vi "VC100_Facility_Control_V1.0.vi"() -> ()   [LabVIEW 2024]
uses:
  Small_Facility_Control/Current_Facility_State.ctl
  Small_Facility_Control/Facility_State.ctl
  <vilib>/Platform/TimedLoop/XDataNode/timing_clust.ctl
  <vilib>/Platform/TimedLoop/XDataNode/nitl_modes.ctl
  <vilib>/Platform/TimedLoop/XDataNode/wakeup.ctl
  <vilib>/DAQmx/read.llb/DAQmx Read (Analog Wfm 1Chan 1Samp).vi
  <vilib>/DAQmx/read.llb/DAQmx Read (Digital Bool 1Line 1Point).vi
  <vilib>/DAQmx/read.llb/DAQmx Read (Analog 1D Wfm NChan NSamp).vi
  <vilib>/DAQmx/read.llb/DAQmx Read (Digital 1D Bool NChan 1Samp 1Line).vi
  <vilib>/Analysis/baseanly.llb/Mean (DBL).vi
  92da63ed-27f3-4d29-b829-85232dab9436.vi
  dc02d6ae-0d69-4f83-ad2b-62eea8acb765.vi
  5e56a759-01b7-43ee-a6c9-aa4e2b3cae4c.vi
  a7228664-7861-4e48-9f8d-e2306638d1d9.vi
  <vilib>/DAQmx/write.llb/DAQmx Write (Digital 1D Bool NChan 1Samp 1Line).vi
  <vilib>/DAQmx/write.llb/DAQmx Write (Digital Bool 1Line 1Point).vi
  <instrlib>/U1250 Series Multimeter Device Driver/Public/Configure/Low Level/DC Voltage Configuration.vi
  <vilib>/DAQmx/create/channels.llb/DAQmx Create Channel (AI-Voltage-Basic).vi
  <vilib>/DAQmx/miscellaneous.llb/DAQmx Fill In Error Info.vi
  <vilib>/DAQmx/create/channels.llb/DAQmx Create Channel (DO-Digital Output).vi
  <vilib>/DAQmx/create/channels.llb/DAQmx Create Channel (DI-Digital Input).vi
  <vilib>/DAQmx/configure/timing.llb/DAQmx Timing (Sample Clock).vi
  <vilib>/express/express shared/transition.llb/Dynamic To Waveform Array.vi
  <vilib>/express/express signal manip/GetorSetDDTAttributes/Set DDT Attributes/SetT0.vi
  <vilib>/express/express signal manip/GetorSetDDTAttributes/Set DDT Attributes/sub Set StartTimeStamp.vi
  <vilib>/express/express shared/transition.llb/Waveform Array To Dynamic.vi
  <vilib>/Utility/file.llb/Write Delimited Spreadsheet (string).vi
  <instrlib>/U1250 Series Multimeter Device Driver/Controls/Voltage Range.ctl
  <vilib>/platform/TimedLoop/XDataNode/XDataNode.xnode
  <vilib>/express/express signal manip/GetorSetDDTAttributes/Set DDT Attributes/Set DDT Properties.xnode
  <vilib>/express/express signal manip/GetorSetDDTAttributes/Get DDT Attributes/Get DDT Properties.xnode
  <resource>/objmgr/daqmx.rc
  <instrlib>/U1250 Series Multimeter Device Driver/U1250 Series Digital Multimeter.lvlib
  <vilib>/express/express signal manip/GetorSetDDTAttributes/Set DDT Attributes/Set DDT Attributes.lvlib
  <vilib>/Platform/TimedLoop/XDataNode/XDNodeRunTimeDep.lvlib
  <vilib>/Analysis/NI_AALBase.lvlib
panel:
  out "Low Compressor Pressure!":bool
  out "Turbo on Threshold (torr) 3":dbl=0.08
  out "Compressor Pressure (Bar)":dbl=627.9033934565941 format="%_3f"
  in  "Turbo slowing Threshold (%)":dbl=50.0 format="%#_13g"
  out "Use Ecodry As Primary?":bool=TRUE
  out "Ecodry Speed":string="0"
  out "Turbo 2 Speed":string="0"
  out "Turbo 3 Standby?":bool
  out "Turbo 2 Standby?":bool
  out "Turbo 2 Motor Read":bool
  out "Turbo_2_Motor_Sys_Cmd":bool
  out "Numeric 3":dbl
  out "Numeric 2":dbl
  out "New_State? 2":bool
  out "appended array":string[][](array[string])
  out "New log 3":string
  out "New log 2":string
  out "output array":string[][](array[string])
  out "New log":string
  out "New_State?":bool
  out "Sub_state_iteration":i32
  out "DAQ_Name 2":string="cDAQ1"
  out "Turbo on Threshold (torr)":dbl=0.08
  out "Elapsed Time (s)":dbl
  in  "Turbo on Threshold (torr) 2":dbl=0.25 format="%#_13g"
  out "WRG (torr)":dbl=nan format="%_3e"
  in  "Turbo_Reset_Cmd":bool
  in  "Turbo_3_Motor_User_Cmd":bool
  in  "Turbo_2_Motor_User_Cmd":bool
  in  "Turbo_1_Motor_User_Cmd":bool
  in  "Chiller_User_Cmd":bool
  in  "Primary_User_Cmd":bool
  in  "Valve_Gate_3_User_Cmd":bool
  in  "Valve_Gate_2_User_Cmd":bool
  in  "Valve_Gate_1_User_Cmd":bool
  in  "Valve_Vent_User_Cmd":bool
  in  "Valve_Bypass_User_Cmd":bool
  in  "Valve_Turbo_3_User_Cmd":bool
  in  "Valve_Turbo_2_User_Cmd":bool
  out "Turbo 3 Valve Error?":bool
  out "Turbo 2 Valve Error?":bool
  out "Bypass Valve Error?":bool
  out "Gate 3 Valve Error?":bool
  out "Gate 2 Valve Error?":bool
  out "Gate 1 Valve Error?":bool
  in  "Valve_Turbo_1_User_Cmd":bool
  out "Turbo 1 Valve Error?":bool
  out "Index_of_working_turbo":i32
  out "Which_Turbos_used?":bool[](array[boolean])
  out "Valve_Gate_3_Sys_Cmd":bool
  out "Valve_Gate_2_Sys_Cmd":bool
  out "Valve_Turbo_3_Sys_Cmd":bool
  out "Valve_Turbo_2_Sys_Cmd":bool
  out "Turbo 3 Gauge":dbl=627.9033934565941 format="%_3e"
  out "Turbo 2 Gauge":dbl=627.9033934565941 format="%_3e"
  out "Turbo 3 Speed":string="0"
  out "Turbo 3 Status":string="Turbo Off"
  out "Turbo 2 Status":string="Turbo Off"
  out "Turbo 3 Status Color":u32(colorbox)=12632256
  out "Turbo 2 Status Color":u32(colorbox)=12632256
  out "Gate 3 Valve":bool
  out "Gate 2 Valve":bool
  out "Turbo 3 Valve":bool
  out "Turbo 2 Valve":bool
  in  "Change to Auto":bool
  out "Measurement":dbl format="%#_8f"
  in  "ON/OFF":bool
  in  "DMM VISA resource name COM4":refnum<visa-resource-name>="COM4"
  in  "use DMM?":bool
  in  "samples per channel":i32=200
  in  "rate":dbl=1000.0 format="%#_13g"
  out "Current Time/date":string
  out "String 3":string
  out "Vent Time (s) 2":dbl caption="Elapsed Time (s)"
  out "Numeric":dbl
  out "Turbo 1 Gauge":dbl=627.9033934565941 format="%_3e"
  out "Log":string
  out "Gate 1 Valve":bool
  out "Valve_Gate_1_Sys_Cmd":bool
  out "Vent Valve Error?":bool
  out "Primary Status":u32(colorbox)=12632256
  out "Bypass Valve":bool
  out "Vent Valve":bool
  out "Primary Pump Status":string="Primary Pump is Off"
  out "Wide Range Gauge Pressure":dbl=nan format="%_3e"
  out "Foreline Gauge":dbl=627.9033934565941 format="%_3e"
  out "Chiller Status":string="Chiller is Off"
  out "Turbo 1 Status":string="Turbo Off"
  out "Chiller Status 2":u32(colorbox)=12632256
  out "Turbo 1 Status Color":u32(colorbox)=12632256
  in  "stop":bool
  out "error out":errorcluster
  out "Control Level":enum32{"Admin", "Debug", "Automatic"}(tab)=enum."Automatic"
  in  "Fake_Chiller_Read":bool
  in  "Fake_Turbo_1_Pressure_mBar":dbl=0.0001 format="%_3e"
  in  "Fake_Primary_Pump_Read":bool
  in  "Fake_Valve_Turbo_Read":bool
  in  "Fake_Valve_Bypass_Read":bool
  in  "Fake_Valve_Vent_Read":bool
  in  "Use fake values?":bool=TRUE
  in  "Fake_Fore_Pressure_mBar":dbl=0.001 format="%_3e"
  in  "Fake_Valve_Gate_Read":bool
  in  "Fake_WRG_Pressure_mBar":dbl=1e-05 format="%_3e"
  in  "Turbo Engage time":timestamp=timestamp(3820287600 s since 1904-01-01)
  out "Current Facility State":T1
  out "Target Facility State":T1
  out "Tab Control":T2(tab)=enum."Holding at Rough"
  in  "Pump to High Vac":bool
  in  "Pump to Rough":bool
  in  "Overnight Pump":bool
  in  "Vent":bool
  in  "Shut Off once rough 2":bool
  in  "Vent 2":bool
  in  "Shut Off":bool
  in  "Overnight Pump 3":bool
  in  "Pump to Rough 2":bool
  in  "Pump to High Vac 2":bool
  in  "Shut Off once rough":bool
  in  "Vent 4":bool
  in  "Pump to Rough 3":bool
  in  "Pump to High Vac 3":bool
  in  "Vent 5":bool
  in  "Shutdown":bool
  in  "Pump to Rough 4":bool
  in  "Overnight Pump 2":bool
  in  "Vent and shutdonw":bool
  in  "Shutdown Now":bool
  in  "Pump to Hi vac":bool
  in  "Overnight Pump 5":bool
  in  "Pump to Rough 5":bool
  in  "Shutdown After Vent":bool
  in  "Pump to High Vac 4":bool
  in  "Vent":bool
  in  "change_to_admin_mode":bool
  out "Countdown":string
  in  "Clear error?":bool
  out "Running":bool
  out "Waveform Chart 2":waveform(dbl)[](graph)=[{"t0"=timestamp(3754409348.7178025 s since 1904-01-01), "dt"=0.1, "Y"=array[1789 elements]}, {"t0"=timestamp(3754409348.7178025 s since 1904-01-01), "dt"=0.1, "Y"=array[1789 elements]}, {"t0"=timestamp(3754409348.7178025 s since 1904-01-01), "dt"=0.1, "Y"=array[1789 elements]}, {"t0"=timestamp(3754409348.7178025 s since 1904-01-01), "dt"=0.1, "Y"=array[1789 elements]}, {"t0"=timestamp(3754409348.7178025 s since 1904-01-01), "dt"=0.1, "Y"=array[1789 elements]}, {"t0"=timestamp(3754409348.7178025 s since 1904-01-01), "dt"=0.1, "Y"=array[1789 elements]}, {"t0"=timestamp(3754409348.7178025 s since 1904-01-01), "dt"=0.1, "Y"=array[1789 elements]}, {"t0"=timestamp(3754409348.7178025 s since 1904-01-01), "dt"=0.1, "Y"=array[1789 elements]}]
  out "Turbo 3 Motor Read":bool
  out "Primary_Pump_Read":bool
  out "Turbo_3_Motor_Sys_Cmd":bool
  out "Chiller_Sys_Cmd":bool
  out "Valve_Vent_Sys_Cmd":bool
  out "Valve_Bypass_Sys_Cmd":bool
  out "Valve_Turbo_1_Sys_Cmd":bool
  out "Use_real_Values?":bool=TRUE
  out "Primary_Sys_Cmd":bool
  out "DAQ_Name":string="cDAQ1"
  out "Turbo 1 Valve":bool
  out "String 4":string
  # "mBar"
  # "Pressure (mBar)"
  # "Speed (%):"
  # "Speed (%):"
  # "mBar"
  # "mBar"
  # "mBar"
  # "On"
  # "Status"
  # "mBar"
  # "Off"
  # "Admin Mode Enabled"
  # "Please Wait..."
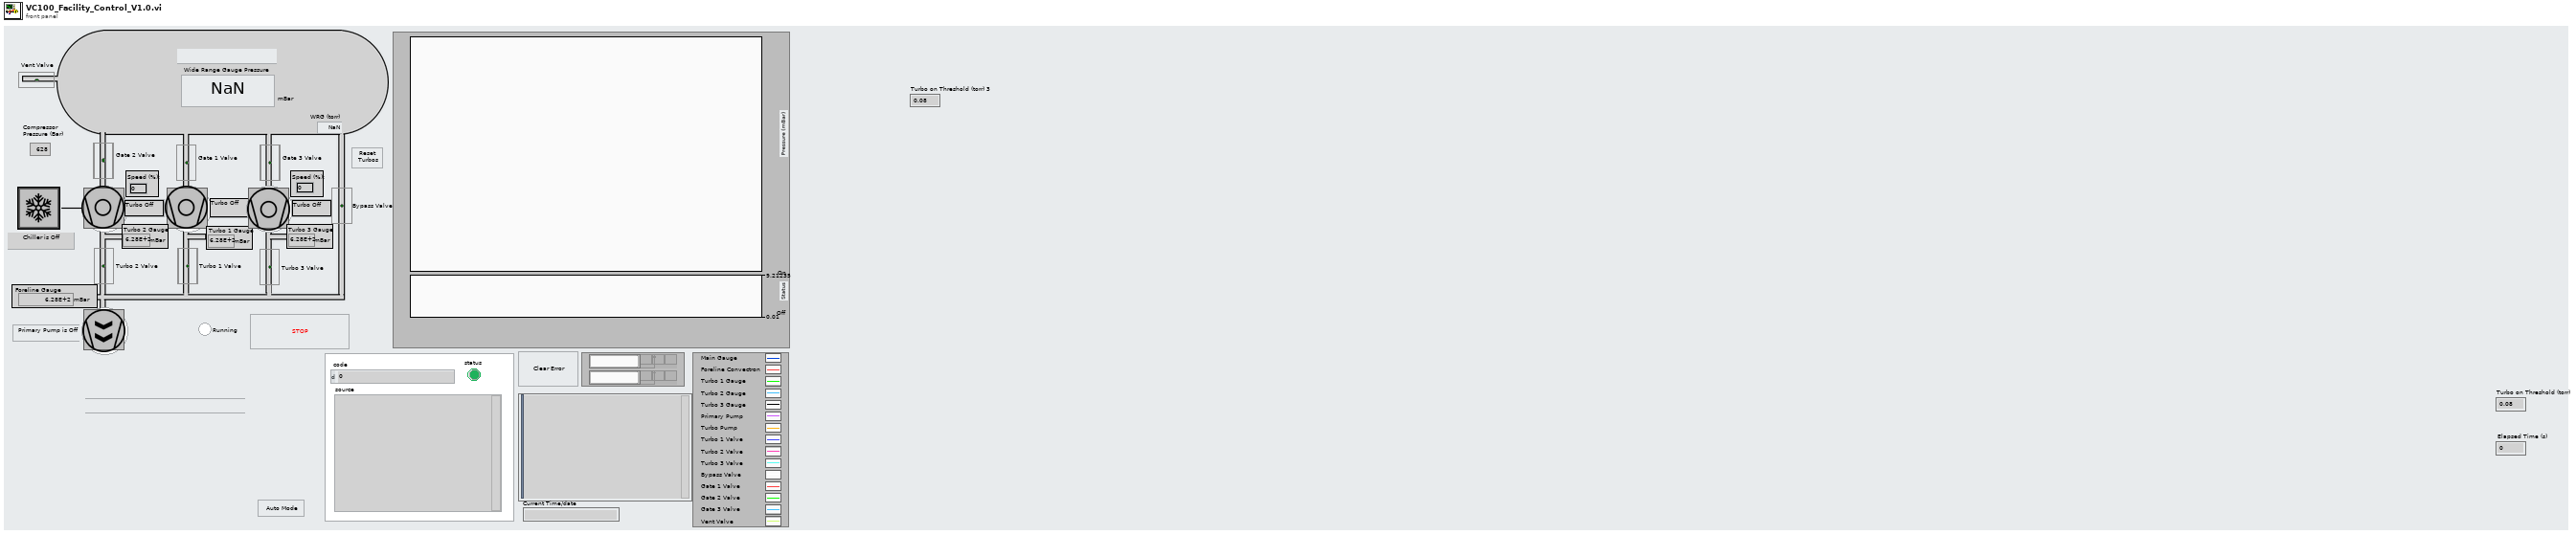
[diagram p1: front panel]
types:
  T1 = typedef "Current_Facility_State.ctl" = enum16{"Facility Off", "Pumping to Rough", "Overnight Pump", "Engage Turbo", "Pumping to High Vac", "Disengage Turbo", "Vent and Shutdown", "Turbo slowing", "Venting"}
  T2 = enum32{"Facility Off", "Pumping to Rough", "Holding at Rough", "Overnight Pump", "Engaging Turbo", "Pumping to Hig Vac", "Closing Gate", "Venting", "Turbo Slowing"}
  T3 = cluster{"Turbo Rotating Read":bool, "Turbo Accelarating Read":bool, "Turbo At Speed Read":bool, "Turbo Breaking Read":bool, "Turbo Alarm Read":bool, "Turbo Warning Read":bool, "Turbo Motor SYS CMD":bool, "Turbo Standby SYS CMD":bool, "Turbo Reset  SYS CMD":bool}
  T4 = typedef "Facility_State.ctl" = enum16{"Intialize", "Admin", "Manual", "Auto"}
  T5 = typedef "U1250 Series Digital Multimeter.lvlib/Voltage Range.ctl" = enum16{"5V", "50V", "500V", "1000V", "Auto"}
  T6 = typedef "XDNodeRunTimeDep.lvlib/timing_clust.ctl" = cluster{"Expected End [f-1]":u64, "Actual End [f-1]":u64, "Finished Late? [f-1]":bool, "Expected End [i-1]":u64, "Actual End [i-1]":u64, "Finished Late? [i-1]":bool, "Expected Start [i]":u64, "Actual Start [i]":u64, "Expected Start [f]":u64, "Actual Start [f]":u64, "Source Name":string, "Structure Name":string, "Period":i64, "Deadline":i64, "Offset":i64, "Start":i64, "Priority":i32, "Timeout":i32, "Mode":T7, "Wakeup Reason":T8, "Error":errorcluster, "Source Type":string, "Secondary Source Type":string, "Global End Time":u64, "Global Start Time":u64, "Frame Duration":u64, "Iteration Duration":u64, "Assigned CPU":i32, "I/O Scan Engine Mode":u32}
  T7 = typedef "XDNodeRunTimeDep.lvlib/nitl_modes.ctl" = enum32{"No Change", "Process missed periods, maintain original phase", "Discard missed periods, maintain original phase", "Process missed periods, ignore original phase", "Discard missed periods, ignore original phase"}
  T8 = typedef "XDNodeRunTimeDep.lvlib/wakeup.ctl" = enum32{"Normal", "Aborted", "Asynchronous wakeup", "Timing source error", "Timed loop error", "Timeout"}
  T9 = enum16{"open", "replace", "create", "open or create", "replace or create", "replace or create with confirmation"}
  T10 = enum16{"Off", "Spinning Up", "Speed Reached", "Spinning Down", "Turbo in Standby", "Turbo Warning", "Error"}
  T11 = enum16{"Off", "Spinning Up", "Speed Reached", "Spinning Down", "Turbo in Standby", "Error"}
  T12 = enum16{"Off", "Spinning Up", "Speed Reached", "Spinning Down", "Turbo In Standby", "Error"}
  T13 = cluster{"[0]":bool, "[1]":bool, "[2]":bool, "[3]":bool, "[4]":bool, "[5]":bool}
  T14 = enum16{"Left Button", "Center Button", "Right Button", "Window Close"}
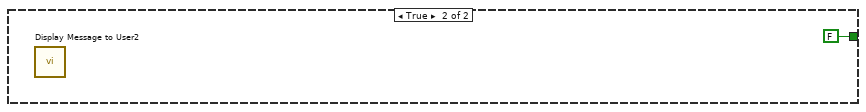
[diagram p2: hidden frame]
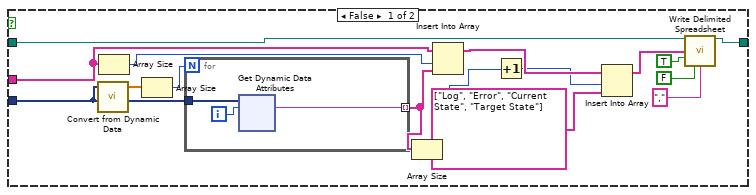
[diagram p3: hidden frame]
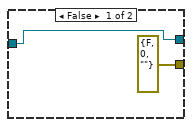
[diagram p4: hidden frame]
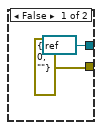
[diagram p6: hidden frame]
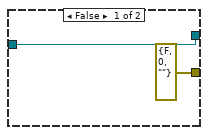
[diagram p7: hidden frame]
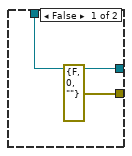
[diagram p8: hidden frame]
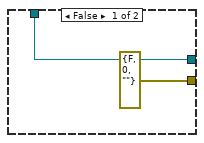
[diagram p9: hidden frame]
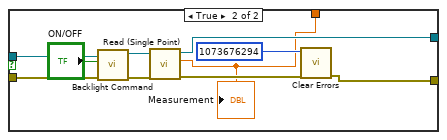
[diagram p10: hidden frame]
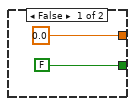
[diagram p11: hidden frame]
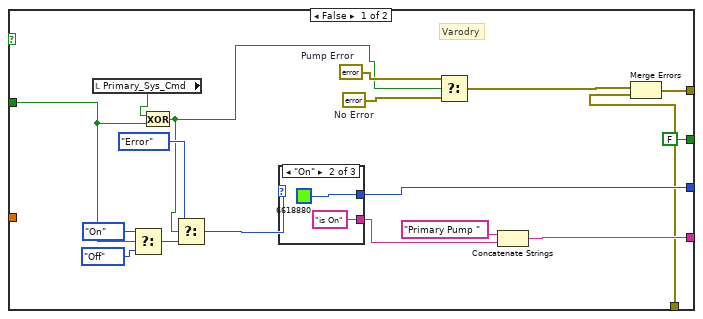
[diagram p12: hidden frame]
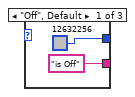
[diagram p13: hidden frame]
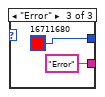
[diagram p14: hidden frame]
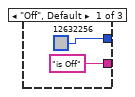
[diagram p15: hidden frame]
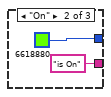
[diagram p16: hidden frame]
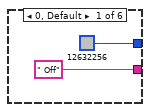
[diagram p17: hidden frame]
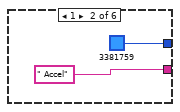
[diagram p18: hidden frame]
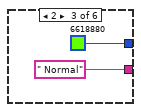
[diagram p19: hidden frame]
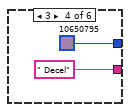
[diagram p20: hidden frame]
diagram:
  w13 = "Air_Com_pressure"  # channel name
  w11 = "Mod8/ai7"  # physical channel
  w24 = 10106 items=["default"=-1, "RSE"=10083, "NRSE"=10078, "Differential"=10106, "Pseudodifferential"=12529]  # input terminal configuration
  w30 = 10348 items=["Volts"=10348, "From Custom Scale"=10065]  # units
  w29 = "Turbo_2_Speed_Read"  # channel name
  w28 = -10.0  # minimum value
  w27 = 10.0  # maximum value
  w40 = "Turbo 2 Error read"  # channel name
  w20 = string[] ["Motor CMD", "Standby CMD", "Reset CMD"]
  w54 = T3 {"Turbo Rotating Read"=FALSE, "Turbo Accelarating Read"=FALSE, "Turbo At Speed Read"=FALSE, "Turbo Breaking Read"=FALSE, "Turbo Alarm Read"=FALSE, "Turbo Warning Read"=FALSE, "Turbo Motor SYS CMD"=FALSE, "Turbo Standby SYS CMD"=FALSE, "Turbo Reset  SYS CMD"=FALSE}  # Turbo 1 Cluseter
  w57 = "Turbo 3 Error read"  # channel name
  w78 = 10178 items=["Finite Samples"=10178, "Continuous Samples"=10123, "Hardware Timed Single Point"=12522]  # sample mode
  w77 = 25  # number of samples
  w76 = 1000.0  # rate
  w49 = 0 items=["one channel for each line", "one channel for all lines"]  # line grouping
  w84 = 10106 items=["default"=-1, "RSE"=10083, "NRSE"=10078, "Differential"=10106, "Pseudodifferential"=12529]  # input terminal configuration
  w85 = 10348 items=["Volts"=10348, "From Custom Scale"=10065]  # units
  w86 = "Turbo_3_Speed_Read"  # channel name
  w87 = -10.0  # minimum value
  w88 = 10.0  # maximum value
  w33 = 0 items=["one channel for each line", "one channel for all lines"]  # line grouping
  w80 = TRUE  # auto cleanup
  w112 = "Valve_Gate_3_Cmd"  # channel name
  w94 = "Valve_Gate_2_Cmd"  # channel name
  w97 = "Valve_Gate_1_Cmd"  # channel name
  w107 = 0 items=["one channel for each line", "one channel for all lines"]  # line grouping
  w100 = "Valve_Turbo_3_Cmd"  # channel name
  w117 = "Turbo_gauge_3_Read"  # channel name
  w115 = "Mod8/ai4"  # physical channel
  w118 = "Turbo_gauge_2_Read"  # channel name
  w129 = TRUE  # Turbo 3 in use?
  w124 = TRUE  # Turbo 2 in use?
  w127 = TRUE  # Turbo 1 in use?
  w152 = "Valve_Gate_3_Read"  # channel name
  w135 = "Valve_Gate_2_Read"  # channel name
  w138 = "Valve_Gate_1_Read"  # channel name
  w153 = 0 items=["one channel for each line", "one channel for all lines"]  # line grouping
  w141 = "Valve_Turbo_3_Read"  # channel name
  w157 = "cDAQ2Mod8/ai0"  # physical channel
  w165 = 10106 items=["Default"=-1, "RSE"=10083, "NRSE"=10078, "Differential"=10106, "Pseudodifferential"=12529] ("input terminal configuration")
  w166 = FALSE
  w173 = 4 items=["verify"=2, "reserve"=4, "commit"=3, "unreserve"=5, "abort"=6] ("action")
  w177 = 10178 items=["Finite Samples"=10178, "Continuous Samples"=10123, "Hardware Timed Single Point"=12522] ("sample mode")
  w182 = "Mod8/ai3"  # physical channel
  w47 = FALSE ("stop")
  w183 = 0  # Sub_state_iteration
  w184 = Current_Facility_State."Facility Off"  # Target Facility State
  w185 = Current_Facility_State."Facility Off"  # Current Facility State
  w189 = "Valve_Turbo_2_Read"  # channel name
  w195 = "Valve_Turbo_2_Cmd"  # channel name
  w201 = TRUE
  w202 = 5.0  # Sample Freq (Hz)
  w208 = FALSE  # invert line
  w23 = FALSE
  w130 = FALSE
  (unwired) Facility_State."Intialize"
  w241 = 0 items=["one channel for each line", "one channel for all lines"]  # line grouping
  w236 = "Chiller_Cmd"  # channel name
  w239 = TRUE  # auto cleanup
  w249 = 0 items=["one channel for each line", "one channel for all lines"]  # line grouping
  w248 = "Chiller_Read"  # channel name
  w251 = TRUE  # auto cleanup
  w280 = "Turbo_gauge_1_Read"  # channel name
  w265 = "Mod8/ai2"  # physical channel
  w278 = "Foreline_gauge_1_Read"  # channel name
  w266 = "Mod8/ai1"  # physical channel
  w5 = 10106 items=["default"=-1, "RSE"=10083, "NRSE"=10078, "Differential"=10106, "Pseudodifferential"=12529]  # input terminal configuration
  w1 = 10348 items=["Volts"=10348, "From Custom Scale"=10065]  # units
  w275 = "Wide Range_Gauge_Read"  # channel name
  w6 = 0.0  # minimum value
  w7 = 10.0  # maximum value
  w269 = "Mod8/ai0"  # physical channel
  w272 = TRUE  # auto cleanup
  w311 = "Valve_Turbo_1_Cmd"  # channel name
  w308 = "Valve_Vent_Cmd"  # channel name
  w270 = 0 items=["one channel for each line", "one channel for all lines"]  # line grouping
  w305 = "Valve_Bypass_Cmd"  # channel name
  w303 = TRUE  # auto cleanup
  w332 = "Valve_Turbo_1_Read"  # channel name
  w329 = "Valve_Vent_Read"  # channel name
  w188 = 0 items=["one channel for each line", "one channel for all lines"]  # line grouping
  w326 = "Valve_Bypass_Read"  # channel name
  w324 = TRUE  # auto cleanup
  w333 = FALSE  # auto cleanup
  w346 = 0 items=["one channel for each line", "one channel for all lines"]  # line grouping
  w205 = "Primary_Pump_Read"  # channel name
  w344 = TRUE  # auto cleanup
  w41 = "cDAQ3"
  # "Turbo 3 Digital CMD"
  # "Turbo 2  Speed Read"
  # "Saving Data"
  # "Turbo 2 Digital CMD"
  # "Turbo 1 Digital CMD"
  # "Turbo 2 Digital Read"
  # "Turbo 1 Digital Read"
  # "Turbo 3  Speed Read"
  # "Turbo 3 Digital Read"
  # "Force Stop on exit?"
  # "Init Chiller Cmd"
  # "Init Chiller Read"
  # "Init Gauge Read"
  # "Init Primary Pump Cmd"
  # "Init Valve Cmd"
  # "Init Valve Read"
  # "Init Primary Pump Read"
  n1 = call <vilib>:"DAQmx Create Task.vi"("auto cleanup"=FALSE) -> ("task out"=w51:refnum<k21>, "error out"=w50:errorcluster)  [unwired: 13 in]
  n2 = Select(t=1, s=w124, f=2) -> (s? t:f=w125:i32)
  n3 = Build Array(w127, w124, w129) -> (→"Which_Turbos_used?":bool[])
  n4 = local write "Valve_Turbo_3_Sys_Cmd"(w47) -> ()
  n5 = local write "Turbo_3_Motor_Sys_Cmd"(w47) -> ()
  n6 = local write "Valve_Gate_1_Sys_Cmd"(w47) -> ()
  n7 = local write "Valve_Gate_2_Sys_Cmd"(w47) -> ()
  n8 = local write "Valve_Turbo_1_Sys_Cmd"(w47) -> ()
  n9 = local write "Valve_Turbo_2_Sys_Cmd"(w47) -> ()
  n10 = property on="Countdown" class="Str"("Visible"=w47) -> ()  [unwired: 2 in, 2 out]
  n11 = local write "Valve_Turbo_3_Sys_Cmd"(w47) -> ()
  n12 = local write "Primary_Sys_Cmd"(w47) -> ()
  n13 = local write "Chiller_Sys_Cmd"(w47) -> ()
  n14 = local write "Valve_Bypass_Sys_Cmd"(w47) -> ()
  n15 = local write "Valve_Vent_Sys_Cmd"(w47) -> ()
  n16 = Select(t=0, s=w127, f=w125) -> (s? t:f=→"Index_of_working_turbo":i32)
  n17 = local write "New_State?"(TRUE ("New_State?")) -> ()
  n18 = local write "DAQ_Name"(w41) -> ()
  n19 = local write "Tab Control"(T2."Holding at Rough" ("Tab Control")) -> ()
  n20 = local write "stop"(FALSE ("stop")) -> ()
  n21 = local read "DAQ_Name"() -> (w15:string)
  n22 = for {
    shift-right: [w364] -> w52
    shift-left: w51 -> [w365]
    shift-right: [w363] -> w53
    shift-left: w50 -> [w366]
    tunnel: w15 -> [w362]
    tunnel: w20 -> [w355] mode=indexing
    tunnel: w49 -> [w352]
    i -> [w360]
    n23 = Concatenate Strings("Turbo 1 " ("string"), w355) -> (w353:string)
    n24 = Add(x=0, y=w360) -> (x+y=w358:i32)
    n25 = Number To Decimal String(number=w358) -> (decimal integer string=w357:string)  [unwired: 1 in]
    n26 = Concatenate Strings(w362, "Mod3/port0/line" ("lines"), w357) -> (w361:string)
    n27 = call-poly <vilib>:"DAQmx Create Virtual Channel.vi"("task in"=w365, "lines"=w361, "name to assign"=w353, "line grouping"=w352, "error in"=w366) -> ("task out"=w364:refnum<k21>, "error out"=w363:errorcluster)  [unwired: 9 in]
  }
  n28 = local write "Use_real_Values?"("Use fake values?") -> ()
  n29 = call <vilib>:"DAQmx Create Task.vi"("auto cleanup"=w80) -> ("task out"=w55:refnum<k21>, "error out"=w62:errorcluster)  [unwired: 13 in]
  n30 = call <vilib>:"Clear Errors.vi"() -> ("error out"=w215:errorcluster)  [unwired: 6 in, 1 out]
  n31 = for {
    shift-right: [w379] -> w37
    shift-left: w55 -> [w380]
    shift-right: [w378] -> w36
    shift-left: w62 -> [w381]
    tunnel: w15 -> [w377]
    tunnel: string[] ["Rotating", "Accelerating", "At Speed", "Breaking", "Alarm", "Warning"] -> [w370] mode=indexing
    tunnel: w33 -> [w367]
    i -> [w375]
    n32 = Concatenate Strings("Turbo 1 " ("string"), w370) -> (w368:string)
    n33 = Add(x=10, y=w375) -> (x+y=w373:i32)
    n34 = Number To Decimal String(number=w373) -> (decimal integer string=w372:string)  [unwired: 1 in]
    n35 = Concatenate Strings(w377, "Mod2/port0/line" ("lines"), w372) -> (w376:string)
    n36 = call-poly <vilib>:"DAQmx Create Virtual Channel.vi"("task in"=w380, "lines"=w376, "name to assign"=w368, "line grouping"=w367, "error in"=w381) -> ("task out"=w379:refnum<k21>, "error out"=w378:errorcluster)  [unwired: 9 in]
  }
  n37 = call <vilib>:"DAQmx Create Task.vi"("auto cleanup"=w272) -> ("task out"=w273:refnum<k21>, "error out"=w271:errorcluster)  [unwired: 13 in]
  n38 = local read "DAQ_Name"() -> (w4:string)
  n39 = case shown="True" w166 {
    tunnel: [refnum<visa-resource-name> refnum ("VISA resource name out") w386] -> w170
    tunnel: [errorcluster {"status"=FALSE, "code"=0, "source"=""} ("error out") w385] -> w169
    frame False {
    }
    frame True {
      n40 = call <instrlib>:"Initialize.vi"("Reset (True)"=TRUE, "ID Query (True)"=TRUE, "VISA resource name"="DMM VISA resource name COM4") -> ("error out"=w392:errorcluster, "VISA resource name out"=w394:refnum<visa-resource-name>)  [unwired: 7 in]
      n41 = call-poly <instrlib>:"Measurement Configuration.vi"("error in (no error)"=w392, "Voltage Range"=Voltage_Range."50V", "VISA resource name"=w394) -> ("error out"=w389:errorcluster, "VISA resource name out"=w390:refnum<visa-resource-name>)  [unwired: 7 in]
      n42 = call <instrlib>:"Backlight Command.vi"("error in (no error)"=w389, "ON/OFF"=TRUE, "VISA resource name"=w390) -> ("error out"=w385:errorcluster, "VISA resource name out"=w386:refnum<visa-resource-name>)  [unwired: 7 in]
    }
  }
  n43 = call <vilib>:"DAQmx Create Task.vi"("auto cleanup"=w303) -> ("task out"=w304:refnum<k21>, "error out"=w302:errorcluster)  [unwired: 13 in]
  n44 = call <vilib>:"DAQmx Create Task.vi"("auto cleanup"=w324, "error in"=w215) -> ("task out"=w325:refnum<k21>, "error out"=w323:errorcluster)  [unwired: 12 in]
  n45 = local read "DAQ_Name"() -> (w187:string)
  n46 = local read "DAQ_Name"() -> (w154:string)
  n47 = Concatenate Strings(w4, w269) -> (w268:string)
  n48 = for {
    shift-right: [w407] -> w22
    shift-left: w52 -> [w408]
    shift-right: [w406] -> w21
    shift-left: w53 -> [w409]
    tunnel: w15 -> [w405]
    tunnel: w49 -> [w396]
    tunnel: w20 -> [w395] mode=indexing
    i -> [w403]
    n49 = Concatenate Strings("Turbo 2 " ("string"), w395) -> (w397:string)
    n50 = Add(x=3, y=w403) -> (x+y=w401:i32)
    n51 = Number To Decimal String(number=w401) -> (decimal integer string=w400:string)  [unwired: 1 in]
    n52 = Concatenate Strings(w405, "Mod3/port0/line" ("lines"), w400) -> (w404:string)
    n53 = call-poly <vilib>:"DAQmx Create Virtual Channel.vi"("task in"=w408, "lines"=w404, "name to assign"=w397, "line grouping"=w396, "error in"=w409) -> ("task out"=w407:refnum<k21>, "error out"=w406:errorcluster)  [unwired: 9 in]
  }
  n54 = local read "DAQ_Name"() -> (w197:string)
  n55 = local read "DAQ_Name"() -> (w111:string)
  n56 = call-poly <vilib>:"DAQmx Create Virtual Channel.vi"("task in"=w273, "maximum value"=w7, "minimum value"=w6, "input terminal configuration"=w5, "physical channels"=w268, "name to assign"=w275, "units"=w1, "error in"=w271) -> ("task out"=w276:refnum<k21>, "error out"=w274:errorcluster)  [unwired: 6 in]
  n57 = Concatenate Strings(w15, "Mod8/ai5" ("physical channel")) -> (w32:string)
  n58 = Concatenate Strings(w197, "Mod1/port0/line0" ("lines")) -> (w295:string)
  n59 = Concatenate Strings(w111, "Mod1/port0/line4" ("lines")) -> (w105:string)
  n60 = Concatenate Strings(w187, "Mod2/port0/line0" ("lines")) -> (w321:string)
  n61 = Concatenate Strings(w154, "Mod2/port0/line4" ("lines")) -> (w143:string)
  n62 = call-poly <vilib>:"DAQmx Create Virtual Channel.vi"("task in"=w325, "lines"=w321, "name to assign"=w326, "line grouping"=w188, "error in"=w323) -> ("task out"=w328:refnum<k21>, "error out"=w327:errorcluster)  [unwired: 9 in]
  n63 = call-poly <vilib>:"DAQmx Create Virtual Channel.vi"("task in"=w304, "lines"=w295, "name to assign"=w305, "line grouping"=w270, "error in"=w302) -> ("task out"=w307:refnum<k21>, "error out"=w306:errorcluster)  [unwired: 9 in]
  n64 = Concatenate Strings(w4, w266) -> (w267:string)
  n65 = call-poly <vilib>:"DAQmx Create Virtual Channel.vi"("task in"=w276, "maximum value"=w7, "minimum value"=w6, "input terminal configuration"=w5, "physical channels"=w267, "name to assign"=w278, "units"=w1, "error in"=w274) -> ("task out"=w279:refnum<k21>, "error out"=w277:errorcluster)  [unwired: 6 in]
  n66 = Concatenate Strings(w15, "Mod2/port0/line16" ("lines")) -> (w39:string)
  n67 = call-poly <vilib>:"DAQmx Create Virtual Channel.vi"("task in"=w37, "lines"=w39, "name to assign"=w40, "line grouping"=w33, "error in"=w36) -> ("task out"=w34:refnum<k21>, "error out"=w35:errorcluster)  [unwired: 9 in]
  n68 = Concatenate Strings(w187, "Mod2/port0/line1" ("lines")) -> (w318:string)
  n69 = Concatenate Strings(w154, "Mod2/port0/line5" ("lines")) -> (w146:string)
  n70 = Concatenate Strings(w197, "Mod1/port0/line1" ("lines")) -> (w297:string)
  n71 = Concatenate Strings(w111, "Mod1/port0/line5" ("lines")) -> (w103:string)
  n72 = call-poly <vilib>:"DAQmx Create Virtual Channel.vi"("task in"=w328, "lines"=w318, "name to assign"=w329, "line grouping"=w188, "error in"=w327) -> ("task out"=w331:refnum<k21>, "error out"=w330:errorcluster)  [unwired: 9 in]
  n73 = for {
    N: 2 -> [_]
    shift-right: [w421] -> w18
    shift-left: w22 -> [w422]
    shift-right: [w420] -> w19
    shift-left: w21 -> [w423]
    tunnel: string[] ["Motor CMD", "Standby CMD"] -> [w411] mode=indexing
    tunnel: w15 -> [w410]
    i -> [w418]
    n74 = Concatenate Strings("Turbo 3 " ("string"), w411) -> (w412:string)
    n75 = Add(x=6, y=w418) -> (x+y=w416:i32)
    n76 = Number To Decimal String(number=w416) -> (decimal integer string=w415:string)  [unwired: 1 in]
    n77 = Concatenate Strings(w410, "Mod3/port0/line" ("lines"), w415) -> (w419:string)
    n78 = call-poly <vilib>:"DAQmx Create Virtual Channel.vi"("task in"=w422, "lines"=w419, "name to assign"=w412, "error in"=w423) -> ("task out"=w421:refnum<k21>, "error out"=w420:errorcluster)  [unwired: 10 in]
  }
  n79 = call-poly <vilib>:"DAQmx Create Virtual Channel.vi"("task in"=w307, "lines"=w297, "name to assign"=w308, "line grouping"=w270, "error in"=w306) -> ("task out"=w310:refnum<k21>, "error out"=w309:errorcluster)  [unwired: 9 in]
  n80 = Concatenate Strings(w4, w265) -> (w264:string)
  n81 = Concatenate Strings(w15, "Mod8/ai6" ("physical channel")) -> (w82:string)
  n82 = call-poly <vilib>:"DAQmx Create Virtual Channel.vi"("task in"=w279, "maximum value"=w7, "minimum value"=w6, "input terminal configuration"=w5, "physical channels"=w264, "name to assign"=w280, "units"=w1, "error in"=w277) -> ("task out"=w181:refnum<k21>, "error out"=w179:errorcluster)  [unwired: 6 in]
  n83 = Concatenate Strings(w15, "Mod2/port0/line17" ("lines")) -> (w59:string)
  n84 = call-poly <vilib>:"DAQmx Create Virtual Channel.vi"("task in"=w34, "lines"=w59, "name to assign"=w57, "line grouping"=w33, "error in"=w35) -> ("task out"=w58:refnum<k21>, "error out"=w56:errorcluster)  [unwired: 9 in]
  n85 = Concatenate Strings(w187, "Mod2/port0/line2" ("lines")) -> (w317:string)
  n86 = Concatenate Strings(w154, "Mod2/port0/line6" ("lines")) -> (w147:string)
  n87 = Concatenate Strings(w197, "Mod1/port0/line2" ("lines")) -> (w298:string)
  n88 = Concatenate Strings(w111, "Mod1/port0/line6" ("lines")) -> (w102:string)
  n89 = call <vilib>:"DAQmx Create Task.vi"("auto cleanup"=w344) -> ("task out"=w345:refnum<k21>, "error out"=w343:errorcluster)  [unwired: 13 in]
  n90 = call <vilib>:"DAQmx Create Task.vi"("auto cleanup"=w251) -> ("task out"=w250:refnum<k21>, "error out"=w252:errorcluster)  [unwired: 13 in]
  n91 = call-poly <vilib>:"DAQmx Create Virtual Channel.vi"("task in"=w331, "lines"=w317, "name to assign"=w332, "line grouping"=w188, "error in"=w330) -> ("task out"=w192:refnum<k21>, "error out"=w191:errorcluster)  [unwired: 9 in]
  n92 = call <vilib>:"DAQmx Create Task.vi"("auto cleanup"=w239) -> ("task out"=w240:refnum<k21>, "error out"=w238:errorcluster)  [unwired: 13 in]
  n93 = call-poly <vilib>:"DAQmx Create Virtual Channel.vi"("task in"=w310, "lines"=w298, "name to assign"=w311, "line grouping"=w270, "error in"=w309) -> ("task out"=w199:refnum<k21>, "error out"=w198:errorcluster)  [unwired: 9 in]
  n94 = call <vilib>:"DAQmx Create Task.vi"("auto cleanup"=w333) -> ("task out"=w335:refnum<k21>, "error out"=w334:errorcluster)  [unwired: 13 in]
  n95 = Concatenate Strings(w4, w182) -> (w180:string)
  n96 = call-poly <vilib>:"DAQmx Create Virtual Channel.vi"("task in"=w181, "maximum value"=w7, "minimum value"=w6, "input terminal configuration"=w5, "physical channels"=w180, "name to assign"=w118, "units"=w1, "error in"=w179) -> ("task out"=w114:refnum<k21>, "error out"=w113:errorcluster)  [unwired: 6 in]
  n97 = local read "DAQ_Name"() -> (w233:string)
  n98 = local read "DAQ_Name"() -> (w253:string)
  n99 = Concatenate Strings(w197, "Mod1/port0/line3" ("lines")) -> (w196:string)
  n100 = Concatenate Strings(w111, "Mod1/port0/line7" ("lines")) -> (w89:string)
  n101 = local read "DAQ_Name"() -> (w351:string)
  n102 = Concatenate Strings(w187, "Mod2/port0/line3" ("lines")) -> (w190:string)
  n103 = Concatenate Strings(w154, "Mod2/port0/line7" ("lines")) -> (w151:string)
  n104 = local read "DAQ_Name"() -> (w342:string)
  n105 = call-poly <vilib>:"DAQmx Create Virtual Channel.vi"("task in"=w199, "lines"=w196, "name to assign"=w195, "error in"=w198) -> ("task out"=w93:refnum<k21>, "error out"=w92:errorcluster)  [unwired: 10 in]
  n106 = call-poly <vilib>:"DAQmx Create Virtual Channel.vi"("task in"=w93, "lines"=w105, "name to assign"=w100, "line grouping"=w107, "error in"=w92) -> ("task out"=w98:refnum<k21>, "error out"=w99:errorcluster)  [unwired: 9 in]
  n107 = call-poly <vilib>:"DAQmx Create Virtual Channel.vi"("task in"=w98, "lines"=w103, "name to assign"=w97, "line grouping"=w107, "error in"=w99) -> ("task out"=w95:refnum<k21>, "error out"=w96:errorcluster)  [unwired: 9 in]
  n108 = call-poly <vilib>:"DAQmx Create Virtual Channel.vi"("task in"=w95, "lines"=w102, "name to assign"=w94, "line grouping"=w107, "error in"=w96) -> ("task out"=w109:refnum<k21>, "error out"=w110:errorcluster)  [unwired: 9 in]
  n109 = call-poly <vilib>:"DAQmx Create Virtual Channel.vi"("task in"=w109, "lines"=w89, "name to assign"=w112, "error in"=w110) -> ("task out"=w91:refnum<k21>, "error out"=w90:errorcluster)  [unwired: 10 in]
  n110 = Concatenate Strings(w233, "Mod4/port0/line1" ("lines")) -> (w234:string)
  n111 = call-poly <vilib>:"DAQmx Create Virtual Channel.vi"("task in"=w192, "lines"=w190, "name to assign"=w189, "line grouping"=w188, "error in"=w191) -> ("task out"=w133:refnum<k21>, "error out"=w134:errorcluster)  [unwired: 9 in]
  n112 = call-poly <vilib>:"DAQmx Create Virtual Channel.vi"("task in"=w133, "lines"=w143, "name to assign"=w141, "line grouping"=w153, "error in"=w134) -> ("task out"=w139:refnum<k21>, "error out"=w140:errorcluster)  [unwired: 9 in]
  n113 = call-poly <vilib>:"DAQmx Create Virtual Channel.vi"("task in"=w139, "lines"=w146, "name to assign"=w138, "line grouping"=w153, "error in"=w140) -> ("task out"=w136:refnum<k21>, "error out"=w137:errorcluster)  [unwired: 9 in]
  n114 = call-poly <vilib>:"DAQmx Create Virtual Channel.vi"("task in"=w136, "lines"=w147, "name to assign"=w135, "line grouping"=w153, "error in"=w137) -> ("task out"=w149:refnum<k21>, "error out"=w150:errorcluster)  [unwired: 9 in]
  n115 = call-poly <vilib>:"DAQmx Create Virtual Channel.vi"("task in"=w149, "lines"=w151, "name to assign"=w152, "line grouping"=w153, "error in"=w150) -> ("task out"=w131:refnum<k21>, "error out"=w132:errorcluster)  [unwired: 9 in]
  n116 = Concatenate Strings(w253, "Mod2/port0/line9" ("lines")) -> (w255:string)
  n117 = Concatenate Strings(w351, "Mod4/port0/line0" ("lines")) -> (w349:string)
  n118 = Concatenate Strings(w4, w115) -> (w116:string)
  n119 = Concatenate Strings(w342, "Mod2/port0/line8" ("lines")) -> (w340:string)
  n120 = call-poly <vilib>:"DAQmx Create Virtual Channel.vi"("task in"=w114, "maximum value"=w7, "minimum value"=w6, "input terminal configuration"=w5, "physical channels"=w116, "name to assign"=w117, "units"=w1, "error in"=w113) -> ("task out"=w10:refnum<k21>, "error out"=w8:errorcluster)  [unwired: 6 in]
  n121 = call-poly <vilib>:"DAQmx Create Virtual Channel.vi"("task in"=w345, "lines"=w340, "name to assign"=w205, "line grouping"=w346, "error in"=w343) -> ("task out"=w207:refnum<k21>, "error out"=w301:errorcluster)  [unwired: 9 in]
  n122 = property class="DAQmx Channel"(reference=w207, "Active Channels (if subset)"=w205, "Digital Input:Invert Lines"=w208) -> (reference out=w206:refnum<k21>)  [unwired: 1 in, 1 out]
  n123 = call-poly <vilib>:"DAQmx Create Virtual Channel.vi"("task in"=w250, "lines"=w255, "name to assign"=w248, "line grouping"=w249, "error in"=w252) -> ("task out"=w247:refnum<k21>, "error out"=w232:errorcluster)  [unwired: 9 in]
  n124 = call-poly <vilib>:"DAQmx Create Virtual Channel.vi"("task in"=w335, "lines"=w349, "name to assign"="Primary_Pump_Cmd", "error in"=w334) -> ("task out"=w348:refnum<k21>, "error out"=w263:errorcluster)  [unwired: 10 in]
  n125 = call-poly <vilib>:"DAQmx Create Virtual Channel.vi"("task in"=w240, "lines"=w234, "name to assign"=w236, "line grouping"=w241, "error in"=w238) -> ("task out"=w237:refnum<k21>, "error out"=w230:errorcluster)  [unwired: 9 in]
  n126 = Concatenate Strings(w4, w11) -> (w12:string)
  n127 = call-poly <vilib>:"DAQmx Create Virtual Channel.vi"("task in"=w10, "maximum value"=w7, "minimum value"=w6, "input terminal configuration"=w5, "physical channels"=w12, "name to assign"=w13, "units"=w1, "error in"=w8) -> ("task out"=w9:refnum<k21>)  [unwired: 6 in, 1 out]
  n128 = Merge Errors(w19) -> (w75:errorcluster)
  n129 = call-poly <vilib>:"DAQmx Timing.vi"("task/channels in"=w9, "sample mode"=w177, "samples per channel"=25, "rate"=1000.0) -> ("task out"=w174:refnum<k21>, "error out"=w172:errorcluster)  [unwired: 10 in]
  n130 = call <vilib>:"DAQmx Control Task.vi"("task/channels in"=w174, "action"=w173, "error in"=w172) -> ("task out"=w26:refnum<k21>, "error out"=w171:errorcluster)  [unwired: 11 in]
  n131 = call-poly <vilib>:"DAQmx Create Virtual Channel.vi"("task in"=w26, "maximum value"=w27, "minimum value"=w28, "input terminal configuration"=w24, "physical channels"=w32, "name to assign"=w29, "units"=w30) -> ("task out"=w25:refnum<k21>)  [unwired: 7 in, 1 out]
  n132 = call-poly <vilib>:"DAQmx Create Virtual Channel.vi"("task in"=w25, "maximum value"=w88, "minimum value"=w87, "input terminal configuration"=w84, "physical channels"=w82, "name to assign"=w86, "units"=w85) -> ("task out"=w3:refnum<k21>, "error out"=w2:errorcluster)  [unwired: 7 in]
  n133 = call-poly <vilib>:"DAQmx Timing.vi"("task/channels in"=w3, "sample mode"=w78, "samples per channel"=w77, "rate"=w76, "error in"=w2) -> ("task out"=w158:refnum<k21>, "error out"=w74:errorcluster)  [unwired: 9 in]
  n134 = Merge Errors(w74, w75) -> (w81:errorcluster)
  n135 = Merge Errors(w56, w81) -> (w227:errorcluster)
  n136 = Merge Errors(w90, w301) -> (w300:errorcluster)
  n137 = Merge Errors(w132, w300) -> (w339:errorcluster)
  n138 = Merge Errors(w227) -> (w228:errorcluster)
  n139 = Merge Errors(w230, w228) -> (w229:errorcluster)
  n140 = Merge Errors(w232, w229) -> (w231:errorcluster)
  n141 = node-c288(i64 1000 ("Period")) -> (w46:T6)  [unwired: 3 in]
  n142 = call-poly <vilib>:"DAQmx Create Virtual Channel.vi"("input terminal configuration"=w165, "physical channels"=w157, "name to assign"="Dummy Variable to get nice time data") -> ("task out"=w156:refnum<k21>, "error out"=w155:errorcluster)  [unwired: 11 in]
  n143 = timed-loop {
    timing: w46 -> [_]
    timing-out: [_] -> w45
    stop <- w429 stop-if-true
    # "Check if file is open"
    n144 = node-c288() -> ()  [unwired: 1 in, 1 out]
    n145 = local read "Waveform Chart 2"() -> (w428:waveform(dbl)[])
    n146 = for {
      tunnel: w428 -> [w473] mode=indexing
      shift-right: [w466] -> w427
      shift-left: _ -> [w472]
      tunnel: string[] ["Wide Range Guage (mBar)", "Foreline Gauge (mBar)", "Turbo 1 Gauge (mBar)", "Turbo 2 Gauge (mBar)", "Turbo 3 Gauge (mBar)", "Primary Pump Status", "Turbo 3 Motor Read", "Turbo 1 Valve status", "Turbo 2 Valve status", "Turbo 3 Valve status", "Bypass Valve Status", "Gate 1 Valve Status", "Gate 2 Valve Status", "Gate 3 Valve Status", "Vant Valve"] -> [w460] mode=indexing
      i -> [w464]
      w459 = 0 ("Signal Index")
      n147 = Equal?(x=0, y=w464) -> (x = y?=w462:bool)
      n148 = Unbundle By Name(w473) -> ("Y"=w470:dbl[])  [unwired: 2 out]
      n149 = Array Size(array=w470) -> (size(s)=w468:i32)
      n150 = Decrement(x=w468) -> (x-1=w469:i32)
      n151 = Index Array(array=w470, index=w469) -> (element=w461:dbl)
      n152 = xnode ("Set Dynamic Data Attributes")("Signals In"=w461, "Signal Index"=w459, "Signal Name"=w460) -> ("Signals Out"=w465:dynamicdata)  [unwired: 4 in, 1 out]
      n153 = xnode ("Set Dynamic Data Attributes")("Signals In"=w461, "Signal Index"=w459, "Signal Name"=w460) -> ("Signals Out"=w471:dynamicdata)  [unwired: 4 in, 1 out]
      n154 = Merge Signals(w471, w472) -> (w467:dynamicdata)
      n155 = Select(t=w465, s=w462, f=w467) -> (s? t:f=w466:dynamicdata)
    }
    n156 = Get Date/Time String(date format (0)=enum16{"short", "long", "abbreviated"}."short") -> (date string=w434:string)  [unwired: 2 in, 1 out]
    n157 = Search and Replace String(replace all?=TRUE ("replace all? (F)"), input string=w434, search string="/", replace string="." ("replace string (\"\")")) -> (result string=w431:string)  [unwired: 4 in, 3 out]
    n158 = Concatenate Strings(w431, ".csv" ("string")) -> (w437:string)
    n159 = Build Path(base path=path "C:/Users/Lab Admin/Desktop/Pressure_Data", name or relative path=w437) -> (appended path=w436:path)
    n160 = call <vilib>:"Check if File or Folder Exists.vi"("path"=w436) -> ("file or folder exists?"=w456:bool)  [unwired: 8 in, 2 out]
    n161 = Build Array("Timestamp" ("new element/subarray")) -> (w447:string[])
    n162 = case shown="True" w456 {
      tunnel: w436 -> [w573 w588]
      tunnel: [w575 w588] -> w445
      tunnel: w427 -> [w570 _]
      tunnel: w447 -> [w567 _]
      frame False {
        n163 = call "Convert from Dynamic Data"("Dynamic Data Type"=w570) -> ("Array"=w568:dbl[])  [unwired: 3 in]
        n164 = Array Size(array=w567) -> (size(s)=w563:i32)
        n165 = Array Size(array=w568) -> (size(s)=w569:i32)
        n166 = for {
          N: w569 -> [_]
          tunnel: w570 -> [w578]
          tunnel: [w577] -> w561 mode=indexing
          i -> [w576]
          n167 = xnode "Get Dynamic Data Attributes"("Signals In"=w578, "Signal Index"=w576) -> ("Signal Name"=w577:string)  [unwired: 1 in, 2 out]
        }
        n168 = Array Size(array=w561) -> (size(s)=w560:i32)
        n169 = Insert Into Array(array=w567, index=w563, new element=w561) -> (w566:string[])
        n170 = Increment(x=w560) -> (x+1=w562:i32)
        n171 = Insert Into Array(array=w566, index=w562, new element=string[] ["Log", "Error", "Current State", "Target State"]) -> (w564:string[])
        n172 = call-poly <vilib>:"Write Delimited Spreadsheet.vi"("file path (dialog if empty)"=w573, "1D data"=w564, "append to file? (new file:F)"=TRUE, "transpose? (no:F)"=FALSE, "delimiter (\\t)"="," ("delimiter (\\t)")) -> ("new file path (Not A Path if cancelled)"=w575:path)  [unwired: 9 in, 1 out]
      }
      frame True {
      }
    }
    n173 = Open/Create/Replace File(file path (use dialog)=w445, operation (0:open)=T9."open or create", access (0:read/write)=enum16{"read/write", "read-only", "write-only"}."read/write") -> (refnum out=w424:refnum<file>, error out=w442:errorcluster)  [unwired: 3 in, 1 out]
    n174 = Get Date/Time String(want seconds? (F)=TRUE) -> (date string=w452:string, time string=w451:string)  [unwired: 2 in]
    n175 = Close File(refnum=w424) -> ()  [unwired: 1 in, 2 out]
    n176 = Unbundle By Name(w442) -> ("code"=w441:i32)
    n177 = Concatenate Strings("\" " ("string"), w452, "  " ("string"), w451, " \"" ("string")) -> (w450:string)
    n178 = Build Array(w450) -> (w446:string[])
    n179 = Equal?(x=w441, y=5) -> (x = y?=w439:bool)
    n180 = case shown="False" w439 {
      tunnel: w445 -> [w546 _]
      tunnel: [TRUE ("Saving Data") FALSE ("Saving Data")] -> _
      tunnel: w427 -> [w542 _]
      tunnel: w446 -> [w540 _]
      frame False {
        n181 = call "Convert from Dynamic Data3"("Dynamic Data Type"=w542) -> ("Array"=w544:dbl[])  [unwired: 3 in]
        n182 = Array Size(array=w540) -> (size(s)=w539:i32)
        n183 = Array Size(array=w544) -> (size(s)=w538:i32)
        n184 = Increment(x=w538) -> (x+1=w523:i32)
        n185 = for {
          N: w538 -> [_]
          tunnel: [w556] -> _ mode=indexing
          tunnel: [w555] -> w541 mode=indexing
          tunnel: w542 -> [w557]
          i -> [w558]
          (unwired) i16 5 ("width (-)")
          n186 = call "Convert from Dynamic Data2"("Dynamic Data Type"=w557, "Channel"=w558) -> ("Array"=w556:dbl[])  [unwired: 2 in]
          n187 = Number To Exponential String(number=w556) -> (E-format string=w555:string[])  [unwired: 3 in]
        }
        n188 = local read "New log"() -> (w536:string)
        "New log 3" <- w536
        n189 = for {
          N: w539 -> [_]
          shift-right: [w553] -> w534
          shift-left: w541 -> [w554]
          tunnel: w540 -> [w550]
          i -> [w551]
          n190 = Index Array(array=w550, index=w551) -> (element=w552:string)
          n191 = Build Array(w552) -> (w549:string[])
          n192 = Insert Into Array(array=w554, index (row)=w551, new element=w549) -> (w553:string[][])  [unwired: 1 in]
        }
        n193 = local read "error out"() -> (w535:errorcluster)
        n194 = Search and Replace String(replace all?=TRUE ("replace all? (F)"), input string=w536, search string="\r") -> (result string=w530:string)  [unwired: 5 in, 3 out]
        "New log 2" <- w530
        n195 = Unbundle By Name(w535) -> ("source"=w532:string)  [unwired: 2 out]
        n196 = property on="Current Facility State" class="Enum (strict)"() -> ("RingText.Text"=w528:string)  [unwired: 2 in, 2 out]
        n197 = property on="Target Facility State" class="Enum (strict)"() -> ("RingText.Text"=w526:string)  [unwired: 2 in, 2 out]
        n198 = Build Array(w530) -> (w529:string[])
        n199 = Build Array(w532) -> (w531:string[])
        n200 = Build Array(w528) -> (w527:string[])
        n201 = Build Array(w526) -> (w525:string[])
        n202 = Build Array(w529, w531, w527, w525) -> (w524:string[][])
        "appended array" <- w524
        n203 = Insert Into Array(array=w534, index (row)=w523, new element=w524) -> (w533:string[][])  [unwired: 1 in]
        "output array" <- w533
        n204 = call-poly <vilib>:"Write Delimited Spreadsheet.vi"("file path (dialog if empty)"=w546, "2D data"=w533, "append to file? (new file:F)"=TRUE, "transpose? (no:F)"=TRUE, "delimiter (\\t)"="," ("delimiter (\\t)")) -> ()  [unwired: 9 in, 2 out]
      }
      frame True {
        n205 = call "Display Message to User2"() -> ()  [unwired: 10 in, 2 out]
      }
    }
    n206 = local read "stop"() -> (w429:bool)
    n207 = node-c288() -> ()  [unwired: 1 in, 1 out]
  }
  n208 = Merge Errors(w171, w231) -> (w175:errorcluster)
  n209 = Merge Errors(w263, w175) -> (w262:errorcluster)
  n210 = Merge Errors(w301, w262) -> ()  [unwired: 1 out]
  n211 = Divide(x=1.0, y=w202) -> (x/y=w204:dbl)
  n212 = while {
    tunnel: w204 -> [w643]
    shift-right: [w664] -> w161
    shift-left: w156 -> [w666]
    shift-right: [w663] -> w160
    shift-left: w155 -> [w665]
    stop <- w693 stop-if-true
    n213 = Multiply(x=1000.0, y=w643) -> (x*y=w636:dbl)
    n214 = Wait Until Next ms Multiple(millisecond multiple=w636) -> ()  [unwired: 1 out]
    n215 = local read "Primary_Pump_Read"() -> (w692:bool)
    n216 = local read "Turbo 3 Motor Read"() -> (w681:bool)
    n217 = call-poly <vilib>:"DAQmx Read.vi"("task/channels in"=w666, "error in"=w665) -> ("task out"=w664:refnum<k21>, "data"=w600:waveform(dbl), "error out"=w663:errorcluster)  [unwired: 11 in]
    n218 = local read "Turbo 1 Valve"() -> (w680:bool)
    n219 = local read "Turbo 2 Valve"() -> (w606:bool)
    n220 = local read "Turbo 2 Valve"() -> (w604:bool)
    n221 = local read "Wide Range Gauge Pressure"() -> (w662:dbl)
    n222 = local read "Bypass Valve"() -> (w673:bool)
    n223 = local read "Gate 3 Valve"() -> (w617:bool)
    n224 = local read "Gate 1 Valve"() -> (w672:bool)
    n225 = local read "Gate 2 Valve"() -> (w618:bool)
    n226 = local read "Vent Valve"() -> (w642:bool)
    n227 = local read "Foreline Gauge"() -> (w659:dbl)
    n228 = local read "Turbo 3 Gauge"() -> (w633:dbl)
    n229 = local read "Turbo 2 Gauge"() -> (w634:dbl)
    n230 = local read "Turbo 1 Gauge"() -> (w647:dbl)
    n231 = Boolean To (0,1)(Boolean=w642) -> (0, 1=w641:i16)
    n232 = Boolean To (0,1)(Boolean=w617) -> (0, 1=w616:i16)
    n233 = Boolean To (0,1)(Boolean=w692) -> (0, 1=w691:i16)
    n234 = Boolean To (0,1)(Boolean=w681) -> (0, 1=w682:i16)
    n235 = Boolean To (0,1)(Boolean=w680) -> (0, 1=w679:i16)
    n236 = Boolean To (0,1)(Boolean=w606) -> (0, 1=w607:i16)
    n237 = Boolean To (0,1)(Boolean=w673) -> (0, 1=w674:i16)
    n238 = Boolean To (0,1)(Boolean=w672) -> (0, 1=w671:i16)
    n239 = Boolean To (0,1)(Boolean=w618) -> (0, 1=w619:i16)
    n240 = Boolean To (0,1)(Boolean=w604) -> (0, 1=w603:i16)
    n241 = To Double Precision Float(number=w641) -> (double precision float=w640:dbl)
    n242 = To Double Precision Float(number=w616) -> (double precision float=w614:dbl)
    n243 = To Double Precision Float(number=w691) -> (double precision float=w648:dbl)
    n244 = To Double Precision Float(number=w682) -> (double precision float=w649:dbl)
    n245 = To Double Precision Float(number=w679) -> (double precision float=w650:dbl)
    n246 = To Double Precision Float(number=w607) -> (double precision float=w609:dbl)
    n247 = To Double Precision Float(number=w674) -> (double precision float=w651:dbl)
    n248 = To Double Precision Float(number=w671) -> (double precision float=w652:dbl)
    n249 = To Double Precision Float(number=w619) -> (double precision float=w621:dbl)
    n250 = To Double Precision Float(number=w603) -> (double precision float=w602:dbl)
    n251 = Build Array(w633) -> (w626:dbl[])
    n252 = Build Array(w647) -> (w658:dbl[])
    n253 = Build Array(w634) -> (w629:dbl[])
    n254 = Build Array(w640) -> (w639:dbl[])
    n255 = Build Array(w614) -> (w615:dbl[])
    n256 = Build Array(w662) -> (w661:dbl[])
    n257 = Build Array(w659) -> (w660:dbl[])
    n258 = Build Array(w648) -> (w657:dbl[])
    n259 = Build Array(w649) -> (w656:dbl[])
    n260 = Build Array(w650) -> (w655:dbl[])
    n261 = Build Array(w609) -> (w608:dbl[])
    n262 = Build Array(w651) -> (w654:dbl[])
    n263 = Build Array(w652) -> (w653:dbl[])
    n264 = Build Array(w621) -> (w620:dbl[])
    n265 = Build Array(w602) -> (w601:dbl[])
    n266 = Bundle By Name(cluster=w600, "Y"=w639) -> (w593:waveform(dbl))
    n267 = Bundle By Name(cluster=w600, "Y"=w608) -> (w599:waveform(dbl))
    n268 = Bundle By Name(cluster=w600, "Y"=w615) -> (w594:waveform(dbl))
    n269 = Bundle By Name(cluster=w600, "Y"=w661) -> (w632:waveform(dbl))
    n270 = Bundle By Name(cluster=w600, "Y"=w660) -> (w631:waveform(dbl))
    n271 = Bundle By Name(cluster=w600, "Y"=w658) -> (w630:waveform(dbl))
    n272 = Bundle By Name(cluster=w600, "Y"=w657) -> (w646:waveform(dbl))
    n273 = Bundle By Name(cluster=w600, "Y"=w656) -> (w645:waveform(dbl))
    n274 = Bundle By Name(cluster=w600, "Y"=w655) -> (w605:waveform(dbl))
    n275 = Bundle By Name(cluster=w600, "Y"=w654) -> (w597:waveform(dbl))
    n276 = Bundle By Name(cluster=w600, "Y"=w653) -> (w596:waveform(dbl))
    n277 = Bundle By Name(cluster=w600, "Y"=w620) -> (w595:waveform(dbl))
    n278 = Bundle By Name(cluster=w600, "Y"=w629) -> (w627:waveform(dbl))
    n279 = Bundle By Name(cluster=w600, "Y"=w626) -> (w628:waveform(dbl))
    n280 = Bundle By Name(cluster=w600, "Y"=w601) -> (w598:waveform(dbl))
    n281 = Build Array(w632, w631, w630, w627, w628, w646, w645, w605, w599, w598, w597, w596, w595, w594, w593) -> (→"Waveform Chart 2":waveform(dbl)[])
    n282 = property on="Waveform Chart 2" class="WFChart (strict)"("Active Plot"=u32 9, "Plot.Plot Name"="Turbo 3 Valve") -> ()  [unwired: 2 in, 2 out]
    n283 = property on="Waveform Chart 2" class="WFChart (strict)"("Active Plot"=u32 8, "Plot.Plot Name"="Turbo 2 Valve") -> ()  [unwired: 2 in, 2 out]
    n284 = property on="Waveform Chart 2" class="WFChart (strict)"("Active Plot"=u32 10, "Plot.Plot Name"="Bypass Valve") -> ()  [unwired: 2 in, 2 out]
    n285 = property on="Waveform Chart 2" class="WFChart (strict)"("Active Plot"=u32 12, "Plot.Plot Name"="Gate 2 Valve") -> ()  [unwired: 2 in, 2 out]
    n286 = property on="Waveform Chart 2" class="WFChart (strict)"("Active Plot"=u32 11, "Plot.Plot Name"="Gate 1 Valve") -> ()  [unwired: 2 in, 2 out]
    n287 = property on="Waveform Chart 2" class="WFChart (strict)"("Active Plot"=u32 13, "Plot.Plot Name"="Gate 3 Valve") -> ()  [unwired: 2 in, 2 out]
    n288 = property on="Waveform Chart 2" class="WFChart (strict)"("Active Plot"=u32 14, "Plot.Plot Name"="Vent Valve") -> ()  [unwired: 2 in, 2 out]
    n289 = property on="Waveform Chart 2" class="WFChart (strict)"("Active Plot"=u32 5, "Plot.Plot Name"="Primary Pump") -> ()  [unwired: 2 in, 2 out]
    n290 = property on="Waveform Chart 2" class="WFChart (strict)"("Active Plot"=u32 6, "Plot.Plot Name"="Turbo Pump") -> ()  [unwired: 2 in, 2 out]
    n291 = property on="Waveform Chart 2" class="WFChart (strict)"("Active Plot"=u32 7, "Plot.Plot Name"="Turbo 1 Valve") -> ()  [unwired: 2 in, 2 out]
    n292 = property on="Waveform Chart 2" class="WFChart (strict)"("Active Plot"=u32 4, "Plot.Plot Name"="Turbo 3 Gauge") -> ()  [unwired: 2 in, 2 out]
    n293 = property on="Waveform Chart 2" class="WFChart (strict)"("Active Plot"=u32 0, "Plot.Plot Name"="Main Gauge") -> ()  [unwired: 2 in, 2 out]
    n294 = property on="Waveform Chart 2" class="WFChart (strict)"("Active Plot"=u32 1, "Plot.Plot Name"="Foreline Convectron") -> ()  [unwired: 2 in, 2 out]
    n295 = property on="Waveform Chart 2" class="WFChart (strict)"("Active Plot"=u32 2, "Plot.Plot Name"="Turbo 1 Gauge") -> ()  [unwired: 2 in, 2 out]
    n296 = property on="Waveform Chart 2" class="WFChart (strict)"("Active Plot"=u32 3, "Plot.Plot Name"="Turbo 2 Gauge") -> ()  [unwired: 2 in, 2 out]
    n297 = local read "stop"() -> (w693:bool)
  }
  n298 = while {
    shift-right: [w930] -> _
    shift-left: w339 -> [w933]
    tunnel: w206 -> [w934]
    tunnel: w348 -> [w914]
    tunnel: [w924] -> w288
    tunnel: w131 -> [w923]
    tunnel: [w922] -> _
    tunnel: [w916] -> w314
    tunnel: [w906] -> w313
    tunnel: w91 -> [w905]
    tunnel: [w901] -> w291
    tunnel: w26 -> [w895]
    tunnel: [w887] -> w261
    tunnel: w247 -> [w885]
    tunnel: [w880] -> w244
    tunnel: w237 -> [w877]
    tunnel: [w858] -> w226
    tunnel: w58 -> [w856]
    tunnel: [w850] -> w214
    tunnel: w158 -> [w849]
    tunnel: [w843] -> w213
    shift-right: [w841] -> _
    shift-left: FALSE -> [w842]
    tunnel: [w839] -> w211
    shift-right: [w696] -> _
    shift-left: FALSE -> [w836]
    shift-right: [w695] -> _
    shift-left: FALSE -> [w831]
    shift-right: [w826] -> _
    shift-left: bool[] [FALSE, FALSE, FALSE] ("appended array") -> [w827]
    shift-right: [w789] -> _
    shift-left: w130 -> [w817]
    shift-right: [w819] -> _
    shift-left: w130 -> [w818]
    shift-right: [w813] -> _
    shift-left: w23 -> [w756]
    shift-right: [w788] -> _
    shift-left: bool[] [FALSE, FALSE, FALSE] ("appended array") -> [w784]
    shift-right: [w718] -> _
    shift-left: "" -> [w781]
    shift-right: [w771] -> _
    shift-left: Facility_State."Intialize" -> [w774]
    shift-right: [w768] -> _
    shift-left: w185 -> [w766]
    shift-right: [w757] -> _
    shift-left: w184 -> [w767]
    shift-right: [w749] -> _
    shift-left: w183 -> [w755]
    tunnel: w166 -> [w748]
    tunnel: w170 -> [w747]
    tunnel: w169 -> [w746]
    tunnel: [w735] -> w168
    tunnel: [w734] -> w167
    shift-right: [w719] -> _
    shift-left: w54 -> [w722]
    shift-right: [w711] -> _
    shift-left: w23 -> [w709]
    tunnel: w18 -> [w703]
    stop <- "stop" stop-if-true
    n299 = flat-sequence {
      tunnel: w934 -> [w1072]
      tunnel: w933 -> [w1071]
      tunnel: [w1070] -> w929
      tunnel: [w1023] -> w927
      tunnel: w923 -> [w1068]
      tunnel: [w1067] -> w922
      tunnel: [w1064] -> w921
      tunnel: [w1060] -> w920
      tunnel: [w1059] -> w915
      tunnel: w914 -> [w1059]
      tunnel: [w1058] -> w910
      tunnel: w905 -> [w1057]
      tunnel: [w1057] -> w902
      tunnel: w895 -> [w1012]
      tunnel: [w1050] -> w894
      tunnel: [w986] -> w893
      tunnel: [w1013] -> w891
      tunnel: [w1053] -> w886
      tunnel: w885 -> [w1044]
      tunnel: [w1043] -> w883
      tunnel: [w1039] -> w879
      tunnel: [w1036] -> w878
      tunnel: w877 -> [w1036]
      tunnel: [w972] -> w869
      tunnel: [w974] -> w868
      tunnel: [w975] -> w867
      tunnel: w856 -> [w1034]
      tunnel: [w1033] -> w855
      tunnel: w849 -> [w1032]
      tunnel: [w1031] -> w848
      tunnel: w836 -> [w1030]
      tunnel: [w1030] -> w837
      tunnel: [w1029] -> w832
      tunnel: w831 -> [w1029]
      tunnel: [w1028] -> w828
      tunnel: w827 -> [w1028]
      tunnel: [w1027] -> w823
      tunnel: [w1026] -> w822
      tunnel: w818 -> [w1027]
      tunnel: w817 -> [w1026]
      tunnel: [w1025] -> w815
      tunnel: w756 -> [w1025]
      tunnel: w784 -> [w1021]
      tunnel: [w1021] -> w785
      tunnel: w781 -> [w1019]
      tunnel: [w1019] -> w780
      tunnel: w767 -> [w1016]
      tunnel: w766 -> [w1017]
      tunnel: [w1017] -> w765
      tunnel: [w1016] -> w762
      tunnel: w755 -> [w1015]
      tunnel: [w1015] -> w754
      tunnel: w748 -> [w995]
      tunnel: w747 -> [w999]
      tunnel: w746 -> [w998]
      tunnel: [w997] -> w745
      tunnel: [w996] -> w744
      tunnel: [w985] -> w729
      tunnel: [w984] -> w728
      tunnel: [w961] -> w725
      tunnel: w722 -> [w960]
      tunnel: [w948] -> w715
      tunnel: [w942] -> w714
      tunnel: [w945] -> w713
      tunnel: [w944] -> w710
      tunnel: w709 -> [w944]
      tunnel: w703 -> [w943]
      tunnel: [w943] -> w701
      tunnel: [w941] -> w697
      tunnel: [w935] -> w694
      tunnel: w929 -> [w1265]
      tunnel: [w1266] -> w928
      tunnel: w927 -> [w1226]
      tunnel: w921 -> [w1180]
      tunnel: w920 -> [w1261]
      tunnel: [w1261] -> w919
      tunnel: w915 -> [w1260]
      tunnel: [w1260] -> w913
      tunnel: w910 -> [w1259]
      tunnel: [w1259] -> w907
      tunnel: [w1258] -> w903
      tunnel: w902 -> [w1258]
      tunnel: w894 -> [w1171]
      tunnel: w893 -> [w1170]
      tunnel: [w1247] -> w892
      tunnel: w891 -> [w1247]
      tunnel: w886 -> [w1164]
      tunnel: [w1246] -> w884
      tunnel: w883 -> [w1246]
      tunnel: w879 -> [w1227]
      tunnel: w878 -> [w1239]
      tunnel: [w1239] -> w876
      tunnel: w869 -> [w1128]
      tunnel: w868 -> [w1131]
      tunnel: w867 -> [w1125]
      tunnel: w855 -> [w1236]
      tunnel: [w1236] -> w854
      tunnel: w848 -> [w1235]
      tunnel: [w1235] -> w847
      tunnel: [w1234] -> w838
      tunnel: w837 -> [w1234]
      tunnel: [w1233] -> w833
      tunnel: w832 -> [w1233]
      tunnel: [w1232] -> w829
      tunnel: w828 -> [w1232]
      tunnel: [w1230] -> w825
      tunnel: [w1231] -> w824
      tunnel: w823 -> [w1231]
      tunnel: w822 -> [w1230]
      tunnel: [w1229] -> w816
      tunnel: w815 -> [w1229]
      tunnel: [w1195] -> w811
      tunnel: [w1225] -> w810
      tunnel: [w1224] -> w808
      tunnel: [w1226] -> w806
      tunnel: [w1164] -> w803
      tunnel: [w1171] -> w801
      tunnel: [w1170] -> w799
      tunnel: [w1227] -> w797
      tunnel: [w1129] -> w795
      tunnel: [w1126] -> w794
      tunnel: [w1223] -> w786
      tunnel: w785 -> [w1223]
      tunnel: [w1175] -> w783
      tunnel: w780 -> [w1220]
      tunnel: [w1220] -> w779
      tunnel: w765 -> [w1219]
      tunnel: [w1219] -> w764
      tunnel: w762 -> [w1218]
      tunnel: [w1218] -> w761
      tunnel: w754 -> [w1216]
      tunnel: [w1216] -> w753
      tunnel: w745 -> [w1208]
      tunnel: w744 -> [w1207]
      tunnel: [w1208] -> w743
      tunnel: [w1207] -> w742
      tunnel: [w1192] -> w733
      tunnel: [w1172] -> w732
      tunnel: w729 -> [w1169]
      tunnel: w728 -> [w1168]
      tunnel: [w1167] -> w727
      tunnel: w725 -> [w1120]
      tunnel: [w1120] -> w723
      tunnel: w715 -> [w1127]
      tunnel: w714 -> [w1130]
      tunnel: w713 -> [w1123]
      tunnel: w710 -> [w1109]
      tunnel: [w1109] -> w708
      tunnel: [w1105] -> w702
      tunnel: w701 -> [w1105]
      tunnel: w697 -> [w1103]
      tunnel: w694 -> [w1091]
      tunnel: w928 -> [w1427]
      tunnel: [w1431] -> w932
      tunnel: [w1426] -> w931
      tunnel: w919 -> [w1454]
      tunnel: [w1454] -> w918
      tunnel: w913 -> [w1453]
      tunnel: [w1453] -> w912
      tunnel: [w1452] -> w908
      tunnel: w907 -> [w1452]
      tunnel: [w1451] -> w904
      tunnel: w903 -> [w1451]
      tunnel: [w1434] -> w900
      tunnel: [w1432] -> w899
      tunnel: w892 -> [w1450]
      tunnel: [w1450] -> w889
      tunnel: w884 -> [w1449]
      tunnel: [w1449] -> w881
      tunnel: w876 -> [w1448]
      tunnel: [w1448] -> w875
      tunnel: [w1430] -> w873
      tunnel: [w1429] -> w871
      tunnel: [w1410] -> w857
      tunnel: w854 -> [w1447]
      tunnel: [w1447] -> w853
      tunnel: w847 -> [w1446]
      tunnel: [w1446] -> w846
      tunnel: w838 -> [w1431]
      tunnel: w833 -> [w1430]
      tunnel: w829 -> [w1434]
      tunnel: w825 -> [w1432]
      tunnel: w824 -> [w1433]
      tunnel: w816 -> [w1429]
      tunnel: [w1444] -> w812
      tunnel: w811 -> [w1444]
      tunnel: w810 -> [w1443]
      tunnel: [w1443] -> w809
      tunnel: w808 -> [w1442]
      tunnel: [w1442] -> w807
      tunnel: w806 -> [w1441]
      tunnel: [w1441] -> w805
      tunnel: [w1440] -> w804
      tunnel: w803 -> [w1440]
      tunnel: [w1439] -> w802
      tunnel: w801 -> [w1439]
      tunnel: [w1438] -> w800
      tunnel: w799 -> [w1438]
      tunnel: [w1437] -> w798
      tunnel: w797 -> [w1437]
      tunnel: [w1436] -> w796
      tunnel: w795 -> [w1436]
      tunnel: w794 -> [w1435]
      tunnel: [w1435] -> w793
      tunnel: [w1433] -> w792
      tunnel: [w1425] -> w787
      tunnel: w786 -> [w1425]
      tunnel: w783 -> [w1424]
      tunnel: [w1424] -> w782
      tunnel: w779 -> [w1423]
      tunnel: [w1423] -> w778
      tunnel: w764 -> [w1422]
      tunnel: [w1422] -> w763
      tunnel: w761 -> [w1421]
      tunnel: [w1421] -> w760
      tunnel: w753 -> [w1420]
      tunnel: [w1420] -> w752
      tunnel: w743 -> [w1419]
      tunnel: w742 -> [w1418]
      tunnel: [w1419] -> w741
      tunnel: [w1418] -> w740
      tunnel: w733 -> [w1417]
      tunnel: w732 -> [w1416]
      tunnel: [w1417] -> w731
      tunnel: [w1416] -> w730
      tunnel: w727 -> [w1415]
      tunnel: [w1415] -> w726
      tunnel: [w1413] -> w724
      tunnel: w723 -> [w1414]
      tunnel: w708 -> [w1412]
      tunnel: [w1412] -> w707
      tunnel: w702 -> [w1409]
      tunnel: [w1409] -> w700
      tunnel: w932 -> [w1554]
      tunnel: w931 -> [w1553]
      tunnel: [w1552] -> w926
      tunnel: [w1551] -> w925
      tunnel: w918 -> [w1544]
      tunnel: [w1544] -> w917
      tunnel: w912 -> [w1545]
      tunnel: [w1545] -> w911
      tunnel: [w1543] -> w909
      tunnel: w908 -> [w1543]
      tunnel: w904 -> [w1546]
      tunnel: w900 -> [w1550]
      tunnel: w899 -> [w1548]
      tunnel: [w1512] -> w898
      tunnel: [w1547] -> w897
      tunnel: [w1511] -> w896
      tunnel: [w1546] -> w890
      tunnel: w889 -> [w1542]
      tunnel: [w1542] -> w888
      tunnel: [w1541] -> w882
      tunnel: w881 -> [w1541]
      tunnel: w875 -> [w1540]
      tunnel: [w1540] -> w874
      tunnel: w873 -> [w1539]
      tunnel: [w1538] -> w872
      tunnel: w871 -> [w1537]
      tunnel: [w1483] -> w870
      tunnel: w857 -> [w1536]
      tunnel: w853 -> [w1535]
      tunnel: [w1535] -> w852
      tunnel: w846 -> [w1534]
      tunnel: [w1534] -> w845
      tunnel: w812 -> [w1533]
      tunnel: w809 -> [w1532]
      tunnel: w807 -> [w1531]
      tunnel: w805 -> [w1530]
      tunnel: w804 -> [w1529]
      tunnel: w802 -> [w1528]
      tunnel: w800 -> [w1515]
      tunnel: w798 -> [w1527]
      tunnel: w796 -> [w1526]
      tunnel: w793 -> [w1525]
      tunnel: w792 -> [w1549]
      tunnel: [w1524] -> w791
      tunnel: w787 -> [w1523]
      tunnel: w782 -> [w1522]
      tunnel: w778 -> [w1521]
      tunnel: [w1520] -> w777
      tunnel: w774 -> [w1494]
      tunnel: [w1507] -> w773
      tunnel: [w1519] -> w770
      tunnel: w763 -> [w1518]
      tunnel: w760 -> [w1517]
      tunnel: [w1516] -> w759
      tunnel: w752 -> [w1514]
      tunnel: [w1513] -> w751
      tunnel: w741 -> [w1492]
      tunnel: w740 -> [w1491]
      tunnel: [w1492] -> w739
      tunnel: [w1491] -> w738
      tunnel: w731 -> [w1488]
      tunnel: w730 -> [w1487]
      tunnel: w726 -> [w1486]
      tunnel: w724 -> [w1485]
      tunnel: [w1484] -> w720
      tunnel: w707 -> [w1481]
      tunnel: [w1482] -> w706
      tunnel: [w1480] -> w705
      tunnel: [w1479] -> w704
      tunnel: w700 -> [w1478]
      tunnel: [w1478] -> w699
      tunnel: [w1477] -> w698
      tunnel: w926 -> [w2941]
      tunnel: w925 -> [w3011]
      tunnel: w917 -> [w3009]
      tunnel: w911 -> [w3008]
      tunnel: w909 -> [w3007]
      tunnel: w898 -> [w2974]
      tunnel: w897 -> [w2959]
      tunnel: w896 -> [w2958]
      tunnel: w890 -> [w3003]
      tunnel: w888 -> [w3002]
      tunnel: w882 -> [w3001]
      tunnel: w874 -> [w3000]
      tunnel: w872 -> [w2942]
      tunnel: w870 -> [w2946]
      tunnel: [w3010] -> w866
      tunnel: [w3012] -> w865
      tunnel: [w3009] -> w864
      tunnel: [w3007] -> w863
      tunnel: [w3006] -> w862
      tunnel: [w3002] -> w861
      tunnel: [w3001] -> w860
      tunnel: [w2999] -> w859
      tunnel: w852 -> [w2992]
      tunnel: [w2992] -> w851
      tunnel: w845 -> [w2991]
      tunnel: [w2991] -> w844
      tunnel: [w2990] -> w840
      tunnel: [w2941] -> w835
      tunnel: [w2942] -> w830
      tunnel: [w2958] -> w821
      tunnel: [w2959] -> w820
      tunnel: [w2946] -> w814
      tunnel: w791 -> [w2967]
      tunnel: [w2967] -> w790
      tunnel: w777 -> [w2986]
      tunnel: [w2986] -> w776
      tunnel: [w2974] -> w775
      tunnel: w773 -> [w2982]
      tunnel: [w2982] -> w772
      tunnel: w770 -> [w2981]
      tunnel: [w2981] -> w769
      tunnel: w759 -> [w2980]
      tunnel: [w2980] -> w758
      tunnel: w751 -> [w2979]
      tunnel: [w2979] -> w750
      tunnel: w739 -> [w2978]
      tunnel: w738 -> [w2977]
      tunnel: [w2978] -> w737
      tunnel: [w2977] -> w736
      tunnel: [w2954] -> w721
      tunnel: w720 -> [w2954]
      tunnel: [w2949] -> w712
      tunnel: w706 -> [w2949]
      tunnel: w705 -> [w2945]
      tunnel: w704 -> [w2947]
      tunnel: w699 -> [w2950]
      tunnel: w698 -> [w2948]
      tunnel: [w3078] -> w858
      tunnel: [w3079] -> w880
      tunnel: [w3080] -> w887
      tunnel: [w3081] -> w901
      tunnel: [w3082] -> w906
      tunnel: [w3083] -> w916
      tunnel: [w3084] -> w924
      tunnel: [w3085] -> w930
      tunnel: w866 -> [w3085]
      tunnel: w865 -> [w3084]
      tunnel: w864 -> [w3083]
      tunnel: w863 -> [w3082]
      tunnel: w862 -> [w3081]
      tunnel: w861 -> [w3080]
      tunnel: w860 -> [w3079]
      tunnel: w859 -> [w3078]
      tunnel: w851 -> [w3076]
      tunnel: [w3076] -> w850
      tunnel: w844 -> [w3075]
      tunnel: [w3075] -> w843
      tunnel: w840 -> [w3074]
      tunnel: [w3074] -> w839
      tunnel: w835 -> [w3051]
      tunnel: [w3051] -> w696
      tunnel: w830 -> [w3046]
      tunnel: [w3046] -> w695
      tunnel: [w3027] -> w826
      tunnel: [w3057] -> w789
      tunnel: w821 -> [w3057]
      tunnel: [w3073] -> w819
      tunnel: w820 -> [w3073]
      tunnel: w814 -> [w3040]
      tunnel: [w3040] -> w813
      tunnel: w790 -> [w3064]
      tunnel: [w3064] -> w788
      tunnel: [w3026] -> w718
      tunnel: w776 -> [w3056]
      tunnel: w775 -> [w3027]
      tunnel: w772 -> [w3037]
      tunnel: [w3037] -> w771
      tunnel: w769 -> [w3036]
      tunnel: [w3036] -> w768
      tunnel: w758 -> [w3035]
      tunnel: [w3035] -> w757
      tunnel: w750 -> [w3034]
      tunnel: [w3034] -> w749
      tunnel: w737 -> [w3032]
      tunnel: w736 -> [w3033]
      tunnel: [w3033] -> w735
      tunnel: [w3032] -> w734
      tunnel: w721 -> [w3028]
      tunnel: [w3028] -> w719
      tunnel: [w3020] -> w711
      tunnel: w712 -> [w3020]
      frame #0 {
        w978 = 10178 items=["Finite Samples"=10178, "Continuous Samples"=10123, "Hardware Timed Single Point"=12522] ("sample mode")
        w994 = FALSE
        w1010 = 10178 items=["Finite Samples"=10178, "Continuous Samples"=10123, "Hardware Timed Single Point"=12522] ("sample mode")
        # "Get Turbo 2 Error"
        # "Drop below threshold long enough to close Breather"
        # "Turbo 2 Read"
        # "Turbo 1 Cluster"
        # "Turbo 1 Read"
        # "Get Turbo 3 Error"
        # "Note this error in line\nfrom the other AI in \ntask must be attached\nto ensure they are read \nsequentially! Otherwise \nthis will throw an error"
        # "Convert 0-10V to 0-100% Turbo Speed"
        # "Turbo Speed Read"
        # "Turbo Error Read"
        # "Turbo Read"
        # "Chiller Read"
        # "Gauge Read"
        # "Valve Read"
        # "Read Current Status"
        # "Primary Pump Read"
        n300 = call-poly <vilib>:"DAQmx Timing.vi"("task/channels in"=w1012, "sample mode"=w1010, "samples per channel"="samples per channel", "rate"="rate") -> ("task out"=w1001:refnum<k21>, "error out"=w1000:errorcluster)  [unwired: 10 in]
        n301 = call-poly <vilib>:"DAQmx Read.vi"("task/channels in"=w1068) -> ("task out"=w1058:refnum<k21>, "data"=w1066:bool[], "error out"=w1067:errorcluster)  [unwired: 12 in]
        n302 = call-poly <vilib>:"DAQmx Read.vi"("task/channels in"=w1044) -> ("task out"=w1043:refnum<k21>, "data"=w1038:bool, "error out"=w1041:errorcluster)  [unwired: 12 in]
        n303 = call-poly <vilib>:"DAQmx Read.vi"("task/channels in"=w1072) -> ("task out"=w1060:refnum<k21>, "data"=w959:bool, "error out"=w1046:errorcluster)  [unwired: 12 in]
        n304 = call-poly <vilib>:"DAQmx Timing.vi"("task/channels in"=w1032, "sample mode"=w978, "samples per channel"=2000, "rate"=4000.0) -> ("task out"=w979:refnum<k21>)  [unwired: 10 in, 1 out]
        n305 = case shown="False" w995 {
          tunnel: w999 -> [w1075 w1085]
          tunnel: w998 -> [w1074 w1084]
          tunnel: [w1074 w1078] -> w997
          tunnel: [w1075 w1077] -> w996
          tunnel: [0.0 ("Measurement") w1076] -> _
          frame False {
          }
          frame True {
            n306 = call <instrlib>:"Backlight Command.vi"("error in (no error)"=w1084, "ON/OFF"="ON/OFF", "VISA resource name"=w1085) -> ("error out"=w1081:errorcluster, "VISA resource name out"=w1082:refnum<visa-resource-name>)  [unwired: 7 in]
            n307 = call <instrlib>:"Read (Single Point).vi"("error in (no error)"=w1081, "VISA resource name"=w1082) -> ("error out"=w1079:errorcluster, "Measurement"=w1076:dbl, "VISA resource name out"=w1077:refnum<visa-resource-name>)  [unwired: 7 in]
            "Measurement" <- w1076
            n308 = call <vilib>:"Clear Errors.vi"("error in (no error)"=w1079, "specific error code to clear (0: all)"=1073676294) -> ("error out"=w1078:errorcluster)  [unwired: 4 in, 1 out]
          }
        }
        n309 = Build Array("Fake_Valve_Turbo_Read", "Fake_Valve_Bypass_Read", "Fake_Valve_Vent_Read", "Fake_Valve_Gate_Read", w994, w994, w994, w994) -> (w1065:bool[])
        n310 = call-poly <vilib>:"DAQmx Read.vi"("task/channels in"=w1001, "number of samples per channel"="samples per channel", "error in"=w1000) -> ("task out"=w1013:refnum<k21>, "data"=w938:waveform(dbl)[], "error out"=w1014:errorcluster)  [unwired: 10 in]
        n311 = Index Array(array=w938, index=0) -> (element=w1009:waveform(dbl))
        n312 = Index Array(array=w938, index=2) -> (element=w1006:waveform(dbl))
        n313 = Index Array(array=w938, index=3) -> (element=w991:waveform(dbl))
        n314 = Index Array(array=w938, index=5) -> (element=w939:waveform(dbl))
        n315 = Index Array(array=w938, index=4) -> (element=w988:waveform(dbl))
        n316 = Index Array(array=w938, index=1) -> (element=w1008:waveform(dbl))
        n317 = call-poly <vilib>:"Mean.vi"("X"=w1006) -> ("mean"=w1005:dbl)  [unwired: 1 out]
        n318 = call-poly <vilib>:"Mean.vi"("X"=w991) -> ("mean"=w992:dbl)  [unwired: 1 out]
        n319 = call-poly <vilib>:"Mean.vi"("X"=w1009) -> ("mean"=w993:dbl)  [unwired: 1 out]
        n320 = call-poly <vilib>:"Mean.vi"("X"=w1008) -> ("mean"=w1007:dbl)  [unwired: 1 out]
        n321 = call-poly <vilib>:"Mean.vi"("X"=w939) -> ("mean"=w937:dbl)  [unwired: 1 out]
        n322 = call-poly <vilib>:"Mean.vi"("X"=w988) -> ("mean"=w987:dbl)  [unwired: 1 out]
        n323 = formula code="P_Gage_mBar = (10**(((V-6.143)/1.286)));" "Turbo 1 Pressure calculation (mBar)"("V"=w1005) -> ("P_Gage_mBar"=w1049:dbl)
        n324 = formula code="P_Gage_mBar = (10**(((V-6.143)/1.286)));" "Foreline 1 Pressure calculation (mBar)"("V"=w1007) -> ("P_Gage_mBar"=w1051:dbl)
        n325 = formula code="P_Gage_mBar = (10**(((V-6.143)/1.286)));" "Turbo 2 Pressure calculation (mBar)"("V"=w992) -> ("P_Gage_mBar"=w985:dbl)
        n326 = formula code="Pressure_Bar = (V/5*10);" "Air Compressor Pressure Calc (Bar)"("V"=w937) -> ("Pressure_Bar"=w935:dbl)
        n327 = formula code="P_Gage_mBar = (10**(((V-6.143)/1.286)));" "Turbo 3 Pressure calculation (mBar)"("V"=w987) -> ("P_Gage_mBar"=w984:dbl)
        n328 = formula code="P_WRG_mBar = 10**((V-6.8)/0.6);" "Ion gauge Pressure calculation (mBar)"("V"=w993) -> ("P_WRG_mBar"=w1018:dbl)
        n329 = call-poly <vilib>:"DAQmx Read.vi"("task/channels in"=w979, "error in"=w1014) -> ("task out"=w1031:refnum<k21>, "data"=w949:waveform(dbl)[], "error out"=w982:errorcluster)  [unwired: 11 in]
        n330 = Index Array(array=w949, index=7) -> (element=w977:waveform(dbl))
        n331 = Index Array(array=w949, index=6) -> (element=w954:waveform(dbl))
        n332 = call-poly <vilib>:"Mean.vi"("X"=w977) -> ("mean"=w976:dbl)  [unwired: 1 out]
        n333 = call-poly <vilib>:"Mean.vi"("X"=w954) -> ("mean"=w953:dbl)  [unwired: 1 out]
        n334 = local read "Use_real_Values?"() -> (w1024:bool)
        n335 = call-poly <vilib>:"DAQmx Read.vi"("task/channels in"=w1034, "error in"=w982) -> ("task out"=w1033:refnum<k21>, "data"=w946:bool[], "error out"=w1035:errorcluster)  [unwired: 11 in]
        n336 = Multiply(x=w953, y=10.0) -> (x*y=w942:dbl)
        "Numeric 2" <- w942
        n337 = Multiply(x=w976, y=10.0) -> (x*y=w974:dbl)
        "Numeric" <- w974
        n338 = Multiply(x=0.0, y=10.0) -> (x*y=w941:dbl)
        "Numeric 3" <- w941
        n339 = Merge Errors(w1041, w1035) -> (w1040:errorcluster)
        n340 = Merge Errors(w1014, w1040) -> (w1042:errorcluster)
        n341 = Merge Errors(w1046, w1042) -> (w1045:errorcluster)
        n342 = Number To Decimal String(number=w942, width (-)=i16 0) -> (decimal integer string=→"Turbo 2 Speed":string)
        n343 = Number To Decimal String(number=w974, width (-)=i16 0) -> (decimal integer string=→"Turbo 3 Speed":string)
        n344 = Number To Decimal String(number=w941, width (-)=i16 0) -> (decimal integer string=→"Ecodry Speed":string)
        n345 = Select(t=w959, s=w1024, f="Fake_Primary_Pump_Read") -> (s? t:f=w1023:bool)
        n346 = Select(t=w1038, s=w1024, f="Fake_Chiller_Read") -> (s? t:f=w1039:bool)
        n347 = Merge Errors(w1071, w1045) -> (w1070:errorcluster)
        n348 = Select(t=w1066, s=w1024, f=w1065) -> (s? t:f=w1064:bool[])
        n349 = Array Subset(array=w946, index=0, length=6) -> (w969:bool[])
        n350 = Array To Cluster(array=w969) -> (cluster=w968:T13)
        n351 = Unbundle(w968) -> ("[0]"=w967:bool, "[1]"=w966:bool, "[2]"=w965:bool, "[3]"=w964:bool, "[4]"=w963:bool, "[5]"=w962:bool)
        n352 = Bundle By Name(cluster=w960, "Turbo Rotating Read"=w967, "Turbo Accelarating Read"=w966, "Turbo At Speed Read"=w965, "Turbo Breaking Read"=w964, "Turbo Alarm Read"=w963, "Turbo Warning Read"=w962) -> (w961:T3)
        n353 = local read "Turbo_2_Motor_Sys_Cmd"() -> (w948:bool)
        "Turbo 2 Motor Read" <- w948
        n354 = local read "Turbo_3_Motor_Sys_Cmd"() -> (w972:bool)
        "Turbo 3 Motor Read" <- w972
        n355 = Index Array(array=w946, index=6) -> (element=w945:bool)
        n356 = local write "Turbo 3 Motor Read"(w972) -> ()
        n357 = local write "Turbo 2 Motor Read"(w948) -> ()
        n358 = Index Array(array=w946, index=7) -> (element=w975:bool)
        n359 = Select(t=w1051, s=w1024, f="Fake_Fore_Pressure_mBar") -> (s? t:f=w1050:dbl)
        n360 = Select(t=w1018, s=w1024, f="Fake_WRG_Pressure_mBar") -> (s? t:f=w1053:dbl)
        n361 = Select(t=w1049, s=w1024, f="Fake_Turbo_1_Pressure_mBar") -> (s? t:f=w986:dbl)
      }
      frame #1 {
        w1093 = 5.0  # Compressor Threashold (Bar)
        w1089 = errorcluster {"status"=FALSE, "code"=5010, "source"="Compressor Pressure Below 5 Bar!"}  # Compressor Error
        w1094 = 5.0  # Min time below threshhold (s)
        w1182 = errorcluster {"status"=FALSE, "code"=5010, "source"="Conflict between Gate 1 Valve command and read!"}  # Valve Gate Error
        w1187 = errorcluster {"status"=FALSE, "code"=5010, "source"="Conflict between Gate 1 Valve command and read!"}  # Valve Gate Error
        w1198 = errorcluster {"status"=FALSE, "code"=5001, "source"="Conflict between turbo 3 valve command and read!"}  # Valve Turbo 3 Error
        w1206 = errorcluster {"status"=FALSE, "code"=5001, "source"="Conflict between turbo 2 valve command and read!"}  # Valve Turbo 2 Error
        w1189 = errorcluster {"status"=FALSE, "code"=5010, "source"="Conflict between Gate 1 Valve command and read!"}  # Valve Gate Error
        w1214 = errorcluster {"status"=FALSE, "code"=5004, "source"="Conflict between Chiller command and read!"}  # Chiller Error
        w1212 = errorcluster {"status"=FALSE, "code"=0, "source"=""}  # No Error
        w1249 = errorcluster {"status"=FALSE, "code"=5003, "source"="Conflict between Vent Valve command and read!"}  # Valve Vent Error
        w1253 = errorcluster {"status"=FALSE, "code"=5002, "source"="Conflict between Bypass Valve command and read!"}  # Valve Bypass Error
        w1181 = errorcluster {"status"=FALSE, "code"=0, "source"=""}  # No Error
        w1256 = errorcluster {"status"=FALSE, "code"=5001, "source"="Conflict between turbo 1 valve command and read!"}  # Valve Turbo 1 Error
        # "And turbo valve open"
        # "Drop below threshold long enough"
        # "Foreline Pressure Reached?"
        # "WRG Pressure reached?"
        # "Check For Turbo Errors and Display Status"
        # "Check For Chiller Errors and Display Status"
        # "Display Gauge"
        # "Check For Primary Pump Errors and Display Status"
        # "Check For Valve Errors and Display Status"
        # "Check Status for error, and display status"
        n362 = local read "Use Ecodry As Primary?"() -> (w1104:bool)
        n363 = Build Array(w1123, w1125) -> (w1124:bool[])
        n364 = local read "Chiller_Sys_Cmd"() -> (w1217:bool)
        n365 = Build Array(w1130, w1131) -> (w1129:dbl[])
        n366 = Build Array(w1127, w1128) -> (w1126:bool[])
        n367 = local read "Which_Turbos_used?"() -> (w1100:bool[])
        n368 = local read "Chiller_Sys_Cmd"() -> (w1242:bool)
        n369 = Unbundle By Name(w1120) -> ("Turbo Accelarating Read"=w1156:bool)
        n370 = Unbundle By Name(w1120) -> ("Turbo Standby SYS CMD"=w1152:bool)
        n371 = Unbundle By Name(w1120) -> ("Turbo Warning Read"=w1159:bool)
        n372 = Unbundle By Name(w1120) -> ("Turbo At Speed Read"=w1149:bool)
        n373 = Unbundle By Name(w1120) -> ("Turbo Breaking Read"=w1153:bool)
        n374 = Unbundle By Name(w1120) -> ("Turbo Rotating Read"=w1144:bool)
        n375 = Unbundle By Name(w1120) -> ("Turbo Alarm Read"=w1161:bool)
        n376 = local read "Turbo 2 Standby?"() -> (w1108:bool)
        n377 = local read "Turbo 3 Standby?"() -> (w1107:bool)
        n378 = local read "Valve_Turbo_1_Sys_Cmd"() -> (w1257:bool)
        n379 = local read "Valve_Gate_2_Sys_Cmd"() -> (w1186:bool)
        n380 = local read "Valve_Gate_3_Sys_Cmd"() -> (w1183:bool)
        n381 = local read "Valve_Gate_1_Sys_Cmd"() -> (w1190:bool)
        n382 = local read "Valve_Bypass_Sys_Cmd"() -> (w1252:bool)
        n383 = local read "Valve_Vent_Sys_Cmd"() -> (w1251:bool)
        n384 = local read "Valve_Turbo_2_Sys_Cmd"() -> (w1205:bool)
        n385 = local read "Valve_Turbo_3_Sys_Cmd"() -> (w1199:bool)
        n386 = Index Array(array=w1180, index=6) -> (element=w1174:bool)
        "Gate 2 Valve" <- w1174
        n387 = Index Array(array=w1180, index=7) -> (element=w1173:bool)
        "Gate 3 Valve" <- w1173
        n388 = Index Array(array=w1180, index=0) -> (element=w1225:bool)
        "Bypass Valve" <- w1225
        n389 = Index Array(array=w1180, index=5) -> (element=w1175:bool)
        "Gate 1 Valve" <- w1175
        n390 = Index Array(array=w1180, index=1) -> (element=w1224:bool)
        "Vent Valve" <- w1224
        n391 = Index Array(array=w1180, index=2) -> (element=w1195:bool)
        "Turbo 1 Valve" <- w1195
        n392 = Not(x=w1161) -> (.not. x?=w1139:bool)
        n393 = Index Array(array=w1180, index=3) -> (element=w1194:bool)
        "Turbo 2 Valve" <- w1194
        n394 = Index Array(array=w1100, index=1) -> (element=w1098:bool)
        n395 = Index Array(array=w1180, index=4) -> (element=w1193:bool)
        "Turbo 3 Valve" <- w1193
        n396 = Not(x=w1159) -> (.not. x?=w1137:bool)
        n397 = Or(x=w1137, y=w1139) -> (x .or. y?=w1138:bool)
        n398 = case shown="True" w1138 {
          tunnel: w1137 -> [_ w1382]
          tunnel: [w1377 w1379] -> w1136
          tunnel: errorcluster {"status"=FALSE, "code"=0, "source"=""} ("error constant") -> [w1377 w1380]
          frame False {
          }
          frame True {
            n399 = Select(t=" Warning" ("source"), s=w1382, f=" Alarm" ("source")) -> (s? t:f=w1381:string)
            n400 = Concatenate Strings("Turbo" ("string"), "1" ("string"), w1381) -> (w1386:string)
            n401 = Bundle By Name(cluster=w1380, "status"=TRUE, "code"=5005, "source"=w1386) -> (w1379:errorcluster)
          }
        }
        n402 = Select(t=enum16{"Off", "On", "Error"}."On", s=w1227, f=enum16{"Off", "On", "Error"}."Off") -> (s? t:f=w1241:enum16{"Off", "On", "Error"})
        n403 = Exclusive Or(1:w1227, 2:w1242) -> (0:w1213:bool)
        n404 = local write "Vent Valve"(w1224) -> ()
        n405 = local write "Bypass Valve"(w1225) -> ()
        n406 = Build Array(w1108, w1107) -> (w1106:bool[])
        n407 = Index Array(array=w1100, index=2) -> (element=w1097:bool)
        n408 = local write "Turbo 1 Valve"(w1195) -> ()
        n409 = local write "Turbo 2 Valve"(w1194) -> ()
        n410 = local write "Turbo 3 Valve"(w1193) -> ()
        n411 = Or(x=w1153, y=w1144) -> (x .or. y?=w1145:bool)
        n412 = Select(t=enum16{"Off", "On", "Error"}."Error", s=w1213, f=w1241) -> (s? t:f=w1240:enum16{"Off", "On", "Error"})
        n413 = local write "Gate 2 Valve"(w1174) -> ()
        n414 = local write "Gate 3 Valve"(w1173) -> ()
        n415 = local write "Gate 1 Valve"(w1175) -> ()
        n416 = Build Array(w1098, w1097) -> (w1096:bool[])
        n417 = case shown="\"On\"" w1240 {
          tunnel: [u32 12632256 ("Color") u32 6618880 ("Color") u32 16711680 ("Color")] -> w1228
          tunnel: ["Chiller is Off" "Chiller is On" "Chiller error"] -> w1237
          frame "Off", Default {
          }
          frame "On" {
          }
          frame "Error" {
          }
        }
        "Chiller Status" <- w1237
        "Chiller Status 2" <- w1228
        n418 = Select(t=w1214, s=w1213, f=w1212) -> (s? t:f=w1215:errorcluster)
        n419 = Exclusive Or(1:w1186, 2:w1174) -> (0:w1179:bool)
        "Gate 2 Valve Error?" <- w1179
        n420 = Exclusive Or(1:w1183, 2:w1173) -> (0:w1178:bool)
        "Gate 3 Valve Error?" <- w1178
        n421 = Select(t=T10."Spinning Down", s=w1145, f=T10."Off") -> (s? t:f=w1146:T10)
        n422 = Select(t=T10."Speed Reached", s=w1149, f=w1146) -> (s? t:f=w1148:T10)
        n423 = Select(t=T10."Turbo in Standby", s=w1152, f=w1148) -> (s? t:f=w1147:T10)
        n424 = Select(t=T10."Spinning Up", s=w1156, f=w1147) -> (s? t:f=w1158:T10)
        n425 = Select(t=T10."Turbo Warning", s=w1137, f=w1158) -> (s? t:f=w1160:T10)
        n426 = Select(t=T10."Error", s=w1139, f=w1160) -> (s? t:f=w1135:T10)
        n427 = Exclusive Or(1:w1190, 2:w1175) -> (0:w1188:bool)
        "Gate 1 Valve Error?" <- w1188
        n428 = Exclusive Or(1:w1252, 2:w1225) -> (0:w1210:bool)
        "Bypass Valve Error?" <- w1210
        n429 = Exclusive Or(1:w1251, 2:w1224) -> (0:w1209:bool)
        "Vent Valve Error?" <- w1209
        n430 = Exclusive Or(1:w1257, 2:w1195) -> (0:w1211:bool)
        "Turbo 1 Valve Error?" <- w1211
        n431 = Exclusive Or(1:w1205, 2:w1194) -> (0:w1203:bool)
        "Turbo 2 Valve Error?" <- w1203
        n432 = Exclusive Or(1:w1199, 2:w1193) -> (0:w1196:bool)
        "Turbo 3 Valve Error?" <- w1196
        n433 = Less?(x=w1091, y=w1093) -> (x < y?=w1092:bool)
        n434 = case shown="\"Spinning Up\"" w1135 {
          tunnel: [u32 12632256 ("Color") u32 3381759 ("Color") u32 6618880 ("Color") u32 10650795 ("Color") u32 16514929 ("Color") u32 16757266 ("Color") u32 16711680 ("Color")] -> w1132
          tunnel: ["Off" "Accel" "Normal" "Decel" "In Standby" "Warning" "Error"] -> w1141
          frame "Off", Default {
          }
          frame "Spinning Up" {
          }
          frame "Speed Reached" {
          }
          frame "Spinning Down" {
          }
          frame "Turbo in Standby" {
          }
          frame "Turbo Warning" {
          }
          frame "Error" {
          }
        }
        "Turbo 1 Status Color" <- w1132
        n435 = Select(t=w1256, s=w1211, f=w1181) -> (s? t:f=w1202:errorcluster)
        n436 = Select(t=w1187, s=w1179, f=w1181) -> (s? t:f=w1177:errorcluster)
        n437 = Select(t=w1182, s=w1178, f=w1181) -> (s? t:f=w1176:errorcluster)
        n438 = Select(t=w1189, s=w1188, f=w1181) -> (s? t:f=w1221:errorcluster)
        n439 = Select(t=w1206, s=w1203, f=w1181) -> (s? t:f=w1201:errorcluster)
        n440 = Select(t=w1198, s=w1196, f=w1181) -> (s? t:f=w1197:errorcluster)
        n441 = Select(t=w1249, s=w1209, f=w1181) -> (s? t:f=w1250:errorcluster)
        n442 = Select(t=w1253, s=w1210, f=w1181) -> (s? t:f=w1254:errorcluster)
        n443 = Divide(x=w1164, y=1.33322368) -> (x/y=→"WRG (torr)":dbl)
        n444 = Build Array(w1170, w1169, w1168) -> (w1167:dbl[])
        n445 = call "Is Value Changed.vim"("value"=w1092) -> ("changed or first call?"=w1095:bool)
        n446 = Merge Errors(w1136) -> (w1122:errorcluster)
        n447 = for {
          tunnel: w1126 -> [w1357] mode=indexing
          tunnel: w1217 -> [_]
          tunnel: [w1333] -> w1111 mode=indexing
          tunnel: [w1352] -> w1117 mode=indexing
          tunnel: w1129 -> [w1322] mode=indexing
          tunnel: w1124 -> [w1329] mode=indexing
          shift-right: [w1344] -> w1121
          shift-left: w1122 -> [w1345]
          tunnel: w1106 -> [w1324] mode=indexing
          tunnel: w1096 -> [w1327] mode=indexing
          i -> [w1343]
          w1348 = errorcluster {"status"=FALSE, "code"=0, "source"=""}  # No Error
          w1360 = 5.0  # Turbo Slow Speed  Threshold
          w1359 = 95.0  # Turbo Speed Reached  Threshold
          # "Ignore Turbo Error if chiller off"
          n448 = Not(x=w1329) -> (.not. x?=w1328:bool)
          n449 = Equal?(x=0, y=w1343) -> (x = y?=w1337:bool)
          n450 = And(x=w1327, y=w1328) -> (x .and. y?=w1326:bool)
          n451 = Greater?(x=w1322, y=40.0) -> (0:w1320:bool)
          n452 = Select(t="Turbo 2 Error." ("string"), s=w1337, f="Turbo 3 Error." ("string")) -> (s? t:f=w1339:string)
          n453 = Greater?(x=w1322, y=w1359) -> (0:w1325:bool)
          n454 = And(x=w1324, y=w1320) -> (x .and. y?=w1323:bool)
          n455 = Select(t=T11."Turbo in Standby", s=w1323, f=T11."Spinning Up") -> (s? t:f=w1331:T11)
          n456 = Select(t=T12."Speed Reached", s=w1325, f=w1331) -> (s? t:f=w1351:u16)
          n457 = Bundle By Name(cluster=w1348, "status"=TRUE, "code"=5007, "source"=w1339) -> (w1350:errorcluster)
          n458 = Greater?(x=w1322, y=w1360) -> (0:w1362:bool)
          n459 = Select(t=T11."Spinning Down", s=w1362, f=T11."Off") -> (s? t:f=w1363:T11)
          n460 = Select(t=w1351, s=w1357, f=w1363) -> (s? t:f=w1364:u16)
          n461 = Select(t=T12."Error", s=w1326, f=w1364) -> (s? t:f=w1361:u16)
          n462 = Or(x=w1326, y=FALSE) -> ()  [unwired: 1 out]
          n463 = case shown="4" w1361 {
            tunnel: [u32 12632256 ("Color") u32 3381759 ("Color") u32 6618880 ("Color") u32 10650795 ("Color") u32 16757266 ("Color") u32 16711680 ("Color")] -> w1352
            tunnel: [" Off" " Accel" " Normal" " Decel" " In Standby" " Error"] -> w1338
            frame 0, Default {
            }
            frame 1 {
            }
            frame 2 {
            }
            frame 3 {
            }
            frame 4 {
            }
            frame 5 {
            }
          }
          n464 = Select(t=" Turbo 2 ", s=w1337, f=" Turbo 3 ") -> (s? t:f=w1334:string)
          n465 = Select(t=w1350, s=w1326, f=w1348) -> (s? t:f=w1349:errorcluster)
          n466 = Concatenate Strings(w1334, w1338) -> (w1333:string)
          n467 = Merge Errors(w1349, w1345) -> (w1344:errorcluster)
        }
        n468 = case shown="True" w1092 {
          tunnel: w1095 -> [_ w1274]
          tunnel: [FALSE ("Time has Elapsed") w1272] -> w1090
          tunnel: [0.0 ("Elapsed Time (s)") w1270] -> _
          tunnel: w1094 -> [_ w1271]
          frame False {
          }
          frame True {
            n469 = call "Elapsed Time5"("Time Target (s)"=w1271, "Reset"=w1274, "Auto Reset"=FALSE) -> ("Elapsed Time (s)"=w1270:dbl, "Time has Elapsed"=w1272:bool)  [unwired: 9 in, 6 out]
          }
        }
        "Low Compressor Pressure!" <- w1090
        n470 = property on="Low Compressor Pressure!" class="Bool (strict)"("Visible"=w1090) -> ()  [unwired: 2 in, 2 out]
        n471 = Concatenate Strings("Turbo " ("string"), "1" ("string"), " " ("string"), w1141) -> (→"Turbo 1 Status":string)
        n472 = Select(t=w1089, s=w1090, f=errorcluster {"status"=FALSE, "code"=0, "source"=""}) -> (s? t:f=w1087:errorcluster)
        n473 = Merge Errors(w1215, w1121) -> (w1238:errorcluster)
        n474 = Index Array(array=w1111, index=0) -> (element=→"Turbo 2 Status":string)
        n475 = Index Array(array=w1111, index=1) -> (element=→"Turbo 3 Status":string)
        n476 = Build Array(w1195, w1194, w1193) -> (w1192:bool[])
        n477 = Index Array(array=w1117, index=0) -> (element=→"Turbo 2 Status Color":u32)
        n478 = Index Array(array=w1117, index=1) -> (element=→"Turbo 3 Status Color":u32)
        n479 = Build Array(w1175, w1174, w1173) -> (w1172:bool[])
        n480 = Merge Errors(w1087, w1238) -> (w1088:errorcluster)
        n481 = case shown="True" w1104 {
          tunnel: [w1289 w1308] -> w1267
          tunnel: [w1283 w1307] -> w1248
          tunnel: w1088 -> [w1279 w1313]
          tunnel: w1226 -> [w1278 _]
          tunnel: [w1277 w1313] -> w1222
          tunnel: w1103 -> [_ w1312]
          tunnel: [FALSE ("Visible") TRUE ("Visible")] -> w1102
          frame False {
            w1285 = errorcluster {"status"=FALSE, "code"=5000, "source"="Conflict between Primary pump command and read!"}  # Pump Error
            w1284 = errorcluster {"status"=FALSE, "code"=0, "source"=""}  # No Error
            # "Varodry"
            n482 = local read "Primary_Sys_Cmd"() -> (w1290:bool)
            n483 = Select(t=enum16{"Off", "On", "Error"}."On", s=w1278, f=enum16{"Off", "On", "Error"}."Off") -> (s? t:f=w1291:enum16{"Off", "On", "Error"})
            n484 = Exclusive Or(1:w1278, 2:w1290) -> (0:w1276:bool)
            n485 = Select(t=enum16{"Off", "On", "Error"}."Error", s=w1276, f=w1291) -> (s? t:f=w1292:enum16{"Off", "On", "Error"})
            n486 = case shown="\"On\"" w1292 {
              tunnel: [u32 12632256 ("Color") u32 6618880 ("Color") u32 16711680 ("Color")] -> w1289
              tunnel: ["is Off" "is On" "Error"] -> w1282
              frame "Off", Default {
              }
              frame "On" {
              }
              frame "Error" {
              }
            }
            n487 = Select(t=w1285, s=w1276, f=w1284) -> (s? t:f=w1280:errorcluster)
            n488 = Concatenate Strings("Primary Pump " ("string"), w1282) -> (w1283:string)
            n489 = Merge Errors(w1280, w1279) -> (w1277:errorcluster)
          }
          frame True {
            # "Ecodry"
            n490 = local read "Primary_Sys_Cmd"() -> (w1304:bool)
            n491 = Greater?(x=w1312, y=90.0) -> (0:w1303:bool)
            n492 = Select(t=enum16{"Off", "On", "Accelerating"}."Accelerating", s=w1304, f=enum16{"Off", "On", "Accelerating"}."Off") -> (s? t:f=w1300:enum16{"Off", "On", "Accelerating"})
            n493 = Select(t=enum16{"Off", "On", "Accelerating"}."On", s=w1303, f=w1300) -> (s? t:f=w1305:enum16{"Off", "On", "Accelerating"})
            n494 = case shown="\"Accelerating\"" w1305 {
              tunnel: [u32 12632256 ("Color") u32 6618880 ("Color") u32 3381759 ("Color")] -> w1308
              tunnel: ["is Off" "is On" "Accelerating"] -> w1310
              frame "Off", Default {
              }
              frame "On" {
              }
              frame "Accelerating" {
              }
            }
            n495 = Concatenate Strings("Primary Pump " ("string"), w1310) -> (w1307:string)
          }
        }
        "Primary Status" <- w1267
        "Primary Pump Status" <- w1248
        n496 = property on="Ecodry Speed" class="Str"("Visible"=w1102) -> ()  [unwired: 2 in, 2 out]
        n497 = Merge Errors(w1202, w1201, w1197, w1254, w1250, w1221, w1222, w1177, w1176) -> (w1255:errorcluster)
        n498 = Merge Errors(w1265, w1255) -> (w1266:errorcluster)
        "error out" <- w1265
        "Wide Range Gauge Pressure" <- w1164
        "Foreline Gauge" <- w1171
        "Primary_Pump_Read" <- w1226
        "Turbo 1 Gauge" <- w1170
        "Turbo 2 Gauge" <- w1169
        "Turbo 3 Gauge" <- w1168
        "Compressor Pressure (Bar)" <- w1091
        "Turbo on Threshold (torr) 3" <- w1093
      }
      frame #2 {
        # "Clear Errors?"
        # "Poll User Turbo Commands"
        # "Poll User Chiller Commands"
        # "Poll User Primary Pump Commands"
        # "Poll User Valve Commands"
        n499 = case shown="True" "Turbo_Reset_Cmd" {
          tunnel: w1414 -> [w1458 w1461]
          tunnel: [w1457 w1460] -> w1413
          tunnel: [FALSE ("Turbo_Reset_Cmd") w1459] -> w1410
          frame False {
            n500 = Bundle By Name(cluster=w1458, "Turbo Reset  SYS CMD"=FALSE) -> (w1457:T3)
          }
          frame True {
            n501 = call <vilib>:"Three Button Dialog.vi"("Right Button Text (\"Cancel\")"="No" ("Left Button Text (\"Yes\")"), "Center Button Text (\"No\")"="Yes, Reset  Both HiPaces" ("Left Button Text (\"Yes\")"), "Left Button Text (\"Yes\")"="Yes, Reset Shimadzu" ("Left Button Text (\"Yes\")"), "message"="Reset Turbo?") -> ("Which Button?"=w1462:T14)  [unwired: 7 in]
            n502 = case shown="\"Right Button\"" w1462 {
              tunnel: w1461 -> [w1470 w1472 w1474]
              tunnel: [w1469 w1472 w1474] -> w1460
              tunnel: [FALSE ("Turbo_Reset_Cmd") TRUE FALSE ("Turbo_Reset_Cmd")] -> w1459
              frame "Left Button", Default {
                n503 = Bundle By Name(cluster=w1470, "Turbo Reset  SYS CMD"=TRUE) -> (w1469:T3)
              }
              frame "Center Button" {
              }
              frame "Right Button" {
              }
            }
          }
        }
        n504 = case shown="False" "Clear error?" {
          tunnel: [w1475 w1476] -> w1426
          tunnel: w1427 -> [w1475 _]
          frame False {
          }
          frame True {
            n505 = call <vilib>:"Clear Errors.vi"() -> ("error out"=w1476:errorcluster)  [unwired: 6 in, 1 out]
          }
        }
        n506 = Wait (ms)(milliseconds to wait=u32 10) -> ()  [unwired: 1 out]
      }
      frame #3 {
        # "Turbo 3 Standby"
        # "Gate Cmd"
        # "Turbo 2 Standby"
        # "Turbo Standby\ncmd"
        # "Gate Valve\nRead"
        # "Turbo Motor\nRead"
        # "Turbo Speed\n(%)"
        # "Turbo 3 Motor\nCmd"
        # "Turbo Error\nAckn Cmd"
        # "Chiller \nCmd"
        # "Chiller \nRead"
        # "WRG Pressure (mBar)"
        # "Primary Pump\nCmd"
        # "Primary Pump\nRead"
        # "Vent Valve\nCmd"
        # "Bypass Valve\nCmd"
        # "Turbo_Valve\nCmd"
        # "Vent Valve\nRead"
        # "Bypass Valve\nRead"
        # "Turbo_Valve\nRead"
        # "Asses User Demands"
        n507 = Select(t=Facility_State."Admin", s="change_to_admin_mode", f=w1494) -> (s? t:f=w1495:T4)
        n508 = case shown="\"Auto\"" w1495 {
          selector: w1495 -> [w1620 _ _ w2135]
          tunnel: [w1556 FALSE ("Primary_User_Cmd") FALSE w2119] -> w1552
          tunnel: w1554 -> [w1628 _ _ w2126]
          tunnel: w1553 -> [w1625 _ _ w2106]
          tunnel: [w1625 errorcluster {"status"=FALSE, "code"=0, "source"=""} ("error out") errorcluster {"status"=FALSE, "code"=0, "source"=""} ("error out") w2106] -> w1551
          tunnel: w1550 -> [w1633 _ _ w2131]
          tunnel: w1549 -> [w1632 _ _ w2130]
          tunnel: w1548 -> [w1631 _ _ w2129]
          tunnel: [w1603 bool[] [FALSE, FALSE, FALSE] ("appended array") w1998 w2071] -> w1512
          tunnel: [w1607 FALSE ("Valve_Bypass_User_Cmd") FALSE ("Valve_Bypass_User_Cmd") w2121] -> w1547
          tunnel: [w1619 FALSE ("Valve_Vent_User_Cmd") FALSE ("Valve_Vent_User_Cmd") w2120] -> w1511
          tunnel: w1539 -> [w1626 _ _ w2124]
          tunnel: [w1555 FALSE ("Chiller_User_Cmd") FALSE ("Chiller_User_Cmd") w2014] -> w1538
          tunnel: w1537 -> [w1591 _ _ w2117]
          tunnel: [w1569 w1973 w1994 w2081] -> w1483
          tunnel: w1536 -> [w1577 _ _ w2015]
          tunnel: w1533 -> [_ _ _ w2096]
          tunnel: w1532 -> [_ _ _ w2134]
          tunnel: w1531 -> [_ _ _ w2133]
          tunnel: w1530 -> [_ _ _ w2127]
          tunnel: w1529 -> [_ _ _ w2116]
          tunnel: w1528 -> [_ _ _ w2092]
          tunnel: w1527 -> [_ _ _ w2125]
          tunnel: w1526 -> [w1557 _ _ w2118]
          tunnel: w1525 -> [_ _ _ w2123]
          tunnel: [TRUE ("Visible") FALSE ("Visible") FALSE ("Visible") FALSE ("Visible")] -> w1489
          tunnel: [w1601 bool[] [FALSE, FALSE, FALSE] ("appended array") w1998 w2072] -> w1524
          tunnel: w1523 -> [w1623 _ _ w2128]
          tunnel: w1522 -> [_ _ _ w2132]
          tunnel: w1521 -> [w1622 w1987 w2008 w2108]
          tunnel: [w1622 w1987 w2008 w2088] -> w1520
          tunnel: [w1609 w1986 w2007 w2135] -> w1507
          tunnel: [w1612 Current_Facility_State."Facility Off" Current_Facility_State."Facility Off" w2045] -> w1519
          tunnel: w1518 -> [_ _ _ w2112]
          tunnel: w1517 -> [_ _ _ w2111]
          tunnel: [w1614 Current_Facility_State."Facility Off" ("Facility Target State") Current_Facility_State."Facility Off" ("Facility Target State") w2052] -> w1516
          tunnel: w1515 -> [_ _ _ w2091]
          tunnel: w1514 -> [_ _ _ w2115]
          tunnel: [w1617 0 ("f") 0 ("f") w2114] -> w1513
          tunnel: w1488 -> [_ _ _ _]
          tunnel: w1487 -> [_ _ _ w2095]
          tunnel: w1486 -> [_ _ _ w2094]
          tunnel: [w1586 w1975 w1997 w2089] -> w1484
          tunnel: w1485 -> [w1585 _ w1997 w2093]
          tunnel: [w1576 w1973 w1994 w2035] -> w1482
          tunnel: w1481 -> [w1568 _ _ w2027]
          tunnel: [w1575 w1972 w1993 w2022] -> w1479
          tunnel: [w1570 w1972 w1993 w2016] -> w1480
          tunnel: [w1577 w1972 w1993 w2015] -> w1477
          frame "Admin" {
            w1561 = 15.0 ("y")
            (unwired) FALSE ("Turbo_Error_Acknowlege_Cmd")
            # "Turbo  Standby\nCmd"
            # "Turbo on?"
            # "go right into substate 2, if and only if you are going\n to primary pump down and bypass is open"
            # "Bypass"
            # "Turbo Valve"
            # "Vent"
            # "Gate"
            # "Enable Switches?"
            # "Read User Commands"
            n509 = Unbundle By Name(w1585) -> ("Turbo Motor SYS CMD"=w1592:bool, "Turbo Standby SYS CMD"=w1581:bool)
            n510 = local read "Turbo 2 Standby?"() -> (w1567:bool)
            n511 = local read "Turbo 3 Standby?"() -> (w1566:bool)
            n512 = Index Array(array=w1557, index=1) -> (element=w1563:dbl)
            n513 = Index Array(array=w1557, index=0) -> (element=w1562:dbl)
            n514 = Greater?(x=w1563, y=w1561) -> (0:w1559:bool)
            n515 = Greater?(x=w1562, y=w1561) -> (0:w1560:bool)
            n516 = Build Array(w1592, w1568, w1591) -> (w1590:bool[])
            n517 = Or(x=w1560, y=w1559) -> (x .or. y?=w1558:bool)
            n518 = Build Array("Turbo_1_Motor_User_Cmd", "Turbo_2_Motor_User_Cmd", "Turbo_3_Motor_User_Cmd") -> (w1593:bool[])
            n519 = Build Array(w1581, w1567, w1566) -> (w1580:bool[])
            n520 = Build Array("Valve_Gate_1_User_Cmd", "Valve_Gate_2_User_Cmd", "Valve_Gate_3_User_Cmd") -> (w1579:bool[])
            n521 = Build Array("Valve_Turbo_1_User_Cmd", "Valve_Turbo_2_User_Cmd", "Valve_Turbo_3_User_Cmd") -> (w1578:bool[])
            n522 = for {
              tunnel: w1593 -> [w1640] mode=indexing
              tunnel: w1590 -> [w1642] mode=indexing
              tunnel: [w1641] -> w1572 mode=indexing
              tunnel: [w1643] -> w1571 mode=indexing
              tunnel: w1580 -> [w1639] mode=indexing
              i -> [w1638]
              n523 = Increment(x=w1638) -> (x+1=w1637:i32)
              n524 = Number To Decimal String(number=w1637) -> (decimal integer string=w1636:string)  [unwired: 1 in]
              n525 = Concatenate Strings("Turbo " ("string"), w1636) -> (w1634:string)
              n526 = case shown="True" w1640 {
                tunnel: [w1645 w1650] -> w1641
                tunnel: w1642 -> [w1645 w1649]
                tunnel: [w1644 w1648] -> w1643
                tunnel: w1639 -> [w1644 w1646]
                tunnel: w1634 -> [_ w1647]
                frame False {
                }
                frame True {
                  n527 = case shown="True" w1649 {
                    tunnel: [w1655 w1659] -> w1650
                    tunnel: [FALSE w1658] -> w1648
                    tunnel: w1647 -> [_ w1657]
                    tunnel: w1646 -> [_ w1656]
                    frame False {
                      n528 = Two Button Dialog(message="Start Turbo Pump?", 1:"No" ("F button name (\"Cancel\")"), 2:"Yes" ("T button name (\"OK\")")) -> (T button?=w1655:bool)
                    }
                    frame True {
                      n529 = case shown="False" w1656 {
                        tunnel: [w1665 w1683] -> w1659
                        tunnel: [w1664 w1682] -> w1658
                        tunnel: w1657 -> [w1661 w1679]
                        frame False {
                          n530 = Concatenate Strings("Stop " ("string"), w1661, " Pump?" ("string")) -> (w1662:string)
                          n531 = call <vilib>:"Three Button Dialog.vi"("Right Button Text (\"Cancel\")"=" Activate Standby" ("Right Button Text (\"Cancel\")"), "Center Button Text (\"No\")"="No" ("Center Button Text (\"No\")"), "Left Button Text (\"Yes\")"="Yes" ("Left Button Text (\"Yes\")"), "message"=w1662) -> ("Which Button?"=w1666:T14)  [unwired: 7 in]
                          n532 = case shown="\"Window Close\"" w1666 {
                            tunnel: [FALSE TRUE TRUE TRUE] -> w1665
                            tunnel: [FALSE FALSE TRUE FALSE] -> w1664
                            frame "Left Button" {
                            }
                            frame "Center Button", Default {
                            }
                            frame "Right Button" {
                            }
                            frame "Window Close" {
                            }
                          }
                        }
                        frame True {
                          n533 = Concatenate Strings(" Exit " ("string"), w1679, " Standby Mode? " ("string")) -> (w1678:string)
                          n534 = call <vilib>:"Three Button Dialog.vi"("Right Button Text (\"Cancel\")"=" Yes, Spin Down" ("Right Button Text (\"Cancel\")"), "Center Button Text (\"No\")"="No" ("Center Button Text (\"No\")"), "Left Button Text (\"Yes\")"="Yes, Spin Up" ("Left Button Text (\"Yes\")"), "message"=w1678) -> ("Which Button?"=w1684:T14)  [unwired: 7 in]
                          n535 = case shown="\"Center Button\", Default" w1684 {
                            tunnel: [TRUE TRUE FALSE TRUE] -> w1683
                            tunnel: [FALSE TRUE FALSE TRUE] -> w1682
                            frame "Left Button" {
                            }
                            frame "Center Button", Default {
                            }
                            frame "Right Button" {
                            }
                            frame "Window Close" {
                            }
                          }
                        }
                      }
                    }
                  }
                }
              }
            }
            n536 = for {
              tunnel: w1633 -> [w1726] mode=indexing
              tunnel: [w1725] -> w1603 mode=indexing
              tunnel: w1578 -> [w1724] mode=indexing
              i -> [w1722]
              n537 = Increment(x=w1722) -> (x+1=w1721:i32)
              n538 = Number To Decimal String(number=w1721) -> (decimal integer string=w1723:string)  [unwired: 1 in]
              n539 = case shown="True" w1724 {
                tunnel: [w1727 w1730] -> w1725
                tunnel: w1726 -> [w1727 w1729]
                tunnel: w1723 -> [_ w1728]
                frame False {
                }
                frame True {
                  n540 = case shown="False" w1729 {
                    tunnel: [w1737 w1742] -> w1730
                    tunnel: w1728 -> [w1731 w1738]
                    frame False {
                      n541 = Concatenate Strings("Open Turbo " ("string"), w1731, " Valve?" ("string")) -> (w1732:string)
                      n542 = Two Button Dialog(message=w1732, 1:"No" ("F button name (\"Cancel\")"), 2:"Yes" ("T button name (\"OK\")")) -> (T button?=w1737:bool)
                    }
                    frame True {
                      n543 = Concatenate Strings("Close Turbo " ("string"), w1738, " Valve?" ("string")) -> (w1739:string)
                      n544 = Two Button Dialog(message=w1739, 1:"No" ("F button name (\"Cancel\")"), 2:"Yes" ("T button name (\"OK\")")) -> (T button?=w1743:bool)
                      n545 = Not(x=w1743) -> (.not. x?=w1742:bool)
                    }
                  }
                }
              }
            }
            n546 = for {
              tunnel: w1623 -> [w1701] mode=indexing
              tunnel: [w1700] -> w1601 mode=indexing
              tunnel: w1579 -> [w1696] mode=indexing
              i -> [w1699]
              n547 = Increment(x=w1699) -> (x+1=w1697:i32)
              n548 = Number To Decimal String(number=w1697) -> (decimal integer string=w1698:string)  [unwired: 1 in]
              n549 = case shown="True" w1696 {
                tunnel: [w1702 w1704] -> w1700
                tunnel: w1701 -> [w1702 w1703]
                tunnel: w1698 -> [_ w1705]
                frame False {
                }
                frame True {
                  n550 = case shown="False" w1703 {
                    tunnel: [w1712 w1717] -> w1704
                    tunnel: w1705 -> [w1709 w1716]
                    frame False {
                      n551 = Concatenate Strings("Open Gate " ("string"), w1709, " Valve" ("string")) -> (w1706:string)
                      n552 = Two Button Dialog(message=w1706, 1:"No" ("F button name (\"Cancel\")"), 2:"Yes" ("T button name (\"OK\")")) -> (T button?=w1712:bool)
                    }
                    frame True {
                      n553 = Concatenate Strings("Close Gate " ("string"), w1716, " Valve?" ("string")) -> (w1713:string)
                      n554 = Two Button Dialog(message=w1713, 1:"No" ("F button name (\"Cancel\")"), 2:"Yes" ("T button name (\"OK\")")) -> (T button?=w1718:bool)
                      n555 = Not(x=w1718) -> (.not. x?=w1717:bool)
                    }
                  }
                }
              }
            }
            n556 = case shown="True" "Valve_Bypass_User_Cmd" {
              tunnel: [w1959 w1961] -> w1607
              tunnel: w1632 -> [w1959 w1960]
              frame False {
              }
              frame True {
                n557 = case shown="False" w1960 {
                  tunnel: [w1965 w1966] -> w1961
                  frame False {
                    n558 = Two Button Dialog(message="Open Bypass Valve?", 1:"No" ("F button name (\"Cancel\")"), 2:"Yes" ("T button name (\"OK\")")) -> (T button?=w1965:bool)
                  }
                  frame True {
                    n559 = Two Button Dialog(message="Close Bypass Valve?", 1:"No" ("F button name (\"Cancel\")"), 2:"Yes" ("T button name (\"OK\")")) -> (T button?=w1967:bool)
                    n560 = Not(x=w1967) -> (.not. x?=w1966:bool)
                  }
                }
              }
            }
            n561 = case shown="True" "Valve_Vent_User_Cmd" {
              tunnel: [w1947 w1949] -> w1619
              tunnel: w1631 -> [w1947 w1948]
              frame False {
              }
              frame True {
                n562 = case shown="False" w1948 {
                  tunnel: [w1953 w1954] -> w1949
                  frame False {
                    n563 = Two Button Dialog(message="Open Vent Valve?", 1:"No" ("F button name (\"Cancel\")"), 2:"Yes" ("T button name (\"OK\")")) -> (T button?=w1953:bool)
                  }
                  frame True {
                    n564 = Two Button Dialog(message="Close Vent Valve?", 1:"No" ("F button name (\"Cancel\")"), 2:"Yes" ("T button name (\"OK\")")) -> (T button?=w1955:bool)
                    n565 = Not(x=w1955) -> (.not. x?=w1954:bool)
                  }
                }
              }
            }
            n566 = case shown="True" "Primary_User_Cmd" {
              tunnel: [w1935 w1937] -> w1556
              tunnel: w1628 -> [w1935 w1936]
              frame False {
              }
              frame True {
                n567 = case shown="True" w1936 {
                  tunnel: [w1941 w1942] -> w1937
                  frame False {
                    n568 = Two Button Dialog(message="Turn on Primary Pump?", 1:"No" ("F button name (\"Cancel\")"), 2:"Yes" ("T button name (\"OK\")")) -> (T button?=w1941:bool)
                  }
                  frame True {
                    n569 = Two Button Dialog(message="Turn Off Primary Pump?", 1:"No" ("F button name (\"Cancel\")"), 2:"Yes" ("T button name (\"OK\")")) -> (T button?=w1943:bool)
                    n570 = Not(x=w1943) -> (.not. x?=w1942:bool)
                  }
                }
              }
            }
            n571 = case shown="True" "Chiller_User_Cmd" {
              tunnel: [w1923 w1925] -> w1555
              tunnel: w1626 -> [w1923 w1924]
              frame False {
              }
              frame True {
                n572 = case shown="True" w1924 {
                  tunnel: [w1929 w1930] -> w1925
                  frame False {
                    n573 = Two Button Dialog(message="Turn on Chiller?", 1:"No" ("F button name (\"Cancel\")"), 2:"Yes" ("T button name (\"OK\")")) -> (T button?=w1929:bool)
                  }
                  frame True {
                    n574 = Two Button Dialog(message="Turn Off Chiller?", 1:"No" ("F button name (\"Cancel\")"), 2:"Yes" ("T button name (\"OK\")")) -> (T button?=w1931:bool)
                    n575 = Not(x=w1931) -> (.not. x?=w1930:bool)
                  }
                }
              }
            }
            n576 = local read "Index_of_working_turbo"() -> (w1602:i32)
            n577 = Index Array(array=w1572, index=0) -> (element=w1587:bool)
            n578 = Index Array(array=w1571, index=0) -> (element=w1582:bool)
            n579 = Index Array(array=w1572, index=1) -> (element=w1576:bool)
            n580 = Index Array(array=w1571, index=1) -> (element=w1575:bool)
            n581 = Index Array(array=w1572, index=2) -> (element=w1569:bool)
            n582 = case shown="True" "Change to Auto" {
              tunnel: w1556 -> [_ w1784]
              tunnel: w1620 -> [w1748 _]
              tunnel: [w1748 w1773] -> w1609
              tunnel: [Current_Facility_State."Facility Off" w1775] -> w1612
              tunnel: [Current_Facility_State."Facility Off" w1777] -> w1614
              tunnel: w1569 -> [_ w1783]
              tunnel: w1558 -> [_ w1782]
              tunnel: w1603 -> [_ w1766]
              tunnel: w1601 -> [_ w1781]
              tunnel: w1619 -> [_ w1780]
              tunnel: w1607 -> [_ w1768]
              tunnel: w1602 -> [_ w1758]
              tunnel: w1601 -> [_ w1753]
              frame False {
                (unwired) FALSE ("Keep Primary On While venting?")
              }
              frame True {
                # "All  Gate  valves Closed"
                # "All used Gate  valves Open"
                # "All  Turbo  valves Closed"
                # "All used Turbo  valves Open"
                # "Ask to Switch?"
                # "Primary on?"
                n583 = Index Array(array=w1766, index=w1758) -> (element=w1760:bool)
                n584 = Index Array(array=w1781, index=w1758) -> (element=w1759:bool)
                n585 = local read "Which_Turbos_used?"() -> (w1752:bool[])
                n586 = case shown="True" w1784 {
                  tunnel: w1783 -> [w1801 w1822]
                  tunnel: w1782 -> [_ _]
                  tunnel: [w1812 w1829] -> w1776
                  tunnel: [w1811 w1828] -> w1778
                  tunnel: [w1810 w1827] -> w1779
                  tunnel: w1760 -> [w1799 w1824]
                  tunnel: w1759 -> [w1808 w1821]
                  tunnel: w1780 -> [w1807 w1826]
                  tunnel: [w1809 w1825] -> w1762
                  tunnel: w1768 -> [w1806 w1823]
                  frame False {
                    # "Must be facility off, lets check"
                    n587 = Not(x=w1799) -> (.not. x?=w1805:bool)
                    n588 = Not(x=w1807) -> (.not. x?=w1803:bool)
                    n589 = Not(x=w1808) -> (.not. x?=w1804:bool)
                    n590 = Not(x=w1806) -> (.not. x?=w1802:bool)
                    n591 = Not(x=w1801) -> (.not. x?=w1800:bool)
                    n592 = Compound Arithmetic op=AND(w1800, w1805, w1804, w1803, w1802) -> (w1798:bool)
                    n593 = case shown="True" w1798 {
                      tunnel: [Current_Facility_State."Facility Off" Current_Facility_State."Facility Off"] -> w1812
                      tunnel: [Current_Facility_State."Facility Off" Current_Facility_State."Facility Off"] -> w1811
                      tunnel: ["" "Facility off"] -> w1810
                      tunnel: [FALSE TRUE] -> w1809
                      frame False {
                      }
                      frame True {
                      }
                    }
                  }
                  frame True {
                    # "Gate open?"
                    n594 = case shown="False" w1821 {
                      selector: w1821 -> [w1833 w1909]
                      tunnel: [w1838 w1914] -> w1829
                      tunnel: [w1837 w1913] -> w1828
                      tunnel: [w1836 w1912] -> w1827
                      tunnel: w1826 -> [w1830 w1908]
                      tunnel: [w1835 w1911] -> w1825
                      tunnel: w1824 -> [w1834 w1910]
                      tunnel: w1823 -> [w1832 w1906]
                      tunnel: w1822 -> [w1831 _]
                      frame False {
                        # "Turbo On?"
                        n595 = case shown="True" w1831 {
                          selector: w1831 -> [w1843 _]
                          tunnel: [w1849 w1865] -> w1838
                          tunnel: [w1848 w1864] -> w1837
                          tunnel: [w1847 w1863] -> w1836
                          tunnel: [w1846 w1862] -> w1835
                          tunnel: w1834 -> [w1841 w1860]
                          tunnel: w1833 -> [w1845 w1859]
                          tunnel: w1832 -> [_ w1861]
                          tunnel: w1830 -> [_ w1858]
                          frame False {
                            # "Must be Pumping to rough,\nlets check:"
                            n596 = Not(x=w1843) -> (.not. x?=w1842:bool)
                            n597 = Not(x=w1845) -> (.not. x?=w1844:bool)
                            n598 = Not(x=w1841) -> (.not. x?=w1840:bool)
                            n599 = Compound Arithmetic op=AND(w1840, w1844, w1842) -> (w1839:bool)
                            n600 = case shown="True" w1839 {
                              tunnel: [Current_Facility_State."Facility Off" Current_Facility_State."Pumping to Rough"] -> w1849
                              tunnel: [Current_Facility_State."Facility Off" Current_Facility_State."Pumping to High Vac"] -> w1848
                              tunnel: ["" "Pumping to Rough"] -> w1847
                              tunnel: [FALSE ("Keep Primary On While venting?") TRUE ("Keep Primary On While venting?")] -> w1846
                              frame False {
                              }
                              frame True {
                                # "If bypass open, skip warm up"
                              }
                            }
                          }
                          frame True {
                            # "Is the bypass open?"
                            n601 = case shown="True" w1861 {
                              selector: w1861 -> [w1869 w1887]
                              tunnel: [w1875 w1895] -> w1865
                              tunnel: [w1874 w1894] -> w1864
                              tunnel: [w1873 w1893] -> w1863
                              tunnel: [w1872 w1892] -> w1862
                              tunnel: w1860 -> [w1871 w1886]
                              tunnel: w1859 -> [w1870 w1891]
                              tunnel: w1858 -> [_ w1889]
                              frame False {
                                # "Must be venting, Lets Check:"
                                n602 = Not(x=w1870) -> (.not. x?=w1868:bool)
                                n603 = Not(x=w1869) -> (.not. x?=w1867:bool)
                                n604 = Compound Arithmetic op=AND(w1871, w1868, w1867) -> (w1866:bool)
                                n605 = case shown="True" w1866 {
                                tunnel: [Current_Facility_State."Facility Off" Current_Facility_State."Venting"] -> w1875
                                tunnel: [Current_Facility_State."Facility Off" Current_Facility_State."Venting"] -> w1874
                                tunnel: ["0" "Venting"] -> w1873
                                tunnel: [FALSE ("Keep Primary On While venting?") TRUE ("Keep Primary On While venting?")] -> w1872
                                frame False {
                                }
                                frame True {
                                }
                                }
                              }
                              frame True {
                                # "Must be pumping to Rough,\n Lets check:"
                                n606 = Not(x=w1891) -> (.not. x?=w1890:bool)
                                n607 = Not(x=w1886) -> (.not. x?=w1885:bool)
                                n608 = Not(x=w1889) -> (.not. x?=w1888:bool)
                                n609 = Compound Arithmetic op=AND(w1885, w1890, w1888, w1887) -> (w1884:bool)
                                n610 = case shown="True" w1884 {
                                tunnel: [Current_Facility_State."Facility Off" Current_Facility_State."Pumping to Rough"] -> w1895
                                tunnel: [Current_Facility_State."Facility Off" Current_Facility_State."Pumping to High Vac"] -> w1894
                                tunnel: ["" "Pumping to Rough"] -> w1893
                                tunnel: [FALSE ("Keep Primary On While venting?") TRUE ("Keep Primary On While venting?")] -> w1892
                                frame False {
                                }
                                frame True {
                                }
                                }
                              }
                            }
                          }
                        }
                      }
                      frame True {
                        # "Must be Hi Vac, lets check:"
                        n611 = Not(x=w1908) -> (.not. x?=w1907:bool)
                        n612 = Not(x=w1906) -> (.not. x?=w1905:bool)
                        n613 = Compound Arithmetic op=AND(w1910, w1909, w1907, w1905) -> (w1904:bool)
                        n614 = case shown="False" w1904 {
                          tunnel: [Current_Facility_State."Facility Off" Current_Facility_State."Pumping to High Vac"] -> w1914
                          tunnel: [Current_Facility_State."Facility Off" Current_Facility_State."Pumping to High Vac"] -> w1913
                          tunnel: ["" "Pumping to High Vac"] -> w1912
                          tunnel: [FALSE ("Keep Primary On While venting?") TRUE ("Keep Primary On While venting?")] -> w1911
                          frame False {
                          }
                          frame True {
                          }
                        }
                      }
                    }
                  }
                }
                n615 = Not(x=w1766) -> (.not. x?=w1765:bool[])
                n616 = Not Exclusive Or(1:w1752, 2:w1766) -> (0:w1767:bool[])
                n617 = Not(x=w1753) -> (.not. x?=w1755:bool[])
                n618 = Not Exclusive Or(1:w1752, 2:w1753) -> (0:w1754:bool[])
                n619 = And Array Elements(Boolean array=w1765) -> (logical AND=w1764:bool)
                n620 = And Array Elements(Boolean array=w1767) -> (logical AND=w1763:bool)
                n621 = And Array Elements(Boolean array=w1755) -> (logical AND=w1756:bool)
                n622 = And Array Elements(Boolean array=w1754) -> (logical AND=w1757:bool)
                n623 = Or(x=w1763, y=w1764) -> (x .or. y?=w1750:bool)
                n624 = Or(x=w1757, y=w1756) -> (x .or. y?=w1751:bool)
                n625 = And(x=w1750, y=w1751) -> (x .and. y?=w1749:bool)
                n626 = And(x=w1762, y=w1749) -> (x .and. y?=w1761:bool)
                n627 = case shown="False" w1761 {
                  tunnel: w1779 -> [_ w1796]
                  tunnel: [Current_Facility_State."Facility Off" ("f") Current_Facility_State."Facility Off" ("f")] -> w1770
                  tunnel: [FALSE ("T button?") w1790] -> w1769
                  frame False {
                    n628 = call "Display Message to User"("Message"="Target State Not Recognised! " ("string")) -> ()  [unwired: 9 in, 2 out]
                  }
                  frame True {
                    n629 = Concatenate Strings("Go to State: " ("string"), "\r", "\"" ("string"), w1796, "\"?" ("string")) -> (w1794:string)
                    n630 = Two Button Dialog(message=w1794, 1:"No" ("F button name (\"Cancel\")"), 2:"Yes" ("T button name (\"OK\")")) -> (T button?=w1790:bool)
                  }
                }
                n631 = Select(t=w1776, s=w1769, f=Current_Facility_State."Facility Off") -> (s? t:f=w1775:T1)
                n632 = Select(t=w1778, s=w1769, f=w1770) -> (s? t:f=w1777:T1)
                n633 = Select(t=Facility_State."Auto", s=w1769, f=Facility_State."Admin") -> (s? t:f=w1773:T4)
              }
            }
            n634 = Index Array(array=w1571, index=2) -> (element=w1570:bool)
            n635 = Bundle By Name(cluster=w1585, "Turbo Motor SYS CMD"=w1587, "Turbo Standby SYS CMD"=w1582) -> (w1586:T3)
            n636 = Equal?(x=w1612, y=Current_Facility_State."Pumping to Rough") -> (x = y?=w1611:bool)
            n637 = Equal?(x=w1609, y=Facility_State."Auto") -> (x = y?=w1610:bool)
            n638 = Compound Arithmetic op=AND(w1610, w1611, w1607) -> (w1615:bool)
            n639 = Select(t=2, s=w1615, f=0) -> (s? t:f=w1617:i32)
          }
          frame "Intialize" {
            w1972 = FALSE ("Turbo_Motor_User_Cmd")
            w1975 = T3 {"Turbo Rotating Read"=FALSE, "Turbo Accelarating Read"=FALSE, "Turbo At Speed Read"=FALSE, "Turbo Breaking Read"=FALSE, "Turbo Alarm Read"=FALSE, "Turbo Warning Read"=FALSE, "Turbo Motor SYS CMD"=FALSE, "Turbo Standby SYS CMD"=FALSE, "Turbo Reset  SYS CMD"=FALSE}  # Defualt Turbo Cluseter
            w1973 = FALSE ("Turbo_Motor_User_Cmd")
            # "Enable Switches?"
            n640 = Two Button Dialog(message="Select Control Mode", 1:"Admin" ("Center Button Text (\"No\")"), 2:"Auto" ("Right Button Text (\"Cancel\")")) -> (T button?=w1980:bool)
            n641 = case shown="True" w1980 {
              tunnel: [Facility_State."Admin" Facility_State."Auto"] -> w1986
              frame False {
              }
              frame True {
              }
            }
          }
          frame "Manual" {
            w1998 = bool[] [FALSE, FALSE, FALSE] ("appended array")
            w1993 = FALSE
            (unwired) FALSE ("T button?")
            (unwired) FALSE ("Primary_User_Cmd")
            (unwired) FALSE ("Turbo_Error_Acknowlege_Cmd")
            w1994 = FALSE ("Turbo_Motor_User_Cmd")
            (unwired) FALSE ("Valve_Turbo_User_Cmd")
            # "Enable Switches?"
            n642 = Two Button Dialog(message="Select Control Mode", 1:"Admin" ("Center Button Text (\"No\")"), 2:"Auto" ("Right Button Text (\"Cancel\")")) -> (T button?=w2001:bool)
            n643 = case shown="True" w2001 {
              tunnel: [Facility_State."Admin" Facility_State."Auto"] -> w2007
              frame False {
              }
              frame True {
              }
            }
          }
          frame "Auto" {
            w2109 = Current_Facility_State."Facility Off" ("t")
            # "Go to blank \"Holding at rough\"\npage for a few seconds between \nstate changes"
            # "Foreline\nConvectron\n(mBar)"
            # "Turbo\nConvectron\n(mBar)"
            # "Sub_state_iteration"
            # "Turbo valve control"
            # "Bypass control"
            # "Vent control"
            # "Gate control"
            # "Command Primary"
            # "Command Chiller"
            # "Enable admin Switches?"
            n644 = call <vilib>:"Simple Error Handler.vi"("error in (no error)"=w2106) -> ("code out"=w2103:i32)  [unwired: 4 in, 4 out]
            n645 = Greater Or Equal?(x=w2103, y=5000) -> (x >= y?=w2104:bool)
            n646 = Less Or Equal?(x=w2103, y=5010) -> (x <= y?=w2101:bool)
            n647 = And(x=w2104, y=w2101) -> (x .and. y?=w2100:bool)
            n648 = call <vilib>:"Simple Error Handler.vi"("error in (no error)"=w2106) -> ("error?"=w2099:bool)  [unwired: 4 in, 4 out]
            n649 = Or(x=w2100, y=w2099) -> (x .or. y?=w2097:bool)
            n650 = case shown="True" w2097 {
              tunnel: w2108 -> [w2163 w2169]
              tunnel: [w2163 w2168] -> w2107
              frame False {
              }
              frame True {
                n651 = Get Date/Time String(want seconds? (F)=TRUE) -> (time string=w2164:string)  [unwired: 2 in, 1 out]
                n652 = Concatenate Strings(w2169, "\r", "Shutt down due to error at " ("string"), w2164) -> (w2168:string)
              }
            }
            n653 = Select(t=w2109, s=w2097, f=w2111) -> (s? t:f=w2110:T1)
            n654 = Select(t=w2109, s=w2097, f=w2112) -> (s? t:f=w2048:T1)
            n655 = call "Is Value Changed.vim"("value"=w2048) -> ("changed or first call?"=→"New_State?":bool)
            n656 = case shown="\"Pumping to Rough\"" w2048 {
              tunnel: w2096 -> [_ _ _ _ _ _ _ _]
              tunnel: w2134 -> [_ _ _ _ _ _ _ _]
              tunnel: w2133 -> [_ _ _ _ _ _ _ _]
              tunnel: w2132 -> [_ _ _ _ _ _ _ _]
              tunnel: w2131 -> [_ w2328 _ _ _ _ w2767 w2898]
              tunnel: w2130 -> [_ w2309 _ _ _ _ _ _]
              tunnel: w2129 -> [_ _ _ _ _ _ _ _]
              tunnel: w2128 -> [_ _ _ _ _ _ _ _]
              tunnel: w2127 -> [_ w2311 _ _ _ _ _ _]
              tunnel: w2126 -> [_ _ _ _ _ _ _ _]
              tunnel: w2125 -> [_ _ _ _ _ _ _ _]
              tunnel: w2124 -> [_ _ _ _ _ _ _ _]
              tunnel: w2123 -> [_ _ _ _ _ _ _ _]
              tunnel: [bool[] [FALSE, FALSE, FALSE] w2306 w2436 w2482 w2634 w2672 w2796 w2913] -> w2122
              tunnel: [FALSE ("Valve_Bypass_User_Cmd") w2322 FALSE ("Valve_Bypass_User_Cmd") w2497 FALSE ("Valve_Bypass_User_Cmd") w2675 FALSE ("Valve_Bypass_User_Cmd") FALSE ("Valve_Bypass_User_Cmd")] -> w2121
              tunnel: [FALSE ("Valve_Vent_User_Cmd") FALSE ("Valve_Vent_User_Cmd") FALSE ("Valve_Vent_User_Cmd") FALSE ("Valve_Vent_User_Cmd") FALSE ("Valve_Vent_User_Cmd") FALSE ("Valve_Vent_User_Cmd") w2766 FALSE ("t")] -> w2120
              tunnel: [FALSE ("Primary_User_Cmd") TRUE ("Primary_User_Cmd") w2438 TRUE ("Primary_User_Cmd") TRUE ("Primary_User_Cmd") TRUE ("Primary_User_Cmd") w2743 TRUE ("Primary_User_Cmd")] -> w2119
              tunnel: [FALSE ("Chiller_User_Cmd") w2233 w2438 TRUE ("Chiller_User_Cmd") TRUE ("Chiller_User_Cmd") TRUE ("Chiller_User_Cmd") w2743 TRUE ("Chiller_User_Cmd")] -> w2014
              tunnel: [w2218 w2332 w2434 w2494 w2639 w2678 w2825 w2904] -> w2045
              tunnel: w2110 -> [w2226 w2246 w2453 _ w2655 w2677 w2835 _]
              tunnel: [w2213 w2334 w2457 w2487 w2641 w2676 w2830 w2916] -> w2052
              tunnel: w2118 -> [_ w2241 w2413 w2486 _ _ w2748 w2876]
              tunnel: w2117 -> [_ w2298 _ w2485 _ w2683 w2793 _]
              tunnel: [w2185 w2289 w2410 w2495 w2626 w2673 w2792 w2873] -> w2017
              tunnel: w2091 -> [_ _ _ w2492 _ _ _ _]
              tunnel: w2116 -> [_ w2286 _ w2493 _ _ _ _]
              tunnel: w2092 -> [_ _ _ w2491 _ _ w2772 w2899]
              tunnel: w2115 -> [_ w2314 _ w2498 _ w2681 w2775 w2882]
              tunnel: [0 ("Sub_state_iteration") w2331 0 ("Sub_state_iteration") w2490 0 ("f") w2680 w2827 w2892] -> w2114
              tunnel: w2107 -> [w2215 w2342 w2448 w2489 w2661 w2679 w2840 w2924]
              tunnel: [w2215 w2342 w2447 w2488 w2661 w2679 w2840 w2924] -> w2098
              tunnel: [T2."Facility Off" ("Tab Control") T2."Pumping to Rough" ("Tab Control") T2."Overnight Pump" ("Tab Control") T2."Engaging Turbo" ("Tab Control") T2."Pumping to Hig Vac" ("Tab Control") T2."Closing Gate" ("Tab Control") T2."Venting" ("Tab Control") T2."Turbo Slowing" ("Tab Control")] -> w2042
              tunnel: w2095 -> [_ _ _ _ _ _ _ _]
              tunnel: [bool[] [FALSE, FALSE, FALSE] bool[] [FALSE, FALSE, FALSE] ("appended array") bool[] [FALSE, FALSE, FALSE] ("appended array") w2479 w2631 w2671 bool[] [FALSE, FALSE, FALSE] ("appended array") bool[] [FALSE, FALSE, FALSE] ("appended array")] -> w2032
              tunnel: w2094 -> [_ w2299 _ _ _ _ w2773 w2900]
              tunnel: w2093 -> [_ w2297 w2442 w2478 w2630 w2670 w2794 w2922]
              tunnel: [w2209 w2290 w2442 w2477 w2629 w2669 w2791 w2921] -> w2090
              tunnel: w2027 -> [_ w2237 _ w2475 _ w2668 w2745 _]
              tunnel: [w2185 w2235 w2410 w2476 w2598 w2667 w2746 w2873] -> w2026
              frame "Facility Off", Default {
                w2209 = T3 {"Turbo Rotating Read"=FALSE, "Turbo Accelarating Read"=FALSE, "Turbo At Speed Read"=FALSE, "Turbo Breaking Read"=FALSE, "Turbo Alarm Read"=FALSE, "Turbo Warning Read"=FALSE, "Turbo Motor SYS CMD"=FALSE, "Turbo Standby SYS CMD"=FALSE, "Turbo Reset  SYS CMD"=FALSE}  # Defualt Turbo Cluseter
                w2185 = FALSE ("Turbo_Error_Acknowlege_Cmd")
                n657 = local read "New_State?"() -> (w2202:bool)
                n658 = Select(t=FALSE, s=w2202, f="Pump to Rough") -> (s? t:f=w2205:bool)
                n659 = Select(t=Current_Facility_State."Pumping to Rough", s=w2205, f=w2226) -> (s? t:f=w2224:T1)
                n660 = local read "New_State?"() -> (w2201:bool)
                n661 = Select(t=FALSE, s=w2201, f="Pump to High Vac") -> (s? t:f=w2198:bool)
                n662 = Select(t=Current_Facility_State."Pumping to High Vac", s=w2198, f=w2224) -> (s? t:f=w2221:T1)
                n663 = local read "New_State?"() -> (w2196:bool)
                n664 = Select(t=FALSE, s=w2196, f="Overnight Pump") -> (s? t:f=w2194:bool)
                n665 = Select(t=Current_Facility_State."Overnight Pump", s=w2194, f=w2221) -> (s? t:f=w2208:T1)
                n666 = local read "New_State?"() -> (w2193:bool)
                n667 = Select(t=FALSE, s=w2193, f="Shut Off once rough 2") -> (s? t:f=w2190:bool)
                n668 = Compound Arithmetic op=OR(w2205, w2198, w2194, w2190) -> (w2227:bool)
                n669 = Select(t=Current_Facility_State."Facility Off", s=w2190, f=w2208) -> (s? t:f=w2207:T1)
                n670 = Select(t=Current_Facility_State."Pumping to Rough", s=w2227, f=Current_Facility_State."Facility Off") -> (s? t:f=w2219:T1)
                n671 = local read "New_State?"() -> (w2189:bool)
                n672 = Select(t=FALSE, s=w2189, f="Vent") -> (s? t:f=w2186:bool)
                n673 = Select(t=Current_Facility_State."Venting", s=w2186, f=w2219) -> (s? t:f=w2218:T1)
                n674 = Select(t=Current_Facility_State."Vent and Shutdown", s=w2186, f=w2207) -> (s? t:f=w2213:T1)
              }
              frame "Pumping to Rough" {
                w2254 = Current_Facility_State."Facility Off" ("y")
                w2285 = 5.0  # Turbo_hot_start_threshold_(mbar)
                w2239 = 15.0 ("y")
                # "Hot Start Turbo?"
                # "Time long enough"
                # "Foreline\nConvectron\n(mBar)"
                # "Open if lower, then keep open"
                # "For 10 mins"
                # "Turbo spinning?"
                # "Turn on Chiller?"
                n675 = Unbundle By Name(w2297) -> ("Turbo Rotating Read"=w2323:bool)
                n676 = Index Array(array=w2241, index=1) -> (element=w2242:dbl)
                n677 = Index Array(array=w2241, index=0) -> (element=w2240:dbl)
                n678 = Greater?(x=w2242, y=w2239) -> (0:w2330:bool)
                n679 = Greater?(x=w2240, y=w2239) -> (0:w2238:bool)
                n680 = Compound Arithmetic op=OR(w2323, w2238, w2330) -> (w2232:bool)
                n681 = Equal?(x=0, y=w2314) -> (x = y?=w2310:bool)
                n682 = call "Elapsed Time3"("Time Target (s)"=20.0, "Reset"=w2310, "Auto Reset"=FALSE) -> ("Time has Elapsed"=w2318:bool)  [unwired: 9 in, 7 out]
                n683 = And(x=w2310, y=w2311) -> (x .and. y?=w2308:bool)
                n684 = Compound Arithmetic op=OR(w2318, w2308) -> (w2317:bool)
                n685 = case shown="2" w2314 {
                  tunnel: [w2374 w2382 2] -> w2313
                  tunnel: w2317 -> [_ w2379 _]
                  tunnel: [w2376 w2379 TRUE] -> w2316
                  tunnel: [FALSE ("Time has Elapsed") FALSE ("Time has Elapsed") w2386] -> w2281
                  tunnel: w2308 -> [w2373 _ _]
                  tunnel: w2286 -> [_ _ w2383]
                  frame 0, Default {
                    (unwired) 2 ("t")
                    (unwired) TRUE ("Skip Primary Warm")
                    w2371 = FALSE ("Skip Primary Warm")
                    n686 = Select(t=1, s=w2373, f=1 ("Sub_state_iteration")) -> (s? t:f=w2374:i32)
                    n687 = Select(t=w2371, s=w2373, f=w2371) -> (s? t:f=w2376:bool)
                  }
                  frame 1 {
                    n688 = Select(t=2, s=w2379, f=1 ("Sub_state_iteration")) -> (s? t:f=w2382:i32)
                  }
                  frame 2 {
                    w2388 = 30.0  # Min time below threshhold (s)
                    # "And turbo valve open"
                    # "Drop below threshold long enough"
                    # "Foreline Pressure Reached?"
                    # "WRG Pressure reached?"
                    n689 = Less?(x=w2383, y="Turbo on Threshold (torr) 2") -> (x < y?=w2385:bool)
                    n690 = call "Is Value Changed.vim"("value"=w2385) -> ("changed or first call?"=w2390:bool)
                    n691 = case shown="True" w2385 {
                      tunnel: w2390 -> [_ w2398]
                      tunnel: [FALSE ("Time has Elapsed") w2396] -> w2386
                      tunnel: [0.0 ("Elapsed Time (s)") w2394] -> w2389
                      tunnel: w2388 -> [_ w2395]
                      frame False {
                      }
                      frame True {
                        n692 = call "Elapsed Time"("Time Target (s)"=w2395, "Reset"=w2398, "Auto Reset"=FALSE) -> ("Elapsed Time (s)"=w2394:dbl, "Time has Elapsed"=w2396:bool)  [unwired: 9 in, 6 out]
                      }
                    }
                    "Elapsed Time (s)" <- w2389
                    "Turbo on Threshold (torr)" <- "Turbo on Threshold (torr) 2"
                  }
                }
                n693 = Equal?(x=Current_Facility_State."Overnight Pump", y=w2246) -> (x = y?=w2296:bool)
                n694 = Compound Arithmetic op=OR(w2232, w2310) -> (w2249:bool)
                n695 = And(x=w2281, y=w2296) -> (x .and. y?=w2349:bool)
                n696 = Select(t=Current_Facility_State."Overnight Pump" ("x"), s=w2349, f=Current_Facility_State."Pumping to Rough") -> (s? t:f=w2345:T1)
                n697 = Equal?(x=w2246, y=Current_Facility_State."Pumping to Rough") -> (x = y?=w2294:bool)
                n698 = Equal?(x=w2246, y=Current_Facility_State."Facility Off") -> (x = y?=w2247:bool)
                n699 = Compound Arithmetic op=OR(w2296, w2294, w2247) -> (w2293:bool)
                n700 = case shown="False" w2293 {
                  tunnel: w2298 -> [w2367 _]
                  tunnel: w2297 -> [w2366 w2370]
                  tunnel: [w2367 w2368] -> w2292
                  tunnel: [w2366 w2369] -> w2291
                  tunnel: w2237 -> [w2365 _]
                  tunnel: [w2365 w2368] -> w2236
                  frame False {
                  }
                  frame True {
                    w2368 = FALSE
                    n701 = Bundle By Name(cluster=w2370, "Turbo Motor SYS CMD"=w2368) -> (w2369:T3)
                  }
                }
                n702 = Equal?(x=Current_Facility_State."Pumping to High Vac" ("y"), y=w2246) -> (x = y?=w2335:bool)
                n703 = Or(x=w2335, y=w2249) -> (x .or. y?=w2233:bool)
                n704 = And(x=w2281, y=w2335) -> (x .and. y?=w2346:bool)
                n705 = Select(t=Current_Facility_State."Engage Turbo" ("x"), s=w2346, f=w2345) -> (s? t:f=w2339:T1)
                n706 = local read "New_State?"() -> (w2276:bool)
                n707 = Select(t=FALSE, s=w2276, f="Overnight Pump 3") -> (s? t:f=w2259:bool)
                n708 = Select(t=Current_Facility_State."Overnight Pump", s=w2259, f=w2246) -> (s? t:f=w2303:T1)
                n709 = local read "New_State?"() -> (w2274:bool)
                n710 = Select(t=FALSE, s=w2274, f="Pump to Rough 2") -> (s? t:f=w2258:bool)
                n711 = Select(t=Current_Facility_State."Pumping to Rough", s=w2258, f=w2303) -> (s? t:f=w2302:T1)
                n712 = local read "New_State?"() -> (w2270:bool)
                n713 = case shown="False" FALSE {
                  tunnel: w2292 -> [w2355 _]
                  tunnel: w2291 -> [w2354 w2364]
                  tunnel: [w2355 w2357] -> w2289
                  tunnel: [w2354 w2363] -> w2290
                  tunnel: w2236 -> [w2353 _]
                  tunnel: [w2353 w2356] -> w2235
                  frame False {
                  }
                  frame True {
                    n714 = local read "Which_Turbos_used?"() -> (w2362:bool[])
                    n715 = Index Array(array=w2362, index=0) -> (element=w2358:bool)
                    n716 = Index Array(array=w2362, index=1) -> (element=w2356:bool)
                    n717 = Index Array(array=w2362, index=2) -> (element=w2357:bool)
                    n718 = Bundle By Name(cluster=w2364, "Turbo Motor SYS CMD"=w2358) -> (w2363:T3)
                  }
                }
                n719 = Select(t=FALSE, s=w2270, f="Pump to High Vac 2") -> (s? t:f=w2257:bool)
                n720 = Select(t=Current_Facility_State."Pumping to High Vac", s=w2257, f=w2302) -> (s? t:f=w2279:T1)
                n721 = Less?(x=w2286, y=w2285) -> (x < y?=w2284:bool)
                n722 = Equal?(x=w2246, y=Current_Facility_State."Pumping to High Vac") -> (x = y?=w2287:bool)
                n723 = local read "New_State?"() -> (w2268:bool)
                n724 = local read "New_State?"() -> (w2264:bool)
                n725 = And(x=w2287, y=w2284) -> ()  [unwired: 1 out]
                n726 = Select(t=FALSE, s=w2268, f="Shut Off once rough") -> (s? t:f=w2253:bool)
                n727 = Select(t=w2254, s=w2253, f=w2279) -> (s? t:f=w2278:T1)
                n728 = Select(t=FALSE, s=w2264, f="Shut Off") -> (s? t:f=w2252:bool)
                n729 = Select(t=w2254, s=w2252, f=w2278) -> (s? t:f=w2255:T1)
                n730 = Equal?(x=w2255, y=w2254) -> (x = y?=w2282:bool)
                n731 = for {
                  tunnel: w2309 -> [w2405]
                  tunnel: w2286 -> [w2404]
                  tunnel: w2299 -> [w2403] mode=indexing
                  tunnel: w2328 -> [w2401] mode=indexing
                  tunnel: [w2400] -> w2327 mode=indexing
                  tunnel: w2281 -> [w2399]
                  n732 = Less?(x=w2404, y=w2403) -> (x < y?=w2406:bool)
                  n733 = And(x=w2406, y=w2405) -> (x .and. y?=w2402:bool)
                  n734 = Compound Arithmetic op=OR(w2402, w2401, w2399) -> (w2400:bool)
                }
                n735 = And(x=w2282, y=w2281) -> (x .and. y?=w2280:bool)
                n736 = Or(x=w2252, y=w2280) -> (x .or. y?=w2283:bool)
                n737 = Select(t=Current_Facility_State."Turbo slowing", s=w2232, f=Current_Facility_State."Facility Off" ("t")) -> (s? t:f=w2248:T1)
                n738 = Select(t=w2248, s=w2283, f=w2339) -> (s? t:f=w2350:T1)
                n739 = local read "New_State?"() -> (w2262:bool)
                n740 = Select(t=FALSE, s=w2262, f="Vent 2") -> (s? t:f=w2256:bool)
                n741 = Compound Arithmetic op=OR(w2256, w2283, w2259) -> (w2305:bool)
                n742 = Select(t=Current_Facility_State."Venting", s=w2256, f=w2255) -> (s? t:f=w2334:T1)
                n743 = Select(t=FALSE, s=w2305, f=w2316) -> (s? t:f=w2322:bool)
                n744 = local read "Which_Turbos_used?"() -> (w2320:bool[])
                n745 = And(x=w2327, y=w2320) -> (x .and. y?=w2321:bool[])
                n746 = Select(t=Current_Facility_State."Venting", s=w2256, f=w2350) -> (s? t:f=w2332:T1)
                n747 = Not Equal?(x=w2332, y=Current_Facility_State."Pumping to Rough") -> (x != y?=w2336:bool)
                n748 = case shown="False" w2336 {
                  tunnel: w2313 -> [w2407 _]
                  tunnel: [w2407 0 ("t")] -> w2331
                  frame False {
                  }
                  frame True {
                  }
                }
                n749 = Not Equal?(x=w2255, y=Current_Facility_State."Pumping to Rough") -> (x != y?=w2325:bool)
                n750 = And(x=w2321, y=w2325) -> (x .and. y?=w2307:bool[])
                n751 = Select(t=bool[] [FALSE, FALSE, FALSE] ("appended array"), s=w2305, f=w2307) -> (s? t:f=w2306:bool[])
              }
              frame "Overnight Pump" {
                (unwired) FALSE ("Turbo_Error_Acknowlege_Cmd")
                w2456 = Current_Facility_State."Pumping to Rough" ("t")
                w2410 = FALSE ("Turbo_Error_Acknowlege_Cmd")
                w2460 = Current_Facility_State."Venting" ("t")
                # "Turbo spinning?"
                n752 = local read "Turbo Engage time"() -> (w2430:timestamp)
                n753 = local read "Turbo slowing Threshold (%)"() -> (w2409:dbl)
                n754 = Index Array(array=w2413, index=1) -> (element=w2415:dbl)
                n755 = Index Array(array=w2413, index=0) -> (element=w2414:dbl)
                n756 = Unbundle By Name(w2442) -> ("Turbo Rotating Read"=w2441:bool)
                n757 = Greater?(x=w2415, y=w2409) -> (0:w2412:bool)
                n758 = Greater?(x=w2414, y=w2409) -> (0:w2411:bool)
                n759 = Get Date/Time In Seconds() -> (seconds since 1Jan1904=w2431:timestamp)
                n760 = Build Array(w2441, w2411, w2412) -> (w2440:bool[])
                n761 = Compound Arithmetic op=OR(w2441, w2411, w2412) -> (w2438:bool)
                n762 = Greater?(x=w2431, y=w2430) -> (0:w2444:bool)
                n763 = Select(t=Current_Facility_State."Pumping to High Vac", s=w2444, f=w2453) -> (s? t:f=w2452:T1)
                n764 = case shown="True" w2444 {
                  tunnel: w2448 -> [w2466 w2471]
                  tunnel: [w2466 w2470] -> w2447
                  frame False {
                  }
                  frame True {
                    n765 = Get Date/Time String(want seconds? (F)=TRUE) -> (time string=w2467:string)  [unwired: 2 in, 1 out]
                    n766 = Concatenate Strings(w2471, "\r", "Timestamp reached, turning on pumps at " ("string"), w2467) -> (w2470:string)
                  }
                }
                n767 = Select(t=Current_Facility_State."Pumping to Rough", s=w2444, f=Current_Facility_State."Overnight Pump") -> (s? t:f=w2450:T1)
                n768 = local read "New_State?"() -> (w2429:bool)
                n769 = Select(t=FALSE, s=w2429, f="Vent 4") -> (s? t:f=w2427:bool)
                n770 = Select(t=w2460, s=w2427, f=w2450) -> (s? t:f=w2463:T1)
                n771 = Select(t=w2460, s=w2427, f=w2452) -> (s? t:f=w2459:T1)
                n772 = local read "New_State?"() -> (w2425:bool)
                n773 = Select(t=FALSE, s=w2425, f="Pump to Rough 3") -> (s? t:f=w2422:bool)
                n774 = Select(t=w2456, s=w2422, f=w2463) -> (s? t:f=w2462:T1)
                n775 = Select(t=w2456, s=w2422, f=w2459) -> (s? t:f=w2458:T1)
                n776 = local read "New_State?"() -> (w2421:bool)
                n777 = Select(t=FALSE, s=w2421, f="Pump to High Vac 3") -> (s? t:f=w2418:bool)
                n778 = Select(t=Current_Facility_State."Pumping to High Vac", s=w2418, f=w2458) -> (s? t:f=w2457:T1)
                n779 = Select(t=Current_Facility_State."Pumping to Rough", s=w2418, f=w2462) -> (s? t:f=w2434:T1)
                n780 = local read "Which_Turbos_used?"() -> (w2439:bool[])
                n781 = And(x=w2439, y=w2440) -> (x .and. y?=w2437:bool[])
                n782 = Not Equal?(x=w2434, y=Current_Facility_State."Overnight Pump") -> (x != y?=w2432:bool)
                n783 = Select(t=bool[] [FALSE, FALSE, FALSE] ("appended array"), s=w2432, f=w2437) -> (s? t:f=w2436:bool[])
              }
              frame "Engage Turbo" {
                (unwired) FALSE ("Turbo_Error_Acknowlege_Cmd")
                # "Command Turbo"
                n784 = case shown="1" w2498 {
                  tunnel: [TRUE ("Valve_Bypass_User_Cmd") TRUE ("Valve_Bypass_User_Cmd") TRUE ("Valve_Bypass_User_Cmd") FALSE ("Valve_Bypass_User_Cmd") FALSE ("Valve_Bypass_User_Cmd") FALSE ("Valve_Bypass_User_Cmd")] -> w2497
                  tunnel: [w2502 w2525 w2557 w2566 w2575 w2583] -> w2495
                  tunnel: [Current_Facility_State."Engage Turbo" ("f") w2534 Current_Facility_State."Engage Turbo" ("f") Current_Facility_State."Engage Turbo" ("f") Current_Facility_State."Engage Turbo" ("f") Current_Facility_State."Pumping to High Vac" ("f")] -> w2494
                  tunnel: w2493 -> [_ w2539 _ _ _ _]
                  tunnel: w2492 -> [_ _ _ _ _ _]
                  tunnel: w2491 -> [_ w2538 _ _ _ _]
                  tunnel: [1 ("Sub_state_iteration") w2532 3 ("Sub_state_iteration") 4 ("f") 5 ("f") 0 ("f")] -> w2490
                  tunnel: w2489 -> [w2503 w2529 w2559 w2569 w2578 w2593]
                  tunnel: [w2503 w2528 w2559 w2569 w2578 w2593] -> w2488
                  tunnel: [Current_Facility_State."Pumping to High Vac" ("f") Current_Facility_State."Pumping to High Vac" ("Target Facility State") Current_Facility_State."Pumping to High Vac" ("f") Current_Facility_State."Pumping to High Vac" ("f") Current_Facility_State."Pumping to High Vac" ("f") Current_Facility_State."Pumping to High Vac" ("f")] -> w2487
                  tunnel: w2486 -> [_ w2511 _ _ _ _]
                  tunnel: w2485 -> [w2502 w2525 w2557 w2566 w2575 _]
                  tunnel: [bool[] [FALSE, FALSE, FALSE] ("appended array") bool[] [FALSE, FALSE, FALSE] ("appended array") bool[] [FALSE, FALSE, FALSE] ("appended array") bool[] [FALSE, FALSE, FALSE] ("appended array") bool[] [TRUE, TRUE, TRUE] ("appended array") bool[] [TRUE, TRUE, TRUE] ("appended array")] -> w2480
                  tunnel: w2478 -> [w2500 w2520 w2556 w2565 w2574 w2590]
                  tunnel: [w2500 w2520 w2556 w2565 w2574 w2588] -> w2477
                  tunnel: [w2499 w2508 w2554 w2563 w2572 w2581] -> w2476
                  tunnel: w2475 -> [w2499 w2508 w2554 w2563 w2572 _]
                  frame 0, Default {
                    (unwired) FALSE ("T button?")
                    # "Init"
                  }
                  frame 1 {
                    w2512 = 15.0 ("y")
                    w2523 = 5.0  # Threshold_wiggle_room_multiplier
                    # "Any Turbos spinnig?"
                    # "Foreline Pressuse"
                    # "WRG Pressuse"
                    # "Check safe to turn on turbo/open gate"
                    n785 = Unbundle By Name(w2520) -> ("Turbo Rotating Read"=w2521:bool)
                    n786 = local read "Turbo on Threshold (torr)"() -> (w2517:dbl)
                    n787 = Index Array(array=w2511, index=1) -> (element=w2514:dbl)
                    n788 = Index Array(array=w2511, index=0) -> (element=w2513:dbl)
                    n789 = Greater?(x=w2514, y=w2512) -> (0:w2509:bool)
                    n790 = Greater?(x=w2513, y=w2512) -> (0:w2510:bool)
                    n791 = Compound Arithmetic op=OR(w2521, w2510, w2509) -> (w2519:bool)
                    n792 = Multiply(x=w2517, y=w2523) -> (x*y=w2524:dbl)
                    n793 = Less?(x=w2539, y=w2524) -> (x < y?=w2537:bool)
                    n794 = Less?(x=w2538, y=w2524) -> (x < y?=w2536:bool)
                    n795 = And(x=w2537, y=w2536) -> (x .and. y?=w2526:bool)
                    n796 = Select(t=Current_Facility_State."Engage Turbo" ("f"), s=w2526, f=Current_Facility_State."Pumping to Rough") -> (s? t:f=w2534:T1)
                    n797 = Select(t=2, s=w2526, f=0 ("Sub_state_iteration")) -> (s? t:f=w2532:i32)
                    n798 = case shown="False" w2526 {
                      tunnel: w2529 -> [w2544 w2551]
                      tunnel: [w2545 w2552] -> w2528
                      tunnel: w2519 -> [w2540 w2547]
                      frame False {
                        n799 = Select(t="Pressure NOT low enough to open gates!" ("string"), s=w2540, f="Pressure NOT low enough to turn on turbos!" ("string")) -> (s? t:f=w2542:string)
                        n800 = Concatenate Strings(w2544, "\r", w2542) -> (w2545:string)
                      }
                      frame True {
                        n801 = Select(t="Pressure low enough to open gates" ("string"), s=w2547, f="Pressure low enough to turn on turbos" ("string")) -> (s? t:f=w2548:string)
                        n802 = Concatenate Strings(w2551, "\r", w2548) -> (w2552:string)
                      }
                    }
                  }
                  frame 2 {
                    (unwired) FALSE ("T button?")
                    # "Open turbo Valve"
                  }
                  frame 3 {
                    (unwired) FALSE ("T button?")
                    # "Close Bypass"
                  }
                  frame 4 {
                    (unwired) TRUE ("T button?")
                    # "Open Gate"
                  }
                  frame 5 {
                    # "Turn on Turbo"
                    n803 = local read "Which_Turbos_used?"() -> (w2584:bool[])
                    n804 = Index Array(array=w2584, index=1) -> (element=w2581:bool)
                    n805 = Index Array(array=w2584, index=0) -> (element=w2582:bool)
                    n806 = Index Array(array=w2584, index=2) -> (element=w2583:bool)
                    n807 = Bundle By Name(cluster=w2590, "Turbo Motor SYS CMD"=w2582) -> (w2588:T3)
                  }
                }
                n808 = local read "Which_Turbos_used?"() -> (w2481:bool[])
                n809 = And(x=w2481, y=w2480) -> (x .and. y?=w2479:bool[])
                n810 = And(x=w2481, y=bool[] [TRUE, TRUE, TRUE] ("appended array")) -> (x .and. y?=w2482:bool[])
              }
              frame "Pumping to High Vac" {
                (unwired) TRUE ("T button?")
                # "Keep Primary on?"
                # "Turn off Turbo?"
                n811 = local read "New_State?"() -> (w2618:bool)
                n812 = Select(t=FALSE, s=w2618, f="Shutdown") -> (s? t:f=w2615:bool)
                n813 = Select(t=Current_Facility_State."Disengage Turbo", s=w2615, f=Current_Facility_State."Pumping to High Vac") -> (s? t:f=w2659:T1)
                n814 = Select(t=Current_Facility_State."Facility Off", s=w2615, f=w2655) -> (s? t:f=w2654:T1)
                n815 = local read "New_State?"() -> (w2614:bool)
                n816 = Select(t=FALSE, s=w2614, f="Pump to Rough 4") -> (s? t:f=w2611:bool)
                n817 = Select(t=Current_Facility_State."Pumping to Rough", s=w2611, f=w2654) -> (s? t:f=w2653:T1)
                n818 = Select(t=Current_Facility_State."Disengage Turbo", s=w2611, f=w2659) -> (s? t:f=w2658:T1)
                n819 = local read "New_State?"() -> (w2610:bool)
                n820 = Select(t=FALSE, s=w2610, f="Overnight Pump 2") -> (s? t:f=w2607:bool)
                n821 = Select(t=Current_Facility_State."Overnight Pump" ("f"), s=w2607, f=w2653) -> (s? t:f=w2652:T1)
                n822 = Select(t=Current_Facility_State."Disengage Turbo", s=w2607, f=w2658) -> (s? t:f=w2657:T1)
                n823 = local read "New_State?"() -> (w2606:bool)
                n824 = Select(t=FALSE, s=w2606, f="Vent and shutdonw") -> (s? t:f=w2603:bool)
                n825 = Select(t=Current_Facility_State."Vent and Shutdown", s=w2603, f=w2652) -> (s? t:f=w2642:T1)
                n826 = Select(t=Current_Facility_State."Disengage Turbo", s=w2603, f=w2657) -> (s? t:f=w2640:T1)
                n827 = local read "Which_Turbos_used?"() -> (w2621:bool[])
                n828 = local read "New_State?"() -> (w2602:bool)
                n829 = Compound Arithmetic op=OR(w2615, w2611, w2607, w2603) -> (w2644:bool)
                n830 = Select(t=FALSE, s=w2602, f="Vent 5") -> (s? t:f=w2599:bool)
                n831 = Not(x=w2644) -> (.not. x?=w2627:bool)
                n832 = Index Array(array=w2621, index=0) -> (element=w2620:bool)
                n833 = Index Array(array=w2621, index=1) -> (element=w2619:bool)
                n834 = Index Array(array=w2621, index=2) -> (element=w2625:bool)
                n835 = And(x=w2620, y=w2627) -> (x .and. y?=w2628:bool)
                n836 = Select(t=Current_Facility_State."Disengage Turbo", s=w2599, f=w2640) -> (s? t:f=w2639:T1)
                n837 = Select(t=Current_Facility_State."Venting", s=w2599, f=w2642) -> (s? t:f=w2641:T1)
                n838 = And(x=w2627, y=w2625) -> (x .and. y?=w2626:bool)
                n839 = And(x=w2619, y=w2627) -> (x .and. y?=w2598:bool)
                n840 = Bundle By Name(cluster=w2630, "Turbo Motor SYS CMD"=w2628) -> (w2629:T3)
                n841 = local read "Which_Turbos_used?"() -> (w2635:bool[])
                n842 = local read "Which_Turbos_used?"() -> (w2633:bool[])
                n843 = And(x=w2635, y=bool[] [TRUE, TRUE, TRUE] ("appended array")) -> (x .and. y?=w2634:bool[])
                n844 = And(x=w2633, y=bool[] [TRUE, TRUE, TRUE] ("appended array")) -> (x .and. y?=w2631:bool[])
              }
              frame "Disengage Turbo" {
                n845 = case shown="1" w2681 {
                  tunnel: w2683 -> [w2693 w2710 w2741]
                  tunnel: [w2693 w2710 w2741] -> w2673
                  tunnel: [1 ("f") w2704 0 ("f")] -> w2680
                  tunnel: [w2687 w2698 w2715] -> w2672
                  tunnel: [Current_Facility_State."Disengage Turbo" ("f") Current_Facility_State."Disengage Turbo" ("f") w2720] -> w2678
                  tunnel: w2677 -> [w2691 w2702 w2724]
                  tunnel: [w2691 w2702 w2724] -> w2676
                  tunnel: [FALSE FALSE w2730] -> w2675
                  tunnel: [bool[] [FALSE, FALSE, FALSE] ("appended array") bool[] [FALSE, FALSE, FALSE] ("appended array") bool[] [FALSE, FALSE, FALSE] ("appended array")] -> w2671
                  tunnel: [w2685 w2696 w2712] -> w2669
                  tunnel: w2670 -> [w2685 w2696 w2712]
                  tunnel: w2668 -> [w2684 w2695 w2711]
                  tunnel: [w2684 w2695 w2711] -> w2667
                  frame 0, Default {
                    # "Close gate"
                    n846 = local read "Which_Turbos_used?"() -> (w2689:bool[])
                    n847 = And(x=w2689, y=bool[] [TRUE, TRUE, TRUE] ("appended array")) -> (x .and. y?=w2687:bool[])
                  }
                  frame 1 {
                    (unwired) FALSE ("T button?")
                    # "Wait 3 secs"
                    n848 = call "Elapsed Time2"("Time Target (s)"=1.0, "Auto Reset"=TRUE) -> ("Time has Elapsed"=w2706:bool)  [unwired: 10 in, 7 out]
                    n849 = Select(t=2 ("Sub_state_iteration"), s=w2706, f=1) -> (s? t:f=w2704:i32)
                    n850 = local read "Which_Turbos_used?"() -> (w2700:bool[])
                    n851 = And(x=w2700, y=bool[] [TRUE, TRUE, TRUE] ("appended array")) -> (x .and. y?=w2698:bool[])
                  }
                  frame 2 {
                    (unwired) FALSE ("T button?")
                    # "Overnight pump"
                    # "Slowing down"
                    # "Close Turbo Valve"
                    n852 = Equal?(x=w2724, y=Current_Facility_State."Pumping to Rough" ("t")) -> (x = y?=w2730:bool)
                    n853 = Select(t=Current_Facility_State."Pumping to Rough", s=w2730, f=Current_Facility_State."Turbo slowing" ("y")) -> (s? t:f=w2726:T1)
                    n854 = Equal?(x=w2724, y=Current_Facility_State."Overnight Pump") -> (x = y?=w2728:bool)
                    n855 = Select(t=Current_Facility_State."Overnight Pump", s=w2728, f=w2726) -> (s? t:f=w2725:T1)
                    n856 = Equal?(x=w2724, y=Current_Facility_State."Vent and Shutdown") -> (x = y?=w2735:bool)
                    n857 = Equal?(x=w2724, y=Current_Facility_State."Venting") -> (x = y?=w2719:bool)
                    n858 = Or(x=w2735, y=w2719) -> (x .or. y?=w2734:bool)
                    n859 = Select(t=Current_Facility_State."Venting", s=w2734, f=w2725) -> (s? t:f=w2722:T1)
                    n860 = Equal?(x=w2724, y=Current_Facility_State."Facility Off") -> (x = y?=w2721:bool)
                    n861 = Select(t=Current_Facility_State."Turbo slowing", s=w2721, f=w2722) -> (s? t:f=w2720:T1)
                    n862 = Select(t=bool[] [TRUE, TRUE, TRUE] ("appended array"), s=w2719, f=bool[] [FALSE, FALSE, FALSE] ("appended array")) -> (s? t:f=w2718:bool[])
                    n863 = local read "Which_Turbos_used?"() -> (w2714:bool[])
                    n864 = And(x=w2714, y=w2718) -> (x .and. y?=w2715:bool[])
                  }
                }
              }
              frame "Venting" {
                (unwired) FALSE ("T button?")
                # "Stop Turbos?"
                # "Close Vent ?"
                # "Close Turbo Vavle when \nventing is complete, \nor changing state,\nor if it is the first iteration"
                # "For 20 mins"
                # "Open Vent valve"
                n865 = local read "Turbo slowing Threshold (%)"() -> (w2742:dbl)
                n866 = Unbundle By Name(w2794) -> ("Turbo Rotating Read"=w2798:bool)
                n867 = Index Array(array=w2748, index=1) -> (element=w2750:dbl)
                n868 = Index Array(array=w2748, index=0) -> (element=w2749:dbl)
                n869 = Greater?(x=w2750, y=w2742) -> (0:w2747:bool)
                n870 = Greater?(x=w2749, y=w2742) -> (0:w2744:bool)
                n871 = Compound Arithmetic op=OR(w2798, w2744, w2747) -> (w2743:bool)
                n872 = Build Array(w2798, w2744, w2747) -> (w2771:bool[])
                n873 = Select(t=Current_Facility_State."Turbo slowing" ("y"), s=w2743, f=Current_Facility_State."Facility Off") -> (s? t:f=w2832:T1)
                n874 = Equal?(x=w2835, y=Current_Facility_State."Facility Off" ("t")) -> (x = y?=w2837:bool)
                n875 = Equal?(x=w2835, y=Current_Facility_State."Vent and Shutdown") -> (x = y?=w2758:bool)
                n876 = Or(x=w2758, y=w2837) -> (x .or. y?=w2836:bool)
                n877 = Select(t=w2832, s=w2836, f=Current_Facility_State."Venting") -> (s? t:f=w2842:T1)
                n878 = Equal?(x=w2775, y=0) -> (x = y?=w2816:bool)
                n879 = Select(t=Current_Facility_State."Facility Off", s=w2836, f=w2835) -> (s? t:f=w2811:T1)
                n880 = Multiply(x=15.0, y=60.0) -> (x*y=w2823:dbl)
                n881 = call "Elapsed Time4"("Time Target (s)"=w2823, "Reset"=w2816, "Auto Reset"=TRUE) -> ("Elapsed Time (s)"=→"Vent Time (s) 2":dbl, "Time has Elapsed"=w2818:bool)  [unwired: 9 in, 6 out]
                n882 = case shown="2" w2775 {
                  tunnel: [TRUE TRUE FALSE] -> w2759
                  tunnel: [1 ("Sub_state_iteration") w2866 2 ("Sub_state_iteration")] -> w2828
                  tunnel: w2818 -> [_ w2864 _]
                  frame 0, Default {
                  }
                  frame 1 {
                    n883 = Select(t=2, s=w2864, f=1 ("Sub_state_iteration")) -> (s? t:f=w2866:i32)
                  }
                  frame 2 {
                  }
                }
                n884 = Select(t=Current_Facility_State."Venting" ("f"), s=w2759, f=w2842) -> (s? t:f=w2814:T1)
                n885 = local read "New_State?"() -> (w2789:bool)
                n886 = Select(t=FALSE, s=w2789, f="Overnight Pump 5") -> (s? t:f=w2755:bool)
                n887 = local read "New_State? 2"() -> (w2762:bool)
                n888 = local read "New_State?"() -> (w2780:bool)
                n889 = Select(t=FALSE, s=w2762, f="Shutdown After Vent") -> (s? t:f=w2760:bool)
                n890 = Select(t=Current_Facility_State."Pumping to Rough", s=w2755, f=w2814) -> (s? t:f=w2813:T1)
                n891 = Select(t=FALSE, s=w2780, f="Shutdown Now") -> (s? t:f=w2754:bool)
                n892 = Select(t=Current_Facility_State."Overnight Pump", s=w2755, f=w2811) -> (s? t:f=w2802:T1)
                n893 = Or(x=w2760, y=w2754) -> (x .or. y?=w2761:bool)
                n894 = Select(t=Current_Facility_State."Facility Off", s=w2761, f=w2802) -> (s? t:f=w2769:T1)
                n895 = Select(t=Current_Facility_State."Turbo slowing", s=w2743, f=Current_Facility_State."Facility Off") -> (s? t:f=w2807:T1)
                n896 = Select(t=w2807, s=w2754, f=w2813) -> (s? t:f=w2804:T1)
                n897 = local read "New_State?"() -> (w2786:bool)
                n898 = for {
                  tunnel: w2772 -> [w2853]
                  tunnel: w2773 -> [w2852] mode=indexing
                  tunnel: [w2847] -> w2770 mode=indexing
                  tunnel: w2771 -> [w2851] mode=indexing
                  tunnel: w2767 -> [w2850] mode=indexing
                  n899 = Less?(x=w2853, y=w2852) -> (x < y?=w2849:bool)
                  n900 = Or(x=w2849, y=w2850) -> (x .or. y?=w2848:bool)
                  n901 = And(x=w2851, y=w2848) -> (x .and. y?=w2847:bool)
                }
                n902 = Select(t=FALSE, s=w2786, f="Pump to Rough 5") -> (s? t:f=w2756:bool)
                n903 = Compound Arithmetic op=OR(w2755, w2754, w2756, w2760) -> (w2790:bool)
                n904 = case shown="False" w2790 {
                  tunnel: w2794 -> [w2855 w2860]
                  tunnel: w2793 -> [w2856 _]
                  tunnel: [w2856 w2857] -> w2792
                  tunnel: [w2855 w2859] -> w2791
                  tunnel: [w2854 w2857] -> w2746
                  tunnel: w2745 -> [w2854 _]
                  frame False {
                  }
                  frame True {
                    w2857 = FALSE
                    n905 = Bundle By Name(cluster=w2860, "Turbo Motor SYS CMD"=FALSE) -> (w2859:T3)
                  }
                }
                n906 = Select(t=Current_Facility_State."Pumping to Rough", s=w2756, f=w2804) -> (s? t:f=w2803:T1)
                n907 = Select(t=Current_Facility_State."Pumping to Rough", s=w2756, f=w2769) -> (s? t:f=w2801:T1)
                n908 = Equal?(x=w2775, y=0) -> (x = y?=w2776:bool)
                n909 = local read "New_State?"() -> (w2783:bool)
                n910 = local read "Which_Turbos_used?"() -> (w2799:bool[])
                n911 = Select(t=FALSE, s=w2783, f="Pump to Hi vac") -> (s? t:f=w2757:bool)
                n912 = Compound Arithmetic op=OR(w2757, w2756, w2755, w2754) -> (w2753:bool)
                n913 = Select(t=FALSE, s=w2753, f=w2759) -> (s? t:f=w2766:bool)
                n914 = Select(t=Current_Facility_State."Pumping to Rough", s=w2757, f=w2803) -> (s? t:f=w2825:T1)
                n915 = Select(t=Current_Facility_State."Pumping to High Vac", s=w2757, f=w2801) -> (s? t:f=w2830:T1)
                n916 = Not Equal?(x=w2825, y=Current_Facility_State."Venting") -> (x != y?=w2815:bool)
                n917 = Or(x=w2815, y=w2776) -> (x .or. y?=w2777:bool)
                n918 = Select(t=0, s=w2815, f=w2828) -> (s? t:f=w2827:i32)
                n919 = And(x=w2799, y=w2770) -> (x .and. y?=w2797:bool[])
                n920 = Select(t=bool[] [FALSE, FALSE, FALSE] ("appended array"), s=w2777, f=w2797) -> (s? t:f=w2796:bool[])
              }
              frame "Turbo slowing" {
                (unwired) FALSE ("Turbo_Error_Acknowlege_Cmd")
                n921 = Index Array(array=w2876, index=1) -> (element=w2879:dbl)
                n922 = Unbundle By Name(w2922) -> ("Turbo Rotating Read"=w2923:bool)
                n923 = Index Array(array=w2876, index=0) -> (element=w2878:dbl)
                n924 = Greater?(x=w2879, y="Turbo slowing Threshold (%)") -> (0:w2875:bool)
                n925 = Greater?(x=w2878, y="Turbo slowing Threshold (%)") -> (0:w2874:bool)
                n926 = Compound Arithmetic op=OR(w2923, w2874, w2875) -> (w2870:bool)
                n927 = Build Array(w2923, w2874, w2875) -> (w2902:bool[])
                n928 = Select(t=Current_Facility_State."Turbo slowing" ("f"), s=w2870, f=Current_Facility_State."Facility Off") -> (s? t:f=w2886:T1)
                n929 = local read "New_State?"() -> (w2889:bool)
                n930 = Select(t=FALSE, s=w2889, f="Vent") -> (s? t:f=w2884:bool)
                n931 = Select(t=Current_Facility_State."Venting", s=w2884, f=w2886) -> (s? t:f=w2885:T1)
                n932 = local read "New_State?"() -> (w2909:bool)
                n933 = for {
                  tunnel: w2899 -> [w2934]
                  tunnel: w2900 -> [w2933] mode=indexing
                  tunnel: [w2928] -> w2901 mode=indexing
                  tunnel: w2902 -> [w2929] mode=indexing
                  tunnel: w2898 -> [w2932] mode=indexing
                  n934 = Less?(x=w2934, y=w2933) -> (x < y?=w2930:bool)
                  n935 = Or(x=w2930, y=w2932) -> (x .or. y?=w2931:bool)
                  n936 = And(x=w2931, y=w2929) -> (x .and. y?=w2928:bool)
                }
                n937 = Select(t=FALSE, s=w2909, f="Pump to High Vac 4") -> (s? t:f=w2906:bool)
                n938 = local read "Which_Turbos_used?"() -> (w2920:bool[])
                n939 = Select(t=TRUE ("Turbo_Error_Acknowlege_Cmd"), s=w2906, f=FALSE) -> (s? t:f=w2873:bool)
                n940 = Bundle By Name(cluster=w2922, "Turbo Motor SYS CMD"=w2873) -> (w2921:T3)
                n941 = Select(t=Current_Facility_State."Pumping to Rough", s=w2906, f=w2885) -> (s? t:f=w2904:T1)
                n942 = Select(t=Current_Facility_State."Pumping to High Vac", s=w2906, f=Current_Facility_State."Facility Off" ("Target Facility State")) -> (s? t:f=w2916:T1)
                n943 = Equal?(x=w2882, y=0 ("Sub_state_iteration")) -> (x = y?=w2895:bool)
                n944 = And(x=w2920, y=w2901) -> (x .and. y?=w2914:bool[])
                n945 = Not Equal?(x=w2904, y=Current_Facility_State."Turbo slowing") -> (x != y?=w2894:bool)
                n946 = Or(x=w2894, y=w2895) -> (x .or. y?=w2897:bool)
                n947 = Select(t=bool[] [FALSE, FALSE, FALSE], s=w2897, f=w2914) -> (s? t:f=w2913:bool[])
                n948 = Select(t=0 ("Sub_state_iteration"), s=w2894, f=1) -> (s? t:f=w2892:i32)
              }
            }
            n949 = Index Array(array=w2032, index=0) -> (element=w2084:bool)
            n950 = Unbundle By Name(w2090) -> ("Turbo Motor SYS CMD"=w2082:bool)
            n951 = Index Array(array=w2032, index=1) -> (element=w2031:bool)
            n952 = Index Array(array=w2032, index=2) -> (element=w2030:bool)
            n953 = Not(x=w2084) -> (.not. x?=w2085:bool)
            n954 = Not(x=w2030) -> (.not. x?=w2028:bool)
            n955 = Not(x=w2031) -> (.not. x?=w2029:bool)
            n956 = case shown="True" w2017 {
              tunnel: [FALSE ("Turbo_Motor_User_Cmd") w2172] -> w2113
              tunnel: w2098 -> [w2170 w2174]
              tunnel: [w2170 w2173] -> w2087
              frame False {
              }
              frame True {
                n957 = local read "Turbo 3 Gauge"() -> (w2176:dbl)
                n958 = Less?(x=w2176, y=5.0) -> (x < y?=w2172:bool)
                n959 = case shown="False" w2172 {
                  tunnel: w2174 -> [w2181 w2182]
                  tunnel: [w2180 w2182] -> w2173
                  frame False {
                    n960 = Get Date/Time String(want seconds? (F)=TRUE) -> (time string=w2178:string)  [unwired: 2 in, 1 out]
                    n961 = Concatenate Strings(w2181, "High pressure turbo 3 shuttoff triggered at" ("string"), w2178) -> (w2180:string)
                  }
                  frame True {
                  }
                }
              }
            }
            n962 = case shown="True" w2082 {
              tunnel: [FALSE ("Turbo_Motor_User_Cmd") w2153] -> w2074
              tunnel: w2087 -> [w2150 w2154]
              tunnel: [w2150 w2152] -> w2086
              frame False {
              }
              frame True {
                n963 = local read "Turbo 1 Gauge"() -> (w2156:dbl)
                n964 = Less?(x=w2156, y=5.0) -> (x < y?=w2153:bool)
                n965 = case shown="False" w2153 {
                  tunnel: w2154 -> [w2161 w2162]
                  tunnel: [w2160 w2162] -> w2152
                  frame False {
                    n966 = Get Date/Time String(want seconds? (F)=TRUE) -> (time string=w2158:string)  [unwired: 2 in, 1 out]
                    n967 = Concatenate Strings(w2161, "High pressure turbo 1 shuttoff triggered at" ("string"), w2158) -> (w2160:string)
                  }
                  frame True {
                  }
                }
              }
            }
            n968 = case shown="True" w2026 {
              tunnel: [FALSE ("Turbo_Motor_User_Cmd") w2140] -> w2036
              tunnel: [w2137 w2141] -> w2088
              tunnel: w2086 -> [w2137 w2139]
              frame False {
              }
              frame True {
                n969 = local read "Turbo 2 Gauge"() -> (w2143:dbl)
                n970 = Less?(x=w2143, y=5.0) -> (x < y?=w2140:bool)
                n971 = case shown="True" w2140 {
                  tunnel: [w2148 w2149] -> w2141
                  tunnel: w2139 -> [w2144 w2149]
                  frame False {
                    n972 = Get Date/Time String(want seconds? (F)=TRUE) -> (time string=w2146:string)  [unwired: 2 in, 1 out]
                    n973 = Concatenate Strings(w2144, "High pressure turbo 1 shuttoff triggered at" ("string"), w2146) -> (w2148:string)
                  }
                  frame True {
                  }
                }
              }
            }
            n974 = And(x=w2085, y=w2082) -> (x .and. y?=w2076:bool)
            n975 = And(x=w2029, y=w2026) -> (x .and. y?=w2024:bool)
            n976 = And(x=w2028, y=w2017) -> (x .and. y?=w2018:bool)
            n977 = Get Date/Time In Seconds() -> (seconds since 1Jan1904=w2057:timestamp)
            n978 = local read "Which_Turbos_used?"() -> (w2073:bool[])
            n979 = Equal?(x=Current_Facility_State."Overnight Pump", y=w2052) -> (x = y?=w2051:bool)
            n980 = Subtract(x="Turbo Engage time", y=w2057) -> (x-y=w2061:dbl)
            n981 = Equal?(x=w2042, y=T2."Overnight Pump") -> (x = y?=w2053:bool)
            n982 = call "Is Value Changed.vim"("value"=w2045) -> ("changed or first call?"=w2044:bool)
            n983 = Or(x=w2053, y=w2051) -> (x .or. y?=w2049:bool)
            n984 = Divide(x=w2061, y=60.0) -> (x/y=w2062:dbl)
            n985 = local read "Which_Turbos_used?"() -> (w2070:bool[])
            n986 = property on="Countdown" class="Str"("Visible"=w2049) -> ()  [unwired: 2 in, 2 out]
            n987 = call "Elapsed Time6"("Time Target (s)"=3.0, "Reset"=w2044, "Auto Reset"=FALSE) -> ("Time has Elapsed"=w2041:bool)  [unwired: 9 in, 7 out]
            n988 = Divide(x=w2062, y=60.0) -> (x/y=w2059:dbl)
            n989 = And(x=w2032, y=w2073) -> (x .and. y?=w2072:bool[])
            n990 = Select(t=w2042, s=w2041, f=T2."Holding at Rough" ("Tab Control")) -> (s? t:f=→"Tab Control":T2)
            n991 = Quotient & Remainder(x=w2059, y=24.0) -> (x-y*floor(x/y)=w2065:dbl, floor(x/y)=w2068:dbl)
            n992 = Number To Decimal String(number=w2068) -> (decimal integer string=w2067:string)  [unwired: 1 in]
            n993 = Number To Decimal String(number=w2065) -> (decimal integer string=w2064:string)  [unwired: 1 in]
            n994 = And(x=w2122, y=w2070) -> (x .and. y?=w2071:bool[])
            n995 = Concatenate Strings(w2067, " days and " ("string"), w2064, " hours until turn on." ("string")) -> (→"Countdown":string)
            n996 = local read "Which_Turbos_used?"() -> (w2019:bool[])
            n997 = Index Array(array=w2019, index=0) -> (element=w2077:bool)
            n998 = Index Array(array=w2019, index=2) -> (element=w2021:bool)
            n999 = Index Array(array=w2019, index=1) -> (element=w2023:bool)
            n1000 = And(x=w2077, y=w2074) -> (x .and. y?=w2075:bool)
            n1001 = And(x=w2018, y=w2021) -> (x .and. y?=w2016:bool)
            n1002 = And(x=w2024, y=w2023) -> (x .and. y?=w2022:bool)
            n1003 = Bundle By Name(cluster=w2090, "Turbo Motor SYS CMD"=w2075, "Turbo Standby SYS CMD"=w2076) -> (w2089:T3)
            n1004 = Index Array(array=w2019, index=1) -> (element=w2037:bool)
            n1005 = Index Array(array=w2019, index=2) -> (element=w2079:bool)
            n1006 = And(x=w2113, y=w2079) -> (x .and. y?=w2081:bool)
            n1007 = And(x=w2037, y=w2036) -> (x .and. y?=w2035:bool)
          }
        }
        n1008 = Get Date/Time String(want seconds? (F)=TRUE) -> (date string=w1497:string, time string=w1498:string)  [unwired: 2 in]
        n1009 = Concatenate Strings(w1498, "       " ("string"), w1497) -> (→"Current Time/date":string)
        n1010 = Equal?(x=Facility_State."Auto", y=w1507) -> (x = y?=w1501:bool)
        n1011 = Select(t="Auto Control Mode", s=w1501, f="Admin Control Mode") -> (s? t:f=→"String 3":string)
        n1012 = Select(t=enum32{"Admin", "Debug", "Automatic"}."Automatic" ("Control Level"), s=w1501, f=enum32{"Admin", "Debug", "Automatic"}."Admin" ("Control Level")) -> (s? t:f=→"Control Level":enum32{"Admin", "Debug", "Automatic"})
        n1013 = property on="Valve_Turbo_1_User_Cmd" class="Bool"("Visible"=w1489) -> ()  [unwired: 2 in, 2 out]
        n1014 = property on="Valve_Turbo_2_User_Cmd" class="Bool"("Visible"=w1489) -> ()  [unwired: 2 in, 2 out]
        n1015 = property on="Valve_Gate_1_User_Cmd" class="Bool"("Visible"=w1489) -> ()  [unwired: 2 in, 2 out]
        n1016 = property on="Valve_Turbo_3_User_Cmd" class="Bool"("Visible"=w1489) -> ()  [unwired: 2 in, 2 out]
        n1017 = property on="Valve_Gate_3_User_Cmd" class="Bool"("Visible"=w1489) -> ()  [unwired: 2 in, 2 out]
        n1018 = property on="Chiller_User_Cmd" class="Bool"("Visible"=w1489) -> ()  [unwired: 2 in, 2 out]
        n1019 = property on="Turbo_1_Motor_User_Cmd" class="Bool"("Visible"=w1489) -> ()  [unwired: 2 in, 2 out]
        n1020 = property on="Valve_Gate_2_User_Cmd" class="Bool"("Visible"=w1489) -> ()  [unwired: 2 in, 2 out]
        n1021 = property on="Valve_Vent_User_Cmd" class="Bool"("Visible"=w1489) -> ()  [unwired: 2 in, 2 out]
        n1022 = property on="Primary_User_Cmd" class="Bool"("Visible"=w1489) -> ()  [unwired: 2 in, 2 out]
        n1023 = property on="Control Level" class="TabCtl (strict)"("Visible"=w1501) -> ()  [unwired: 2 in, 2 out]
        n1024 = property on="Change to Auto" class="Bool"("Visible"=w1489) -> ()  [unwired: 2 in, 2 out]
        "String 4" <- "Admin Control Mode Enabled" ("String 4")
      }
      frame #4 {
        w2935 = u32 2000  # Bypass Delay
        (unwired) bool[] [FALSE, FALSE, FALSE] ("appended array")
        w2983 = u32 9000  # Gate Delay
        w2985 = u32 1000  # Turbo Valve Delay
        # "Turbo Motor  Cmd"
        # "substate"
        # "Command Turbo"
        # "Command Chiller"
        # "Command Primary"
        # "Command"
        # "Command Valves"
        n1025 = feedback #1() -> (w2987:bool)  [unwired: 1 in]
        n1026 = Not Equal?(x=w2987, y=w2942) -> (x != y?=w2943:bool)
        n1027 = feedback-in #1(w2942) -> ()
        n1028 = local write "Valve_Bypass_Sys_Cmd"(w2959) -> ()
        n1029 = local write "Valve_Vent_Sys_Cmd"(w2958) -> ()
        n1030 = feedback #2() -> (w2976:bool)  [unwired: 1 in]
        n1031 = Not Equal?(x=w2976, y=w2941) -> (x != y?=w2975:bool)
        n1032 = And(x=w2975, y=w2941) -> (x .and. y?=w2944:bool)
        n1033 = feedback-in #2(w2941) -> ()
        n1034 = case shown="True" w2943 {
          frame False {
          }
          frame True {
            n1035 = Wait (ms)(milliseconds to wait=u32 10000) -> ()  [unwired: 1 out]
          }
        }
        n1036 = case shown="True" w2944 {
          frame False {
          }
          frame True {
            n1037 = Wait (ms)(milliseconds to wait=u32 10000) -> ()  [unwired: 1 out]
          }
        }
        n1038 = local write "Primary_Sys_Cmd"(w2941) -> ()
        n1039 = local write "Turbo_2_Motor_Sys_Cmd"(w2949) -> ()
        n1040 = local write "Turbo_3_Motor_Sys_Cmd"(w2946) -> ()
        n1041 = Index Array(array=w2967, index=0) -> (element=w2964:bool)
        "Valve_Gate_1_Sys_Cmd" <- w2964
        n1042 = Index Array(array=w2967, index=1) -> (element=w2963:bool)
        "Valve_Gate_2_Sys_Cmd" <- w2963
        n1043 = Index Array(array=w2967, index=2) -> (element=w2962:bool)
        "Valve_Gate_3_Sys_Cmd" <- w2962
        n1044 = Index Array(array=w2974, index=0) -> (element=w2970:bool)
        "Valve_Turbo_1_Sys_Cmd" <- w2970
        n1045 = Index Array(array=w2974, index=1) -> (element=w2969:bool)
        "Valve_Turbo_2_Sys_Cmd" <- w2969
        n1046 = Index Array(array=w2974, index=2) -> (element=w2968:bool)
        "Valve_Turbo_3_Sys_Cmd" <- w2968
        n1047 = Unbundle By Name(w2954) -> ("Turbo Motor SYS CMD"=w2953:bool, "Turbo Standby SYS CMD"=w2952:bool, "Turbo Reset  SYS CMD"=w2951:bool)
        n1048 = local write "Valve_Gate_2_Sys_Cmd"(w2963) -> ()
        n1049 = local write "Valve_Turbo_1_Sys_Cmd"(w2970) -> ()
        n1050 = local write "Valve_Gate_3_Sys_Cmd"(w2962) -> ()
        n1051 = local write "Valve_Gate_1_Sys_Cmd"(w2964) -> ()
        n1052 = local write "Valve_Turbo_2_Sys_Cmd"(w2969) -> ()
        n1053 = local write "Valve_Turbo_3_Sys_Cmd"(w2968) -> ()
        n1054 = Build Array(w2953, w2952, w2951, w2949, w2947, w2948, w2946, w2945) -> (w2955:bool[])
        n1055 = local write "Chiller_Sys_Cmd"(w2942) -> ()
        n1056 = Build Array (concatenate)(w2959, w2958, w2974, w2967) -> (w2957:bool[])
        n1057 = feedback #3() -> (w2984:bool[])  [unwired: 1 in]
        n1058 = Not Equal?(x=w2984, y=w2967) -> (x != y?=w2961:bool[])
        n1059 = feedback-in #3(w2967) -> ()
        n1060 = feedback-in #4(w2957) -> ()
        n1061 = feedback #4() -> (w2989:bool[])  [unwired: 1 in]
        n1062 = Not Equal?(x=w2957, y=w2989) -> (x != y?=w2938:bool[])
        n1063 = call-poly <vilib>:"DAQmx Write.vi"("task/channels in"=w3003, "data"=w2957) -> ("task out"=w3006:refnum<k21>, "error out"=w3005:errorcluster)  [unwired: 11 in, 1 out]
        n1064 = Or Array Elements(Boolean array=w2961) -> (logical OR=w2960:bool)
        n1065 = call-poly <vilib>:"DAQmx Write.vi"("task/channels in"=w2950, "data"=w2955) -> ("task out"=w2990:refnum<k21>, "error out"=w2994:errorcluster)  [unwired: 11 in, 1 out]
        n1066 = Index Array(array=w2938, index=0) -> (element=w2936:bool)
        n1067 = Or Array Elements(Boolean array=w2938) -> (logical OR=w2988:bool)
        n1068 = call-poly <vilib>:"DAQmx Write.vi"("task/channels in"=w3008, "data"=w2941) -> ("task out"=w3012:refnum<k21>, "error out"=w2998:errorcluster)  [unwired: 11 in, 1 out]
        n1069 = Select(t=w2983, s=w2960, f=w2985) -> (s? t:f=w2940:u32)
        n1070 = call-poly <vilib>:"DAQmx Write.vi"("task/channels in"=w3000, "data"=w2942) -> ("task out"=w2999:refnum<k21>, "error out"=w2995:errorcluster)  [unwired: 11 in, 1 out]
        n1071 = Select(t=w2935, s=w2936, f=w2940) -> (s? t:f=w2939:u32)
        n1072 = case shown="True" w2988 {
          tunnel: w2939 -> [_ w3015]
          frame False {
          }
          frame True {
            n1073 = Wait (ms)(milliseconds to wait=w3015) -> ()  [unwired: 1 out]
          }
        }
        n1074 = Merge Errors(w2994) -> (w2993:errorcluster)
        n1075 = Merge Errors(w2995, w2993) -> (w2996:errorcluster)
        n1076 = Merge Errors(w2998, w2996) -> (w2997:errorcluster)
        n1077 = Merge Errors(w3005, w2997) -> (w3004:errorcluster)
        n1078 = Merge Errors(w3011, w3004) -> (w3010:errorcluster)
        "Primary_Sys_Cmd" <- w2941
        "Valve_Bypass_Sys_Cmd" <- w2959
        "Valve_Vent_Sys_Cmd" <- w2958
        "Chiller_Sys_Cmd" <- w2942
        "Turbo_3_Motor_Sys_Cmd" <- w2946
        "Current Facility State" <- w2981
        "Target Facility State" <- w2980
        "Sub_state_iteration" <- w2979
        "Turbo_2_Motor_Sys_Cmd" <- w2949
        "Turbo 3 Standby?" <- w2945
        "Turbo 2 Standby?" <- w2947
      }
      frame #5 {
        n1079 = feedback #5() -> (w3058:bool[])  [unwired: 1 in]
        n1080 = feedback-in #5(w3064) -> ()
        n1081 = Not Equal?(x=w3058, y=w3064) -> (x != y?=w3031:bool[])
        n1082 = feedback #6() -> (w3030:bool[])  [unwired: 1 in]
        n1083 = Not Equal?(x=w3030, y=w3027) -> (x != y?=w3029:bool[])
        n1084 = feedback-in #6(w3027) -> ()
        n1085 = feedback #7() -> (w3060:bool)  [unwired: 1 in]
        n1086 = feedback-in #7(w3057) -> ()
        n1087 = feedback #8() -> (w3055:bool)  [unwired: 1 in]
        n1088 = feedback-in #8(w3051) -> ()
        n1089 = feedback #9() -> (w3063:bool)  [unwired: 1 in]
        n1090 = feedback-in #9(w3073) -> ()
        n1091 = Not Equal?(x=w3055, y=w3051) -> (x != y?=w3016:bool)
        n1092 = Not Equal?(x=w3060, y=w3057) -> (x != y?=w3059:bool)
        n1093 = for {
          shift-right: [w3129] -> w3061
          shift-left: w3056 -> [w3128]
          tunnel: w3029 -> [w3121] mode=indexing
          tunnel: w3027 -> [w3120] mode=indexing
          i -> [w3125]
          n1094 = Increment(x=w3125) -> (x+1=w3123:i32)
          n1095 = Number To Decimal String(number=w3123) -> (decimal integer string=w3124:string)  [unwired: 1 in]
          n1096 = Concatenate Strings(" Turbo " ("string"), w3124, " Valve at " ("string")) -> (w3122:string)
          n1097 = case shown="True" w3121 {
            tunnel: [w3132 w3141] -> w3129
            tunnel: "Opened" ("string") -> [_ w3138]
            tunnel: w3122 -> [_ w3137]
            tunnel: "Closed" ("f") -> [_ w3136]
            tunnel: w3128 -> [w3132 w3135]
            tunnel: w3120 -> [_ w3133]
            frame False {
            }
            frame True {
              n1098 = Get Date/Time String(want seconds? (F)=TRUE) -> (time string=w3140:string)  [unwired: 2 in, 1 out]
              n1099 = Select(t=w3138, s=w3133, f=w3136) -> (s? t:f=w3142:string)
              n1100 = Concatenate Strings(w3135, "\r", w3142, w3137, w3140) -> (w3141:string)
            }
          }
        }
        n1101 = feedback #10() -> (w3047:bool)  [unwired: 1 in]
        n1102 = feedback-in #10(w3046) -> ()
        n1103 = feedback #11() -> (w3021:bool)  [unwired: 1 in]
        n1104 = feedback-in #11(w3020) -> ()
        n1105 = Wait Until Next ms Multiple(millisecond multiple=u32 100 ("milliseconds to wait")) -> ()  [unwired: 1 out]
        n1106 = Not Equal?(x=w3063, y=w3073) -> (x != y?=w3062:bool)
        n1107 = feedback #12() -> (w3043:bool)  [unwired: 1 in]
        n1108 = feedback-in #12(w3040) -> ()
        n1109 = case shown="True" w3062 {
          tunnel: w3061 -> [w3187 w3193]
          tunnel: [w3187 w3195] -> w3066
          tunnel: w3073 -> [_ w3197]
          tunnel: "Opened" ("string") -> [_ w3191]
          tunnel: " Bypass Valve at " ("string") -> [_ w3190]
          tunnel: "Closed" ("f") -> [_ w3189]
          frame False {
          }
          frame True {
            n1110 = Select(t=w3191, s=w3197, f=w3189) -> (s? t:f=w3196:string)
            n1111 = Get Date/Time String(want seconds? (F)=TRUE) -> (time string=w3194:string)  [unwired: 2 in, 1 out]
            n1112 = Concatenate Strings(w3193, "\r", w3196, w3190, w3194) -> (w3195:string)
          }
        }
        n1113 = Not Equal?(x=w3047, y=w3046) -> (x != y?=w3017:bool)
        n1114 = case shown="True" w3059 {
          tunnel: w3066 -> [w3176 w3182]
          tunnel: [w3176 w3184] -> w3065
          tunnel: w3057 -> [_ w3186]
          tunnel: "Opened" ("string") -> [_ w3180]
          tunnel: " Vent Valve at " ("string") -> [_ w3179]
          tunnel: "Closed" ("f") -> [_ w3178]
          frame False {
          }
          frame True {
            n1115 = Get Date/Time String(want seconds? (F)=TRUE) -> (time string=w3183:string)  [unwired: 2 in, 1 out]
            n1116 = Select(t=w3180, s=w3186, f=w3178) -> (s? t:f=w3185:string)
            n1117 = Concatenate Strings(w3182, "\r", w3185, w3179, w3183) -> (w3184:string)
          }
        }
        n1118 = for {
          tunnel: w3064 -> [w3098] mode=indexing
          shift-right: [w3105] -> w3038
          shift-left: w3065 -> [w3106]
          tunnel: w3031 -> [w3097] mode=indexing
          i -> [w3104]
          n1119 = Increment(x=w3104) -> (x+1=w3103:i32)
          n1120 = Number To Decimal String(number=w3103) -> (decimal integer string=w3101:string)  [unwired: 1 in]
          n1121 = Concatenate Strings(" Gate Valve " ("string"), w3101, " at " ("string")) -> (w3099:string)
          n1122 = case shown="True" w3097 {
            tunnel: w3106 -> [w3109 w3116]
            tunnel: [w3109 w3118] -> w3105
            tunnel: w3098 -> [_ w3110]
            tunnel: "Opened" ("string") -> [_ w3114]
            tunnel: w3099 -> [_ w3113]
            tunnel: "Closed" ("f") -> [_ w3112]
            frame False {
            }
            frame True {
              n1123 = Select(t=w3114, s=w3110, f=w3112) -> (s? t:f=w3119:string)
              n1124 = Get Date/Time String(want seconds? (F)=TRUE) -> (time string=w3117:string)  [unwired: 2 in, 1 out]
              n1125 = Concatenate Strings(w3116, "\r", w3119, w3113, w3117) -> (w3118:string)
            }
          }
        }
        n1126 = case shown="True" w3016 {
          tunnel: w3038 -> [w3165 w3168]
          tunnel: [w3165 w3174] -> w3045
          tunnel: w3051 -> [_ w3166]
          tunnel: "Started" ("string") -> [_ w3171]
          tunnel: " Primary Pump at " ("string") -> [_ w3170]
          tunnel: "Stopped" ("f") -> [_ w3169]
          frame False {
          }
          frame True {
            n1127 = Select(t=w3171, s=w3166, f=w3169) -> (s? t:f=w3175:string)
            n1128 = Get Date/Time String(want seconds? (F)=TRUE) -> (time string=w3173:string)  [unwired: 2 in, 1 out]
            n1129 = Concatenate Strings(w3168, "\r", w3175, w3170, w3173) -> (w3174:string)
          }
        }
        n1130 = Not Equal?(x=w3021, y=w3020) -> (x != y?=w3022:bool)
        n1131 = Not Equal?(x=w3043, y=w3040) -> (x != y?=w3044:bool)
        n1132 = case shown="True" w3017 {
          tunnel: w3045 -> [w3154 w3158]
          tunnel: [w3154 w3157] -> w3019
          tunnel: w3046 -> [_ w3155]
          tunnel: "Started" ("string") -> [_ w3161]
          tunnel: " Chiller at " ("string") -> [_ w3160]
          tunnel: "Stopped" ("f") -> [_ w3159]
          frame False {
          }
          frame True {
            n1133 = Select(t=w3161, s=w3155, f=w3159) -> (s? t:f=w3164:string)
            n1134 = Get Date/Time String(want seconds? (F)=TRUE) -> (time string=w3163:string)  [unwired: 2 in, 1 out]
            n1135 = Concatenate Strings(w3158, "\r", w3164, w3160, w3163) -> (w3157:string)
          }
        }
        n1136 = case shown="True" w3022 {
          tunnel: "Started" ("string") -> [_ w3093]
          tunnel: " Turbo Pump 2 at " ("string") -> [_ w3092]
          tunnel: "Stopped" ("f") -> [_ w3091]
          tunnel: w3020 -> [_ w3089]
          tunnel: w3019 -> [w3086 w3088]
          tunnel: [w3086 w3087] -> w3018
          frame False {
          }
          frame True {
            n1137 = Select(t=w3093, s=w3089, f=w3091) -> (s? t:f=w3096:string)
            n1138 = Get Date/Time String(want seconds? (F)=TRUE) -> (time string=w3095:string)  [unwired: 2 in, 1 out]
            n1139 = Concatenate Strings(w3088, "\r", w3096, w3092, w3095) -> (w3087:string)
          }
        }
        n1140 = case shown="True" w3044 {
          tunnel: w3018 -> [w3143 w3145]
          tunnel: [w3143 w3151] -> w3026
          tunnel: w3040 -> [_ w3153]
          tunnel: "Started" ("string") -> [_ w3148]
          tunnel: " Turbo Pump 3 at " ("string") -> [_ w3147]
          tunnel: "Stopped" ("f") -> [_ w3146]
          frame False {
          }
          frame True {
            n1141 = Select(t=w3148, s=w3153, f=w3146) -> (s? t:f=w3152:string)
            n1142 = Get Date/Time String(want seconds? (F)=TRUE) -> (time string=w3150:string)  [unwired: 2 in, 1 out]
            n1143 = Concatenate Strings(w3145, "\r", w3152, w3147, w3150) -> (w3151:string)
          }
        }
        "Log" <- w3026
      }
    }
    n1144 = Not(x=w842) -> (.not. x?=w841:bool)
    n1145 = feedback-in #13(w718) -> ()
    n1146 = feedback #13() -> (w717:string)  [unwired: 1 in]
    n1147 = Search and Replace String(input string=w718, search string=w717) -> (result string=→"New log":string)  [unwired: 6 in, 3 out]
    "Running" <- w842
  }
  n1148 = call <vilib>:"DAQmx Stop Task.vi"("task/channels in"=w161, "error in"=w160) -> ("task out"=w163:refnum<k21>, "error out"=w162:errorcluster)  [unwired: 12 in]
  n1149 = call <vilib>:"DAQmx Clear Task.vi"("task in"=w163, "error in"=w162) -> ()  [unwired: 13 in, 1 out]
  n1150 = node-c288(w45) -> ()  [unwired: 1 out]
  n1151 = case shown="True" w201 {
    tunnel: w226 -> [w3199 w3203]
    tunnel: [w3199 w3201] -> w224
    tunnel: [errorcluster {"status"=FALSE, "code"=0, "source"=""} ("error out") w3200] -> w223
    frame False {
    }
    frame True {
      n1152 = call-poly <vilib>:"DAQmx Write.vi"("task/channels in"=w3203, "data"=FALSE) -> ("task out"=w3201:refnum<k21>, "error out"=w3200:errorcluster)  [unwired: 11 in, 1 out]
    }
  }
  n1153 = case shown="True" w201 {
    tunnel: w291 -> [w3205 w3209]
    tunnel: [w3205 w3208] -> w290
    tunnel: [errorcluster {"status"=FALSE, "code"=0, "source"=""} ("error out") w3207] -> w289
    frame False {
    }
    frame True {
      n1154 = call-poly <vilib>:"DAQmx Write.vi"("task/channels in"=w3209, "data"=bool[] [FALSE, FALSE, FALSE, FALSE, FALSE, FALSE, FALSE, FALSE]) -> ("task out"=w3208:refnum<k21>, "error out"=w3207:errorcluster)  [unwired: 11 in, 1 out]
    }
  }
  n1155 = case shown="True" w201 {
    tunnel: w288 -> [w3211 w3215]
    tunnel: [w3211 w3214] -> w287
    tunnel: [errorcluster {"status"=FALSE, "code"=0, "source"=""} ("error out") w3212] -> w286
    frame False {
    }
    frame True {
      n1156 = call-poly <vilib>:"DAQmx Write.vi"("task/channels in"=w3215, "data"=FALSE) -> ("task out"=w3214:refnum<k21>, "error out"=w3212:errorcluster)  [unwired: 11 in, 1 out]
    }
  }
  n1157 = case shown="True" w166 {
    tunnel: w167 -> [_ w3217]
    tunnel: w168 -> [_ w3216]
    frame False {
    }
    frame True {
      n1158 = call <instrlib>:"Close.vi"("error in (no error)"=w3217, "VISA resource name"=w3216) -> ()  [unwired: 9 in, 1 out]
    }
  }
  n1159 = call <vilib>:"DAQmx Stop Task.vi"("task/channels in"=w224, "error in"=w223) -> ("task out"=w222:refnum<k21>, "error out"=w225:errorcluster)  [unwired: 12 in]
  n1160 = case shown="True" w201 {
    tunnel: w211 -> [w3218 w3223]
    tunnel: [w3218 w3222] -> w65
    tunnel: [errorcluster {"status"=FALSE, "code"=0, "source"=""} ("error out") w3221] -> w64
    frame False {
    }
    frame True {
      n1161 = call-poly <vilib>:"DAQmx Write.vi"("task/channels in"=w3223, "data"=bool[] [FALSE, FALSE, FALSE, FALSE, FALSE, FALSE, FALSE, FALSE] ("appended array")) -> ("task out"=w3222:refnum<k21>, "error out"=w3221:errorcluster)  [unwired: 11 in, 1 out]
    }
  }
  n1162 = call <vilib>:"DAQmx Stop Task.vi"("task/channels in"=w313) -> ("task out"=w315:refnum<k21>, "error out"=w316:errorcluster)  [unwired: 13 in]
  n1163 = call <vilib>:"DAQmx Stop Task.vi"("task/channels in"=w290, "error in"=w289) -> ("task out"=w292:refnum<k21>, "error out"=w293:errorcluster)  [unwired: 12 in]
  n1164 = call <vilib>:"DAQmx Stop Task.vi"("task/channels in"=w314) -> ("task out"=w338:refnum<k21>, "error out"=w336:errorcluster)  [unwired: 13 in]
  n1165 = call <vilib>:"DAQmx Stop Task.vi"("task/channels in"=w287, "error in"=w286) -> ("task out"=w347:refnum<k21>, "error out"=w337:errorcluster)  [unwired: 12 in]
  n1166 = call <vilib>:"DAQmx Stop Task.vi"("task/channels in"=w244) -> ("task out"=w245:refnum<k21>, "error out"=w246:errorcluster)  [unwired: 13 in]
  n1167 = call <vilib>:"DAQmx Stop Task.vi"("task/channels in"=w261) -> ("task out"=w260:refnum<k21>, "error out"=w257:errorcluster)  [unwired: 13 in]
  n1168 = call <vilib>:"DAQmx Stop Task.vi"("task/channels in"=w214) -> ("task out"=w73:refnum<k21>, "error out"=w72:errorcluster)  [unwired: 13 in]
  n1169 = call <vilib>:"DAQmx Stop Task.vi"("task/channels in"=w213) -> ("task out"=w70:refnum<k21>, "error out"=w71:errorcluster)  [unwired: 13 in]
  n1170 = call <vilib>:"DAQmx Clear Task.vi"("task in"=w222, "error in"=w225) -> ("error out"=w218:errorcluster)  [unwired: 13 in]
  n1171 = call <vilib>:"DAQmx Clear Task.vi"("task in"=w315, "error in"=w316) -> ("error out"=w285:errorcluster)  [unwired: 13 in]
  n1172 = call <vilib>:"DAQmx Clear Task.vi"("task in"=w292, "error in"=w293) -> ("error out"=w282:errorcluster)  [unwired: 13 in]
  n1173 = call <vilib>:"DAQmx Clear Task.vi"("task in"=w338, "error in"=w336) -> ("error out"=w284:errorcluster)  [unwired: 13 in]
  n1174 = call <vilib>:"DAQmx Clear Task.vi"("task in"=w347, "error in"=w337) -> ("error out"=w259:errorcluster)  [unwired: 13 in]
  n1175 = call <vilib>:"DAQmx Clear Task.vi"("task in"=w245, "error in"=w246) -> ("error out"=w221:errorcluster)  [unwired: 13 in]
  n1176 = call <vilib>:"DAQmx Clear Task.vi"("task in"=w260, "error in"=w257) -> ("error out"=w243:errorcluster)  [unwired: 13 in]
  n1177 = call <vilib>:"DAQmx Clear Task.vi"("task in"=w73, "error in"=w72) -> ("error out"=w69:errorcluster)  [unwired: 13 in]
  n1178 = call <vilib>:"DAQmx Clear Task.vi"("task in"=w70, "error in"=w71) -> ("error out"=w68:errorcluster)  [unwired: 13 in]
  n1179 = call <vilib>:"DAQmx Stop Task.vi"("task/channels in"=w65, "error in"=w64) -> ("task out"=w67:refnum<k21>, "error out"=w66:errorcluster)  [unwired: 12 in]
  n1180 = call <vilib>:"DAQmx Clear Task.vi"("task in"=w67, "error in"=w66) -> ("error out"=w63:errorcluster)  [unwired: 13 in]
  n1181 = Merge Errors(w63) -> (w48:errorcluster)
  n1182 = Merge Errors(w69, w68, w48) -> (w217:errorcluster)
  n1183 = Merge Errors(w217) -> (w216:errorcluster)
  n1184 = Merge Errors(w218, w216) -> (w219:errorcluster)
  n1185 = Merge Errors(w221, w219) -> (w220:errorcluster)
  n1186 = Merge Errors(w243, w220) -> (w242:errorcluster)
  n1187 = Merge Errors(w259, w242) -> (w258:errorcluster)
  n1188 = Merge Errors(w284, w258) -> (w283:errorcluster)
  n1189 = Merge Errors(w282, w283) -> (w281:errorcluster)
  n1190 = Merge Errors(w285, w281) -> ()  [unwired: 1 out]
  "DAQ_Name" <- w41
  "Use_real_Values?" <- "Use fake values?"
  "Use Ecodry As Primary?" <- FALSE
